vi "COD主界面（列队使用）.vi"() -> (8 "多列列表框":i32(listbox))   [LabVIEW 2016, in "斯坦道CODMn.lvlib"]
uses:
  <vilib>/Utility/miscctls.llb/LVPointTypeDef.ctl
  <vilib>/Analysis/6fits.llb/Curve Fitting Criteria.ctl
  <vilib>/Plasmionique/MB Master/MB_Master_Serial/MB_Master_Serial.lvclass
  D:/Program Files (x86)/National Instruments/LabVIEW 2016/vi.lib/Plasmionique/MB Master/MB_Master/MB_Master.lvclass
  <vilib>/Utility/config.llb/Write Key (Double).vi
  <vilib>/Utility/config.llb/Read Key (I32).vi
  <vilib>/Utility/config.llb/Read Key (Double).vi
  <vilib>/Utility/config.llb/Read Key (Boolean).vi
  <vilib>/Utility/config.llb/Write Key (Boolean).vi
  <vilib>/Utility/config.llb/Write Key (I32).vi
  <vilib>/Waveform/WDTFileIO.llb/Read Waveform from File.vi
  <vilib>/Plasmionique/MB Master/MB Master.lvlib
  <vilib>/ptbypt/NI_PtbyPt.lvlib
  <vilib>/Utility/config.llb/NI_LVConfig.lvlib
  <vilib>/Analysis/NI_AALPro.lvlib
panel:
  out "ORP-K":string
  out "ORP-B":string
  out "ORP-A":string
  out "x = y?":bool
  out "稀释倍数解释":string
  in  "CODMn跨度量程选择":enum32{"H", "L", "AUTO"}(ring)=enum."AUTO"
  in  "跨度液浓度":dbl
  in  "水样":dbl
  in  "蒸馏水":dbl
  in  "标液":dbl
  in  "质控样":dbl
  in  "加标回收":dbl
  in  "草酸钠":dbl
  in  "高锰酸钾":dbl
  in  "硫酸":dbl
  out "量程解释说明":string
  in  "高切低阈值:":dbl
  in  "低切高阈值:":dbl
  in  "自动切换量程:":enum16{"关闭", "自动切换测一次", "自动切换测两次"}(ring)
  in  "修正系数":dbl
  in  "标准液浓度":dbl
  in  "温度":dbl
  in  "恒温时间":dbl
  in  "基本量程":enum16{"L", "H"}(ring)
  in  "CODMn零点核查选择":enum16{"零点核查走纯水管", "零点核查走质控管"}(ring)
  in  "锁定按钮":bool
  in  "低量程稀释倍数:":i8=1
  out "切换量程连续测两次":bool
  in  "高量程稀释倍数:":i8=2
  in  "一键写入":bool
  in  "测量模式(公式)":u16(ring)=1 items=["水样测试"=1, "标样核查"=2, "零点核查"=3, "跨度核查"=4, "空白测试"=5, "平行样"=6, "加标回收"=7]
  out "基本量程(显示)":string
  out "测量模式(显示)":string
  in  "量程切换次数":u8
  out "数据时间":string
  out "断电排液标记":bool
  in  "测量模式":T1(ring)
  out "COM":string
  in  "启用5":bool
  in  "校准5":bool
  in  "泵滴定数5":dbl
  in  "浓度5":dbl
  in  "启用4":bool
  in  "校准4":bool
  in  "泵滴定数4":dbl
  in  "浓度4":dbl
  out "波形时间":timestamp
  in  "历史波形":bool
  out "滴定数-ORP值":u16[](array[numeric]) caption="数组"
  in  "关闭 3":bool
  in  "滴定曲线":bool
  out "ORP滴定曲线":u16[](graph)
  out "空白测试标记":bool
  out "跨度核查标记":bool
  out "启动选择 2":u16(ring) items=["水样测试", "标样核查", "零点核查", "跨度核查", "空白测试", "加标回收", "平行样", "校零", "校标"]
  in  "量程选择":enum16{"低量程", "高量程", "0-2量程"}(ring)
  in  "手动控制":bool
  in  "选用水样":enum16{"葡萄糖", "草酸钠"}(ring)
  in  "方程系数":cluster{"X":dbl, "b":dbl, "X^2":dbl} {"X^2" format="%#.6g"; "b" format="%#.6g"; "X" format="%#.6g"}
  out "多项式系数1":dbl[](array[numeric]) caption="多项式系数"
  out "XY图":cluster{"X Values":dbl[], "Y Values":dbl[]}[](graph)
  in  "模型":enum32{"线性", "多项式"}(ring)
  out "启动时间":timestamp format="%<%Y/%m/%d %H:%M:%S>T"
  in  "24H周期设置":bool[](xcontrol)
  in  "关闭 2":bool
  in  "周期设置":bool
  out "文本.文本":string
  out "r^2":dbl format="%.8g"
  out "拟合公式":string
  out "b":dbl format="%#.4g"
  out "K":dbl format="%#.4f"
  out "当前校准":i32
  in  "启用3":bool
  in  "启用2":bool
  in  "启用1":bool
  in  "校准3":bool
  in  "校准2":bool
  in  "校准1":bool
  in  "泵滴定数3":dbl
  in  "泵滴定数2":dbl
  in  "泵滴定数1":dbl
  in  "浓度3":dbl
  in  "浓度2":dbl
  in  "浓度1":dbl
  in  "写入":bool
  out "测量模式数字":i32
  out "零点核查标记":bool
  out "排液故障":bool
  out "进水样超量程":bool
  out "标样核查标记":bool
  out "平行样测量":bool
  out "加标回收测量":bool
  out "质控样测量":bool
  out "待机":bool
  out "校标错误":bool
  out "校零错误":bool
  out "测量错误":bool
  out "草酸钠报警":bool
  out "高锰酸钾报警":bool
  out "加热故障":bool
  out "温控器故障":bool
  out "ORP故障":bool
  out "排液标记":bool
  out "故障标记":bool
  out "校标标记":bool
  out "校零标记":bool
  out "通讯状态":bool
  out "水样测量":bool
  out "读取KB值":bool
  in  "读取":bool
  in  "返回":bool
  in  "校准配置":bool
  in  "零点泵计量数 2":dbl
  in  "标度泵计量数 2":dbl
  out "标度滴定值":dbl
  out "零点滴定值":dbl
  in  "保存":bool
  in  "关闭":bool
  out "测量数据区":T2 {"单位" items=["ug/L", "mg/L", "ppm", "mg/m3", "cm", "ppb", "ug/m3", "%", "nmol/mol", "umol/mol", "MPN/L", "MPN/100ml", "ng/m3", "NTU", "无量纲", "ms/cm", "us/cm", "℃", "mV", "万个/L"]}
  out "仪器时间":timestamp format="%<%Y/%m/%d %H:%M:%S>T"
  out "秒":u16
  out "分":u16
  out "COD浓度（mg/L)":dbl format="%.2g"
  out "进样管":dbl
  out "高锰酸钾":dbl
  out "草酸钠":dbl
  out "硫酸":dbl
  out "ORP显示":dbl
  out "温度":dbl
  out "加热":bool
  out "搅拌":bool
  out "进硫酸":bool
  out "进加标回收样":bool
  out "进质控样":bool
  out "进标液":bool
  out "进蒸馏水":bool
  out "进水样":bool
  out "进草酸钠":bool
  out "进高锰酸钾":bool
  out "定时启动":bool
  in  "启动":bool
  in  "故障清除":bool
  in  "参数配置":bool
  in  "停止":bool
  in  "单步启动":bool
  out "系统时间":timestamp
  in  "时间校准":bool
  in  "枚举":enum16{"读取数据", "写入数据", "读取写入DATABASE", "读取参数"}(ring)
  out "报警簇":T3
  out "Registers":u16[](array[numeric])
  in  "Slave ID":u8=1
  in  "Serial Config":T4={"baud rate (bps)"=115200, "stop bits"=10, "parity"=0, "flow control"=0, "timeout"=1000, "retries"=1} {"stop bits" items=["1.0"=10, "1.5"=15, "2.0"=20]; "flow control" items=["None", "XON/XOFF", "RTS/CTS", "XON/XOFF & RTS/CTS", "DTR/DSR", "XON/XOFF & DTR/DSR"]; "parity" items=["None", "Odd", "Even", "Mark", "Space"]}
  out "模式（受控）":u16
  in  "VISA resource name":refnum<visa-resource-name>="COM4" caption="VISA资源名称"
  # "测量时间："
  # "(水样~加标回收)"
  # "mV"
  # "℃"
  # "注：遇到加热故障和排液故障时仪器不能正常启动，\n必须排查故障并点击报警清除按钮方可运行。"
  # "mg/L"
  # "泵计量参数设置"
  # "基本参数设置"
  # "校零校标结果"
  # "校零结果："
  # "校零滴定值："
  # "加热恒温温度(℃):"
  # "水样："
  # "高锰酸钾："
  # "校标结果："
  # "标度滴定值："
  # "恒温时间(分钟):"
  # "草酸钠："
  # "蒸馏水："
  # "零点泵计量值："
  # "标准液浓度(mg/L):"
  # "硫酸："
  # "标液："
  # "标度泵计量值："
  # "修正系数："
  # "跨度液浓度："
  # "质控样:"
  # "基本量程(L、H)可选:"
  # "跨度量程选择："
  # "加标回收样："
  # "是否启用"
  # "泵滴定数"
  # "浓度"
  # "辅\n助\n计\n算\n区"
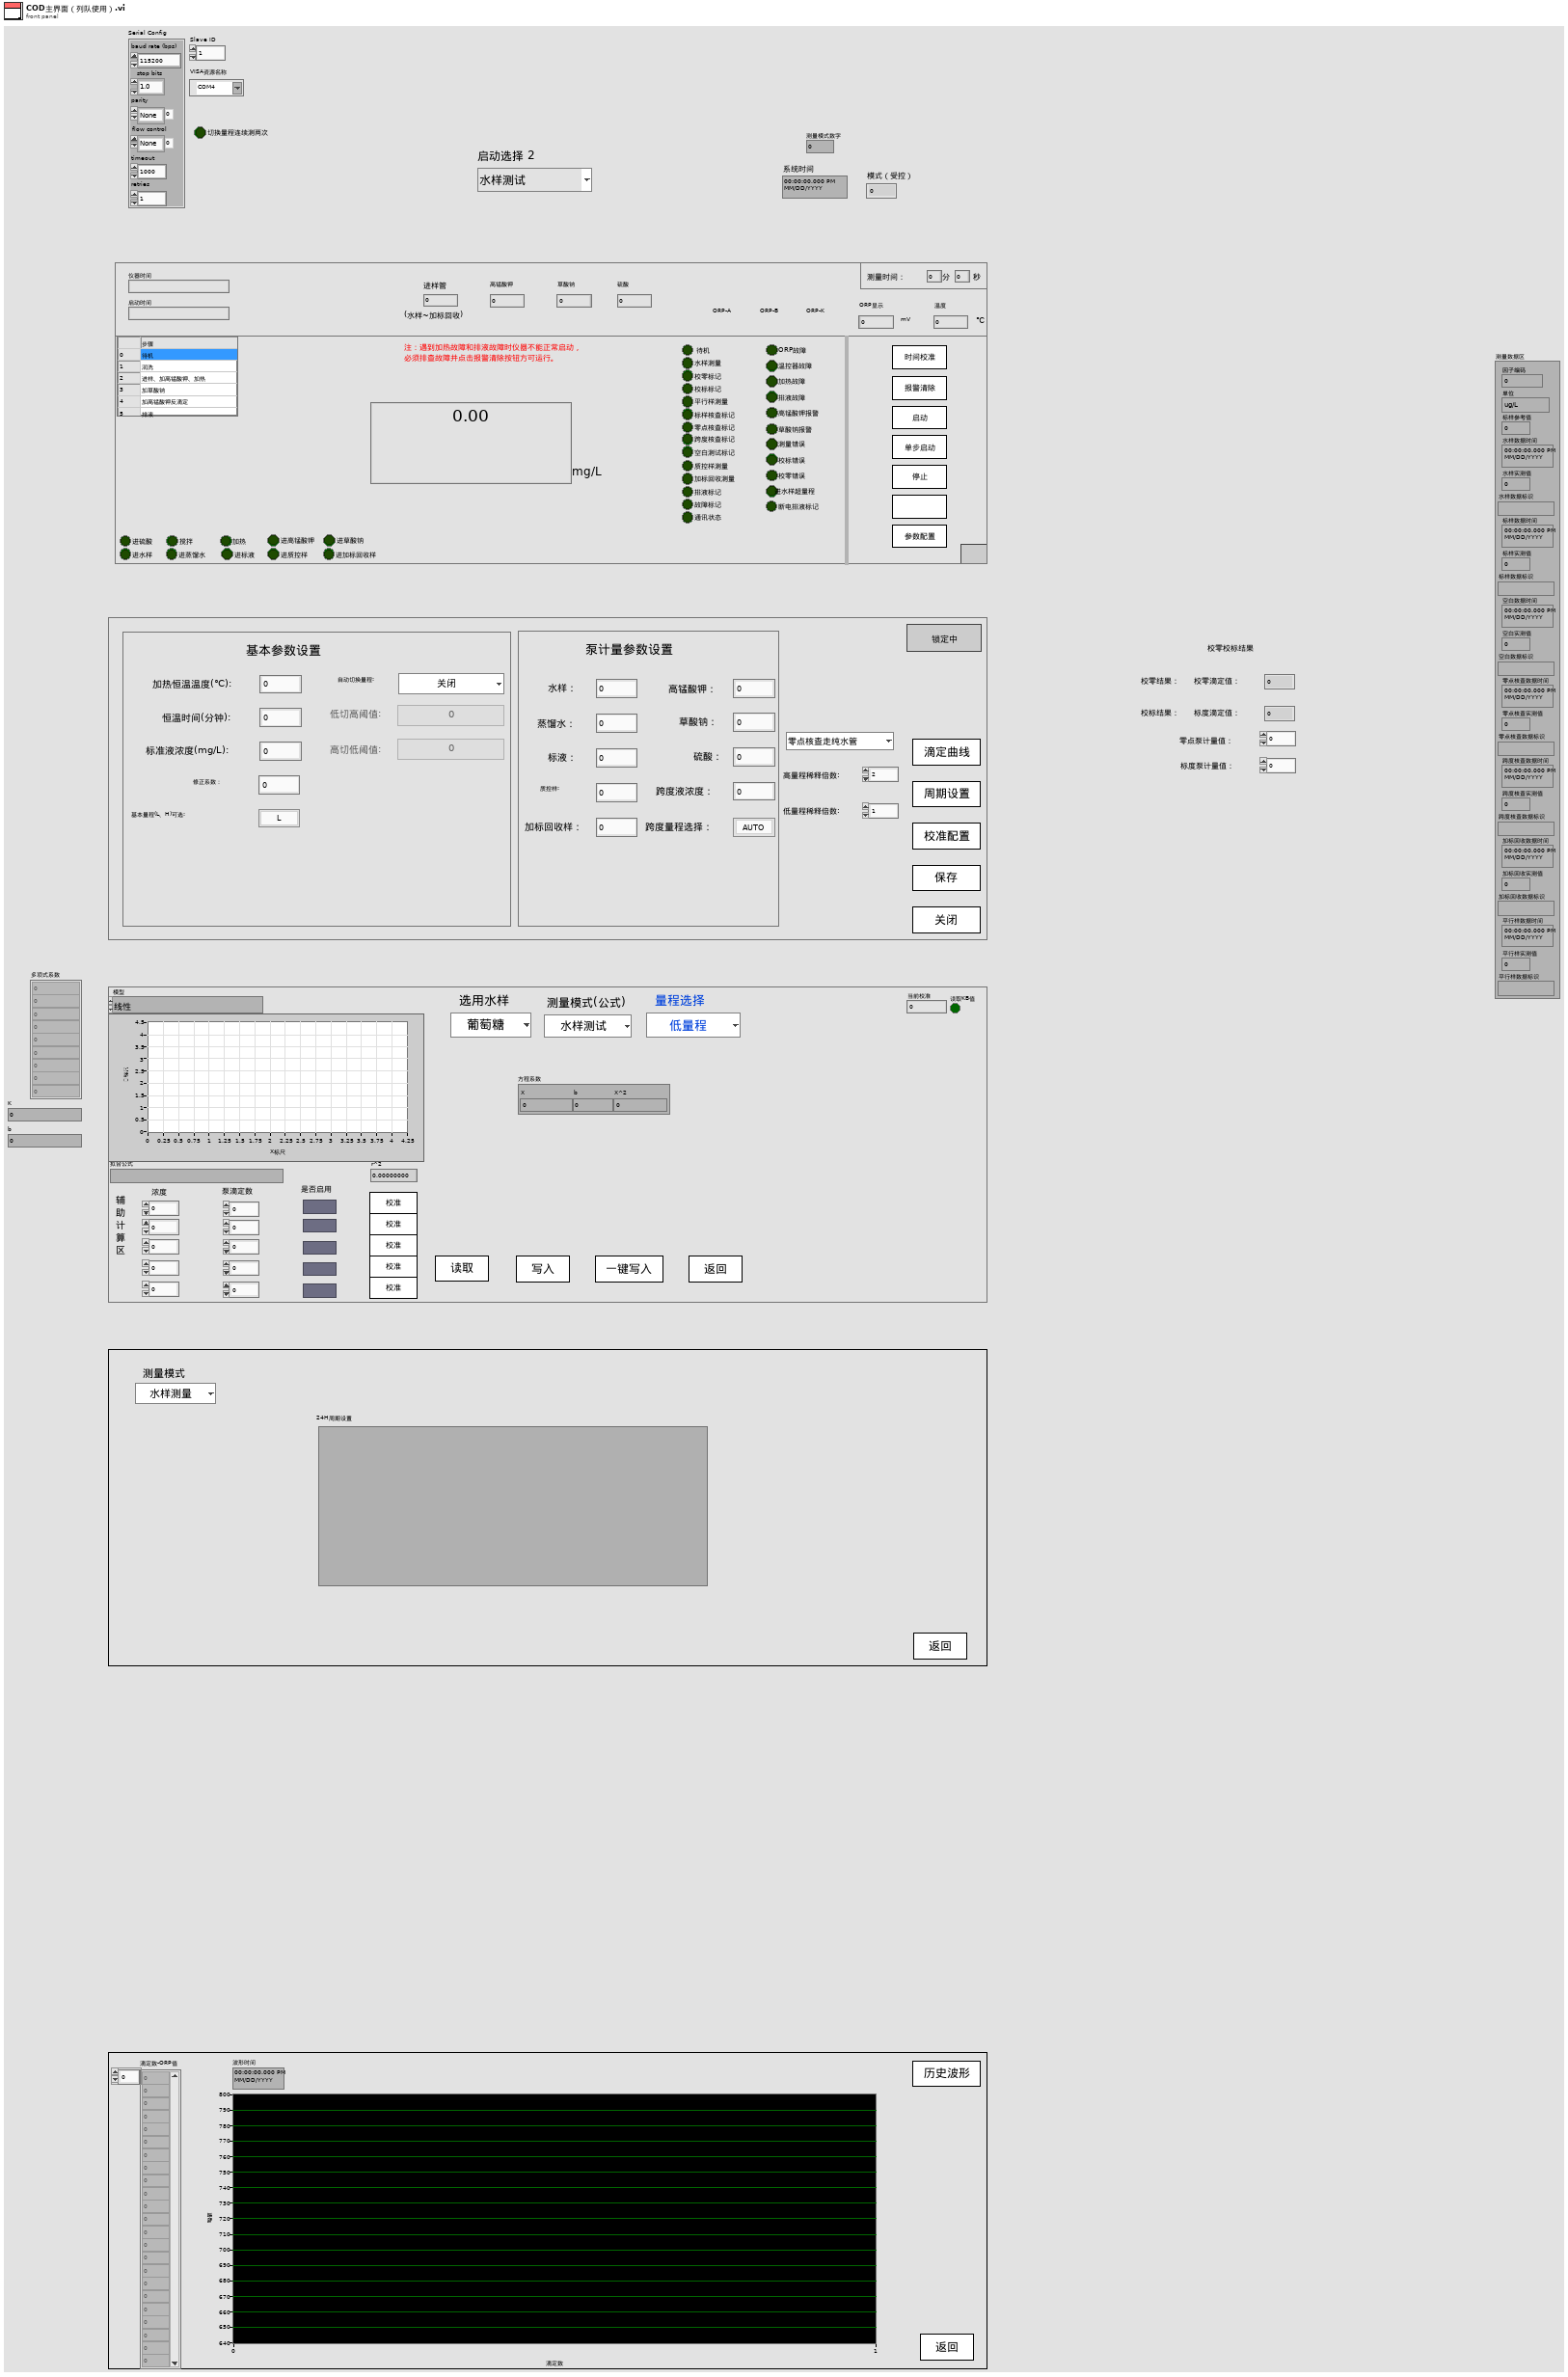
[diagram p1: front panel]
types:
  T1 = enum16{"水样测量", "标样核查", "零点核查", "跨度核查", "空白测试", "加标回收", "平行样", "校零", "校标"}
  T2 = cluster{"因子编码":u32, "单位":u16, "标样参考值":sgl, "水样数据时间":timestamp, "水样实测值":sgl, "水样数据标识":string, "标样数据时间":timestamp, "标样实测值":sgl, "标样数据标识":string, "空白数据时间":timestamp, "空白实测值":sgl, "空白数据标识":string, "零点核查数据时间":timestamp, "零点核查实测值":sgl, "零点核查数据标识":string, "跨度核查数据时间":timestamp, "跨度核查实测值":sgl, "跨度核查数据标识":string, "加标回收数据时间":timestamp, "加标回收实测值":sgl, "加标回收数据标识":string, "平行样数据时间":timestamp, "平行样实测值":sgl, "平行样数据标识":string}
  T3 = cluster{"ORP故障":bool, "温控器故障":bool, "加热故障":bool, "高锰酸钾报警":bool, "草酸钠报警":bool, "测量错误":bool, "校零错误":bool, "校标错误":bool, " 进水样超量程":bool, "排液阀故障":bool}
  T4 = cluster{"baud rate (bps)":u32, "stop bits":u16, "parity":u16, "flow control":u16, "timeout":u32, "retries":i32}
  T5 = cluster{"starting address":u16, "number of holding registers":u16}
  T6 = typedef "NI_LVConfig.lvlib/Config Data RefNum.ctl" = refnum<k1>
  T7 = cluster{"测量模式":enum16{"水样测量", "标样核查", "零点核查", "跨度核查", "空白测试", "加标回收", "平行样", "校零", "校标"}}
  T8 = cluster{"仪器测试类型":enum16{"水样测试", "标样核查", "空白测试", "跨度核查"}, "周期设置类型":enum16{"定点启动", "间隔启动"}, "定时功能启用":bool, "定时间隔":dbl, "24H周期设置":bool[]}
  T9 = typedef "LVDateTimeRec.ctl" = cluster{"秒数的小数部分":dbl, "秒":i32, "分":i32, "时":i32, "日":i32, "月":i32, "年":i32, "天数（周）":i32, "天数（年）":i32, "DST":i32}
  T10 = enum8{"Enabled", "Disabled", "Disabled and Grayed Out"}
  T11 = typedef "NI_AALPro.lvlib/Curve Fitting Criteria.ctl" = u16
  T12 = cluster{"时间":timestamp, "测量模式":string, "数据类型":string, "检测值":sgl, "单位":string, "数据标识":string, "因子编码":string, "标样参考值":sgl, "ORP-A":sgl, "ORP-B":sgl, "ORP-K":sgl, "COD滴定值":sgl, "高锰酸钾滴定数":sgl, "温度":sgl, "量程":sgl}
  T13 = typedef "LVPointTypeDef.ctl" = cluster{"Horizontal":i16, "Vertical":i16}
  T14 = cluster{"时间标识":timestamp, "参数":string, "日志信息":string, "流程参数":string}
  T15 = cluster{"时间标识":timestamp, "设备":string, "日志信息":string}
  T16 = cluster{"时间标识":timestamp, "设备":string, "日志信息":string, "流程参数":string}
  T17 = cluster{"运行模式":enum16{"维护模式", "常规模式", "应急模式", "质控模式"}}
  T18 = cluster{"数组 2[0]":sgl, "数组 2[1]":sgl, "数组 2[2]":sgl, "数组 2[3]":sgl, "数组 2[4]":sgl, "数组 2[5]":sgl, "数组 2[6]":sgl, "数组 2[7]":sgl, "数组 2[8]":sgl, "数组 2[9]":sgl, "数组 2[10]":sgl, "数组 2[11]":sgl, "数组 2[12]":sgl, "数组 2[13]":sgl, "数组 2[14]":sgl, "数组 2[15]":sgl, "数组 2[16]":sgl, "数组 2[17]":sgl, "数组 2[18]":sgl, "数组 2[19]":sgl, "数组 2[20]":sgl, "数组 2[21]":sgl, "数组 2[22]":sgl, "数组 2[23]":sgl, "数组 2[24]":sgl, "数组 2[25]":sgl, "数组 2[26]":sgl, "数组 2[27]":sgl, "数组 2[28]":sgl, "数组 2[29]":sgl, "数组 2[30]":sgl, "数组 2[31]":sgl, "数组 2[32]":sgl, "数组 2[33]":sgl, "数组 2[34]":sgl, "数组 2[35]":sgl, "数组 2[36]":sgl, "数组 2[37]":sgl, "数组 2[38]":sgl, "数组 2[39]":sgl, "数组 2[40]":sgl, "数组 2[41]":sgl}
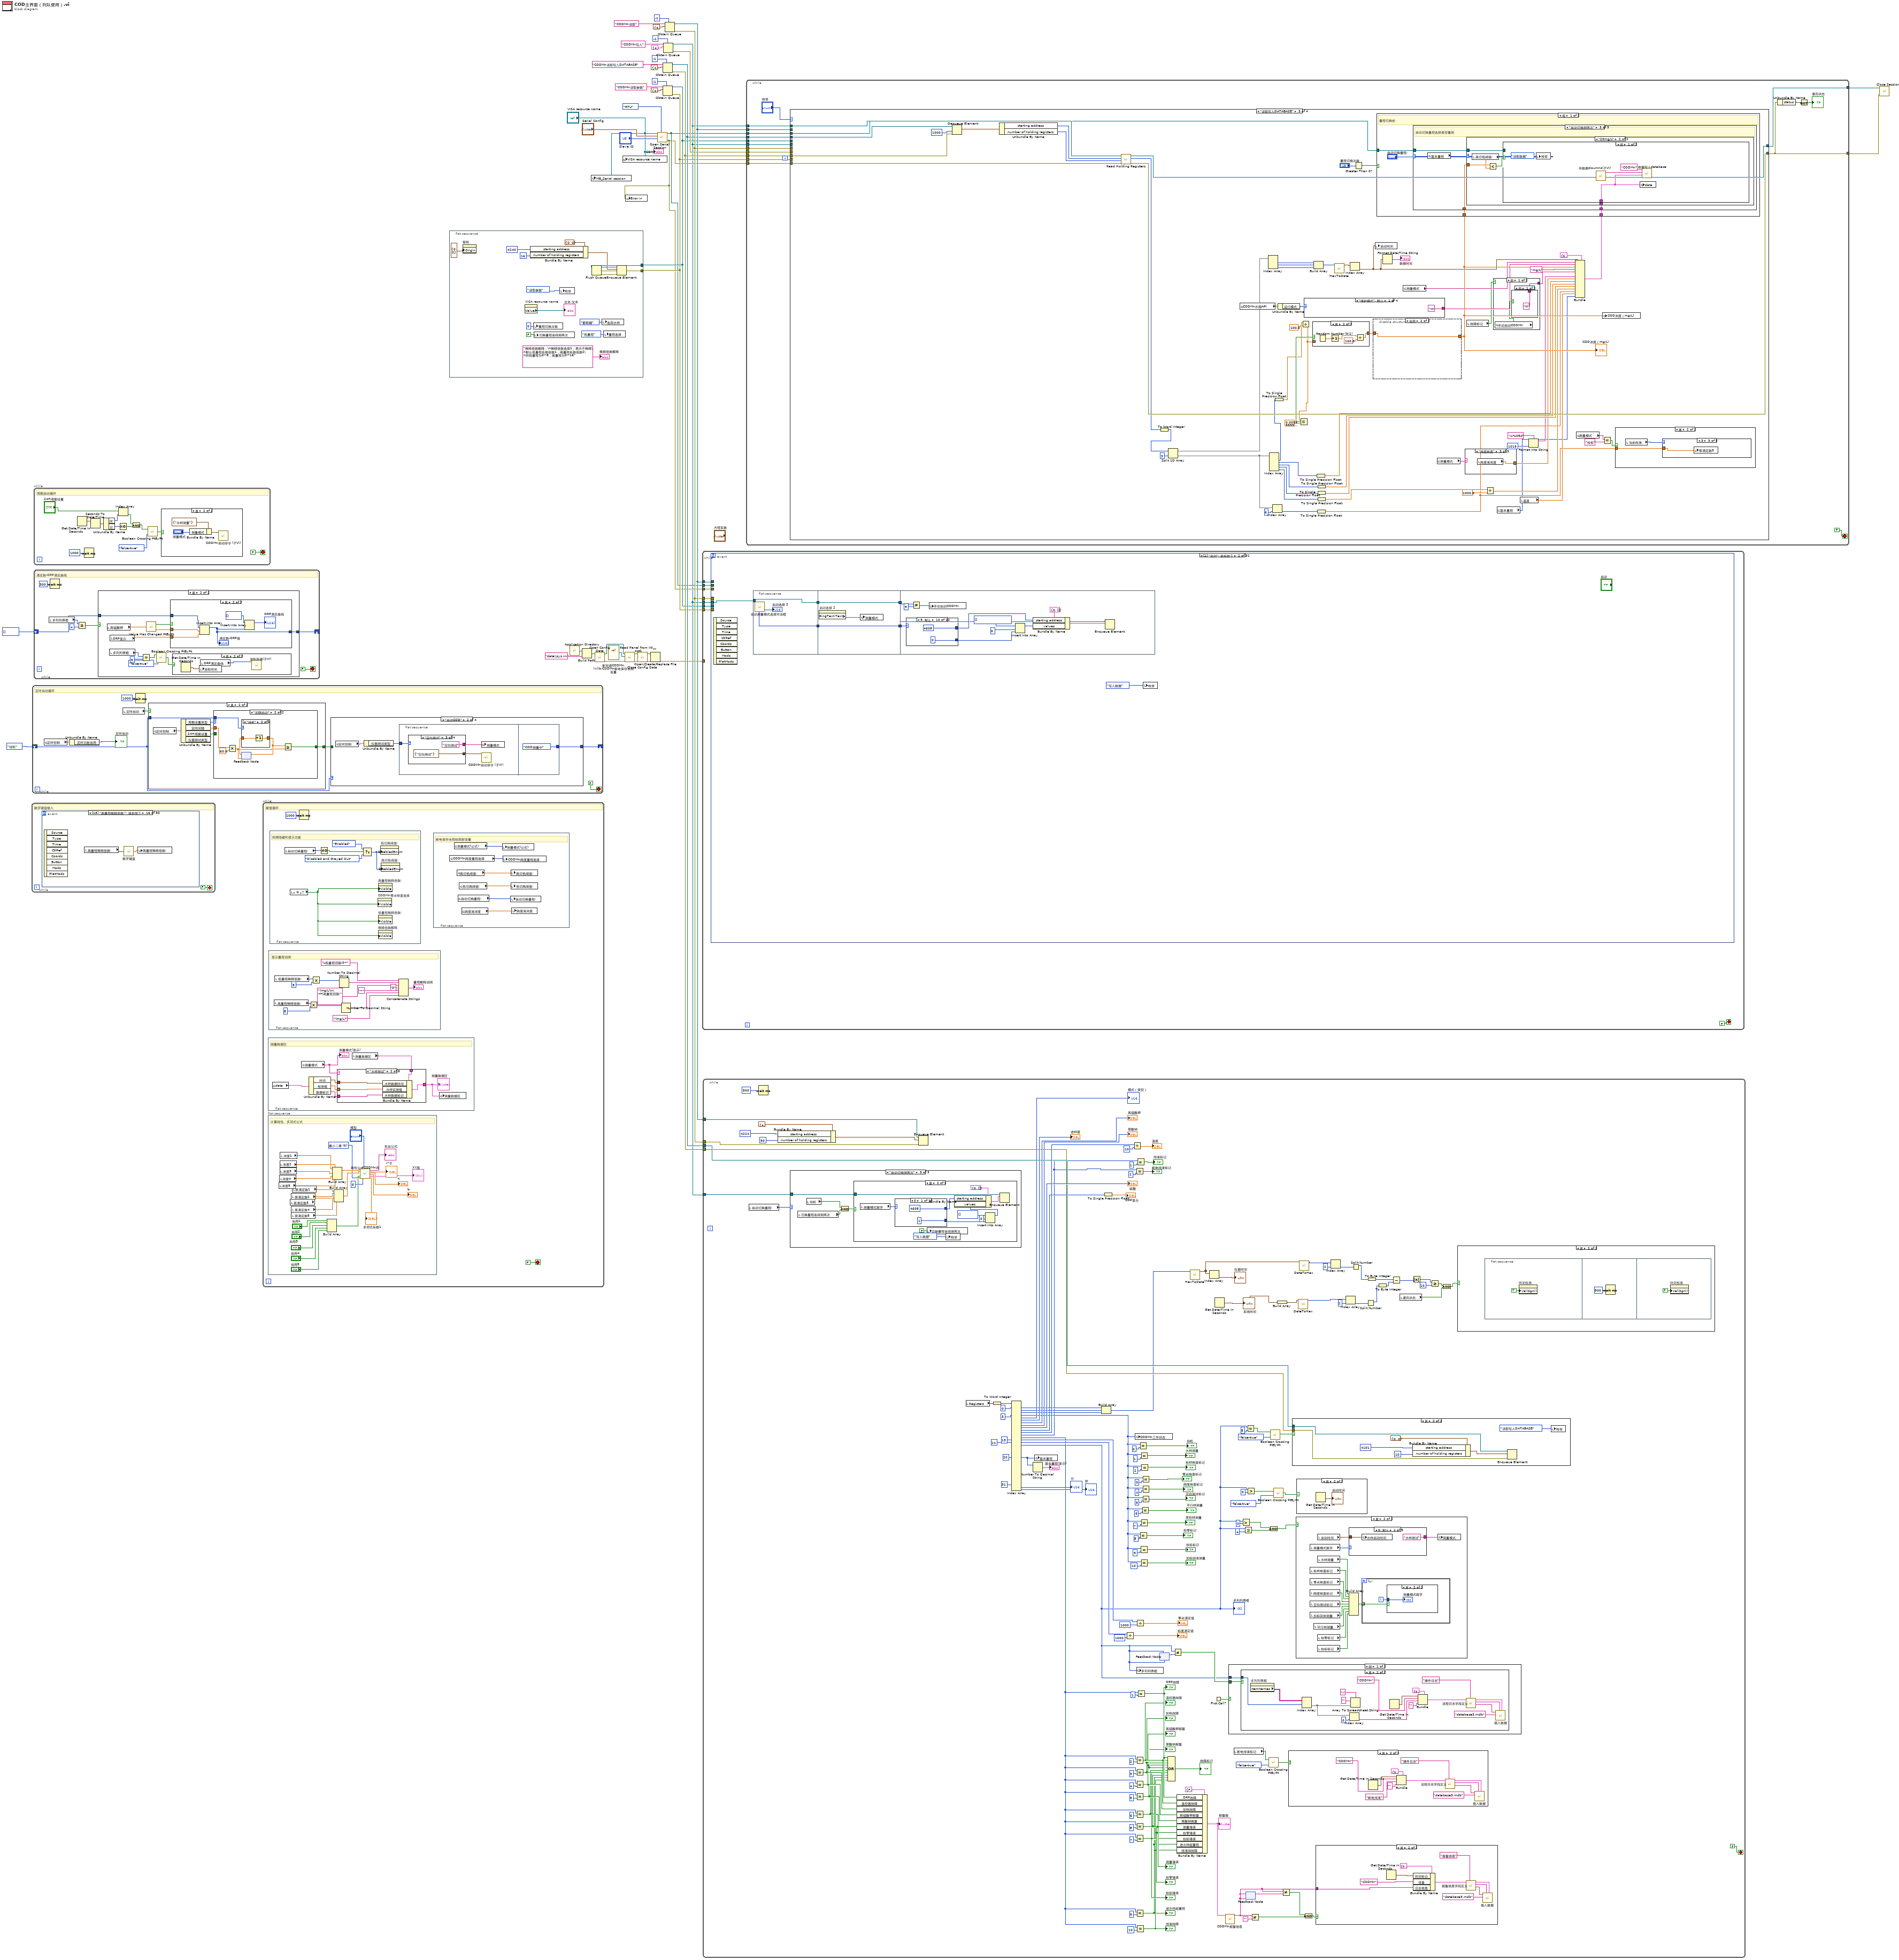
[diagram p0: block diagram]
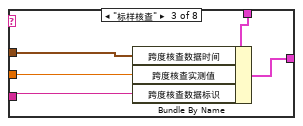
[diagram p3: hidden frame]
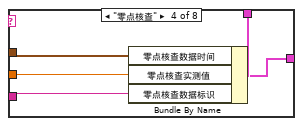
[diagram p4: hidden frame]
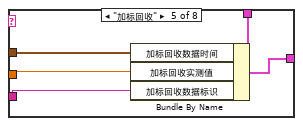
[diagram p5: hidden frame]
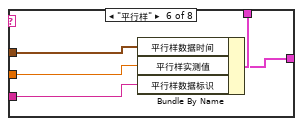
[diagram p6: hidden frame]
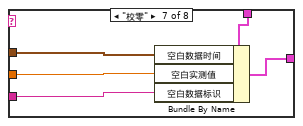
[diagram p7: hidden frame]
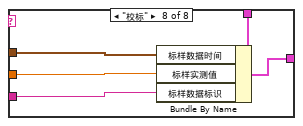
[diagram p8: hidden frame]
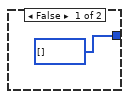
[diagram p9: hidden frame]
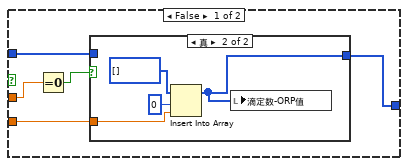
[diagram p11: hidden frame]
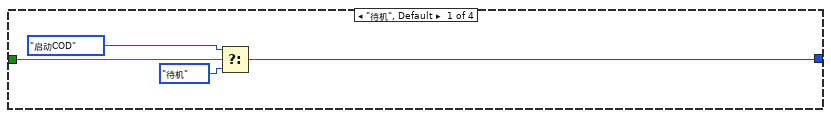
[diagram p14: hidden frame]
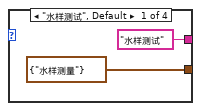
[diagram p15: hidden frame]
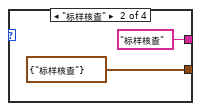
[diagram p16: hidden frame]
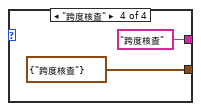
[diagram p17: hidden frame]
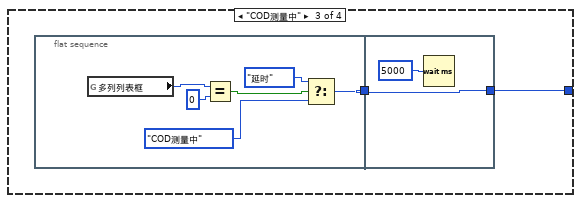
[diagram p18: hidden frame]
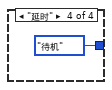
[diagram p19: hidden frame]
diagram:
  n1 = while {
    stop <- FALSE stop-if-true
    # "数字键盘输入"
    n2 = event shown="[15] \"高量程稀释倍数:\": 鼠标按下" {
      selector: _ -> [_ _ _ _ _ _ _ _ _ _ _ _ _ _ _ _ _ _ _ _ _ _ _ _ _ _ _ _ _ _]
      dyn-events: _ -> [_ _ _ _ _ _ _ _ _ _ _ _ _ _ _ _ _ _ _ _ _ _ _ _ _ _ _ _ _ _]
      timeout: _ -> [_ _ _ _ _ _ _ _ _ _ _ _ _ _ _ _ _ _ _ _ _ _ _ _ _ _ _ _ _ _]
      event Timeout {
        n3 = event-data() -> ()  [unwired: 1 in, 3 out]
      }
      event "温度": Mouse Down {
        n4 = event-data() -> ()  [unwired: 1 in, 8 out]
        n5 = local read "温度"() -> (w44:dbl)
        n6 = call "数字键盘.vi"("OldNumber"=w44) -> ("NewNumber"=w43:sgl)
        n7 = local write "温度"(w43) -> ()
      }
      event "恒温时间": Mouse Down {
        n8 = event-data() -> ()  [unwired: 1 in, 8 out]
        n9 = local read "恒温时间"() -> (w45:dbl)
        n10 = call "数字键盘.vi"("OldNumber"=w45) -> ("NewNumber"=w46:sgl)
        n11 = local write "恒温时间"(w46) -> ()
      }
      event "标准液浓度": Mouse Down {
        n12 = event-data() -> ()  [unwired: 1 in, 8 out]
        n13 = local read "标准液浓度"() -> (w48:dbl)
        n14 = call "数字键盘.vi"("OldNumber"=w48) -> ("NewNumber"=w47:sgl)
        n15 = local write "标准液浓度"(w47) -> ()
      }
      event "修正系数": Mouse Down {
        n16 = event-data() -> ()  [unwired: 1 in, 8 out]
        n17 = local read "修正系数"() -> (w49:dbl)
        n18 = call "数字键盘.vi"("OldNumber"=w49) -> ("NewNumber"=w50:sgl)
        n19 = local write "修正系数"(w50) -> ()
      }
      event "水样": Mouse Down {
        n20 = event-data() -> ()  [unwired: 1 in, 8 out]
        n21 = local read "水样"() -> (w51:dbl)
        n22 = call "数字键盘.vi"("OldNumber"=w51) -> ("NewNumber"=w52:sgl)
        n23 = local write "水样"(w52) -> ()
      }
      event "蒸馏水": Mouse Down {
        n24 = event-data() -> ()  [unwired: 1 in, 8 out]
        n25 = local read "蒸馏水"() -> (w53:dbl)
        n26 = call "数字键盘.vi"("OldNumber"=w53) -> ("NewNumber"=w54:sgl)
        n27 = local write "蒸馏水"(w54) -> ()
      }
      event "标液": Mouse Down {
        n28 = event-data() -> ()  [unwired: 1 in, 8 out]
        n29 = local read "标液"() -> (w55:dbl)
        n30 = call "数字键盘.vi"("OldNumber"=w55) -> ("NewNumber"=w56:sgl)
        n31 = local write "标液"(w56) -> ()
      }
      event "质控样": Mouse Down {
        n32 = event-data() -> ()  [unwired: 1 in, 8 out]
        n33 = local read "质控样"() -> (w57:dbl)
        n34 = call "数字键盘.vi"("OldNumber"=w57) -> ("NewNumber"=w58:sgl)
        n35 = local write "质控样"(w58) -> ()
      }
      event "加标回收": Mouse Down {
        n36 = event-data() -> ()  [unwired: 1 in, 8 out]
        n37 = local read "加标回收"() -> (w59:dbl)
        n38 = call "数字键盘.vi"("OldNumber"=w59) -> ("NewNumber"=w60:sgl)
        n39 = local write "加标回收"(w60) -> ()
      }
      event "草酸钠": Mouse Down {
        n40 = event-data() -> ()  [unwired: 1 in, 8 out]
        n41 = local read "草酸钠"() -> (w61:dbl)
        n42 = call "数字键盘.vi"("OldNumber"=w61) -> ("NewNumber"=w62:sgl)
        n43 = local write "草酸钠"(w62) -> ()
      }
      event "高锰酸钾": Mouse Down {
        n44 = event-data() -> ()  [unwired: 1 in, 8 out]
        n45 = local read "高锰酸钾"() -> (w63:dbl)
        n46 = call "数字键盘.vi"("OldNumber"=w63) -> ("NewNumber"=w64:sgl)
        n47 = local write "高锰酸钾"(w64) -> ()
      }
      event "硫酸": Mouse Down {
        n48 = event-data() -> ()  [unwired: 1 in, 8 out]
        n49 = local read "硫酸"() -> (w65:dbl)
        n50 = call "数字键盘.vi"("OldNumber"=w65) -> ("NewNumber"=w66:sgl)
        n51 = local write "硫酸"(w66) -> ()
      }
      event "零点泵计量数 2": Mouse Down {
        n52 = event-data() -> ()  [unwired: 1 in, 8 out]
        n53 = local read "零点泵计量数 2"() -> (w67:dbl)
        n54 = call "数字键盘.vi"("OldNumber"=w67) -> ("NewNumber"=w68:sgl)
        n55 = local write "零点泵计量数 2"(w68) -> ()
      }
      event "标度泵计量数 2": Mouse Down {
        n56 = event-data() -> ()  [unwired: 1 in, 8 out]
        n57 = local read "标度泵计量数 2"() -> (w69:dbl)
        n58 = call "数字键盘.vi"("OldNumber"=w69) -> ("NewNumber"=w70:sgl)
        n59 = local write "标度泵计量数 2"(w70) -> ()
      }
      event "高量程稀释倍数:": Mouse Down {
        n60 = event-data() -> ()  [unwired: 1 in, 8 out]
        n61 = local read "高量程稀释倍数:"() -> (w72:i8)
        n62 = call "数字键盘.vi"("OldNumber"=w72) -> ("NewNumber"=w71:sgl)
        n63 = local write "高量程稀释倍数:"(w71) -> ()
      }
      event "低量程稀释倍数:": Mouse Down {
        n64 = event-data() -> ()  [unwired: 1 in, 8 out]
        n65 = local read "低量程稀释倍数:"() -> (w74:i8)
        n66 = call "数字键盘.vi"("OldNumber"=w74) -> ("NewNumber"=w73:sgl)
        n67 = local write "低量程稀释倍数:"(w73) -> ()
      }
      event "浓度1": Mouse Down {
        n68 = event-data() -> ()  [unwired: 1 in, 8 out]
        n69 = local read "浓度1"() -> (w76:dbl)
        n70 = call "数字键盘.vi"("OldNumber"=w76) -> ("NewNumber"=w75:sgl)
        n71 = property on="浓度1" class="DigNum (严格)"("Val(Sgnl)"=w75) -> ()  [unwired: 2 in, 2 out]
      }
      event "浓度2": Mouse Down {
        n72 = event-data() -> ()  [unwired: 1 in, 8 out]
        n73 = local read "浓度2"() -> (w78:dbl)
        n74 = call "数字键盘.vi"("OldNumber"=w78) -> ("NewNumber"=w77:sgl)
        n75 = property on="浓度2" class="DigNum (严格)"("Val(Sgnl)"=w77) -> ()  [unwired: 2 in, 2 out]
      }
      event "浓度3": Mouse Down {
        n76 = event-data() -> ()  [unwired: 1 in, 8 out]
        n77 = local read "浓度3"() -> (w80:dbl)
        n78 = call "数字键盘.vi"("OldNumber"=w80) -> ("NewNumber"=w79:sgl)
        n79 = property on="浓度3" class="DigNum (严格)"("Val(Sgnl)"=w79) -> ()  [unwired: 2 in, 2 out]
      }
      event "浓度4": Mouse Down {
        n80 = event-data() -> ()  [unwired: 1 in, 8 out]
        n81 = local read "浓度4"() -> (w82:dbl)
        n82 = call "数字键盘.vi"("OldNumber"=w82) -> ("NewNumber"=w81:sgl)
        n83 = property on="浓度4" class="DigNum (严格)"("Val(Sgnl)"=w81) -> ()  [unwired: 2 in, 2 out]
      }
      event "浓度5": Mouse Down {
        n84 = event-data() -> ()  [unwired: 1 in, 8 out]
        n85 = local read "浓度5"() -> (w84:dbl)
        n86 = call "数字键盘.vi"("OldNumber"=w84) -> ("NewNumber"=w83:sgl)
        n87 = property on="浓度5" class="DigNum (严格)"("Val(Sgnl)"=w83) -> ()  [unwired: 2 in, 2 out]
      }
      event "跨度液浓度": Mouse Down {
        n88 = event-data() -> ()  [unwired: 1 in, 8 out]
        n89 = local read "跨度液浓度"() -> (w86:dbl)
        n90 = call "数字键盘.vi"("OldNumber"=w86) -> ("NewNumber"=w85:sgl)
        n91 = property on="跨度液浓度" class="DigNum (严格)"("Val(Sgnl)"=w85) -> ()  [unwired: 2 in, 2 out]
      }
      event "跨度液浓度": Value Change {
        n92 = event-data() -> ()  [unwired: 1 in, 6 out]
        n93 = call <vilib>:"Application Directory.vi"() -> ("Application Directory"=w90:path)
        n94 = Build Path(base path=w90, name or relative path="data\\Set.ini" ("名称或相对路径")) -> (appended path=w92:path)
        n95 = local read "跨度液浓度"() -> (w87:dbl)
        n96 = call <vilib>:"Open Config Data.vi"("configuration file path"=w92) -> ("error out"=w94:errorcluster, "refnum"=w93:T6)  [unwired: 8 in, 1 out]
        n97 = call-poly <vilib>:"Write Key.vi"("section"="CODMn参数" ("key"), "error in (no error)"=w94, "value"=w87, "key"="跨度液浓度", "refnum"=w93) -> ("error out"=w96:errorcluster, "refnum out"=w95:T6)  [unwired: 4 in, 1 out]
        n98 = call <vilib>:"Close Config Data.vi"("error in (no error)"=w96, "refnum"=w95) -> ()  [unwired: 8 in, 2 out]
      }
      event "泵滴定数1": Mouse Down {
        n99 = event-data() -> ()  [unwired: 1 in, 8 out]
        n100 = local read "泵滴定数1"() -> (w98:dbl)
        n101 = call "数字键盘.vi"("OldNumber"=w98) -> ("NewNumber"=w97:sgl)
        n102 = property on="泵滴定数1" class="DigNum (严格)"("Val(Sgnl)"=w97) -> ()  [unwired: 2 in, 2 out]
      }
      event "泵滴定数2": Mouse Down {
        n103 = event-data() -> ()  [unwired: 1 in, 8 out]
        n104 = local read "泵滴定数2"() -> (w100:dbl)
        n105 = call "数字键盘.vi"("OldNumber"=w100) -> ("NewNumber"=w99:sgl)
        n106 = property on="泵滴定数2" class="DigNum (严格)"("Val(Sgnl)"=w99) -> ()  [unwired: 2 in, 2 out]
      }
      event "泵滴定数3": Mouse Down {
        n107 = event-data() -> ()  [unwired: 1 in, 8 out]
        n108 = local read "泵滴定数3"() -> (w102:dbl)
        n109 = call "数字键盘.vi"("OldNumber"=w102) -> ("NewNumber"=w101:sgl)
        n110 = property on="泵滴定数3" class="DigNum (严格)"("Val(Sgnl)"=w101) -> ()  [unwired: 2 in, 2 out]
      }
      event "泵滴定数4": Mouse Down {
        n111 = event-data() -> ()  [unwired: 1 in, 8 out]
        n112 = local read "泵滴定数4"() -> (w104:dbl)
        n113 = call "数字键盘.vi"("OldNumber"=w104) -> ("NewNumber"=w103:sgl)
        n114 = property on="泵滴定数4" class="DigNum (严格)"("Val(Sgnl)"=w103) -> ()  [unwired: 2 in, 2 out]
      }
      event "泵滴定数5": Mouse Down {
        n115 = event-data() -> ()  [unwired: 1 in, 8 out]
        n116 = local read "泵滴定数5"() -> (w106:dbl)
        n117 = call "数字键盘.vi"("OldNumber"=w106) -> ("NewNumber"=w105:sgl)
        n118 = property on="泵滴定数5" class="DigNum (严格)"("Val(Sgnl)"=w105) -> ()  [unwired: 2 in, 2 out]
      }
      event "低切高阈值:", "高切低阈值:": Mouse Down {
        n119 = event-data() -> ("CtlRef"=w110:refnum<vi>)  [unwired: 1 in, 7 out]
        n120 = property class="DigNum (严格)"(reference=w110) -> (reference out=w109:refnum<vi>, "Value"=w108:dbl)  [unwired: 1 in, 1 out]
        n121 = call "数字键盘.vi"("OldNumber"=w108) -> ("NewNumber"=w107:sgl)
        n122 = property class="DigNum (严格)"(reference=w109, "Val(Sgnl)"=w107) -> ()  [unwired: 1 in, 2 out]
      }
    }
  }
  n123 = while {
    shift-right: [w116] -> _
    shift-left: enum16{"待机", "启动COD", "COD测量中", "延时"}."待机" -> [w115]
    stop <- FALSE stop-if-true
    # "定时启动循环"
    n124 = global read "CODMn断电保存全局变量.vi" "定时控制"() -> (w112:T8)
    n125 = Unbundle By Name(w112) -> ("定时功能启用"=→"定时启动":bool)
    n126 = local read "定时启动"() -> (w113:bool)
    n127 = Wait (ms)(milliseconds to wait=u32 1000 ("等待时间（毫秒）")) -> ()  [unwired: 1 out]
    n128 = case shown="真" w113 {
      tunnel: w115 -> [_ w151]
      tunnel: [_ w150] -> w114
      frame False {
      }
      frame True {
        n129 = global read "CODMn断电保存全局变量.vi" "定时控制"() -> (w149:T8)
        n130 = Unbundle By Name(w149) -> ("周期设置类型"=w152:enum16{"定点启动", "间隔启动"}, "定时间隔"=w153:dbl, "24H周期设置"=w154:bool[])  [unwired: 1 out]
        n131 = case shown="\"间隔启动\"" w152 {
          tunnel: w153 -> [_ w171]
          tunnel: w154 -> [w157 _]
          tunnel: w151 -> [w155 w174]
          tunnel: [w156 w169] -> w150
          frame "定点启动", Default {
            n132 = case shown="\"待机\", 默认" w155 {
              tunnel: w157 -> [w165 _]
              tunnel: [w158 _] -> w156
              frame "待机", Default {
                n133 = Get Date/Time In Seconds() -> (seconds since 1Jan1904=w167:timestamp)
                n134 = Seconds To Date/Time(time stamp (now)=w167) -> (date time rec=w166:T9)  [unwired: 1 in]
                n135 = Unbundle By Name(w166) -> ("时"=w164:i32, "分"=w162:i32, "秒"=w163:i32)
                n136 = Equal To 0?(x=w162) -> (x = 0?=w160:bool)
                n137 = Equal To 0?(x=w163) -> (x = 0?=w159:bool)
                n138 = Index Array(array=w165, index=w164) -> (element=w161:bool)
                n139 = Compound Arithmetic op=AND ("复合运算")(w161, w160, w159) -> (w158:bool)
              }
              frame "启动COD" {
              }
            }
          }
          frame "间隔启动" {
            n140 = Multiply(x=w171, y=60.0) -> (x*y=w168:dbl)
            n141 = feedback #1(w168) -> (w173:dbl)
            n142 = case shown="\"待机\"" w174 {
              tunnel: w173 -> [_ w176]
              tunnel: [_ w175] -> w172
              frame Default {
              }
              frame "待机" {
                n143 = Increment(x=w176) -> (x+1=w175:dbl)
              }
            }
            n144 = feedback-in #1(w172) -> ()
            n145 = Greater Or Equal?(x=w172, y=w168) -> (x >= y?=w169:bool)
          }
        }
      }
    }
    n146 = case shown="\"启动COD\"" w115 {
      tunnel: [w119 w125 w139 enum16{"待机", "启动COD", "COD测量中", "延时"}."待机"] -> w116
      tunnel: w114 -> [w122 _ _ _]
      frame "待机", Default {
        n147 = Select(t=enum16{"待机", "启动COD", "COD测量中", "延时"}."启动COD", s=w122, f=enum16{"待机", "启动COD", "COD测量中", "延时"}."待机") -> (s? t:f=w119:enum16{"待机", "启动COD", "COD测量中", "延时"})
      }
      frame "启动COD" {
        n148 = global read "CODMn断电保存全局变量.vi" "定时控制"() -> (w123:T8)
        n149 = Unbundle By Name(w123) -> ("仪器测试类型"=w124:enum16{"水样测试", "标样核查", "空白测试", "跨度核查"})
        n150 = flat-sequence {
          tunnel: w124 -> [w128]
          tunnel: [enum16{"待机", "启动COD", "COD测量中", "延时"}."COD测量中"] -> w125
          frame #0 {
            n151 = case shown="\"空白测试\"" w128 {
              tunnel: [T7 {"测量模式"=enum."水样测量"} ("启动测量模式") T7 {"测量模式"=enum."标样核查"} ("启动测量模式") T7 {"测量模式"=enum."空白测试"} ("启动测量模式") T7 {"测量模式"=enum."跨度核查"} ("启动测量模式")] -> w127
              tunnel: ["水样测试" ("测量模式") "标样核查" ("测量模式") "空白测试" ("测量模式") "跨度核查" ("测量模式")] -> w126
              frame "水样测试", Default {
              }
              frame "标样核查" {
              }
              frame "空白测试" {
              }
              frame "跨度核查" {
              }
            }
            n152 = global write "COD测量模式全局.vi" "测量模式"(w126) -> ()
            n153 = call "CODMn启动命令 (子VI).vi"("启动测量模式"=w127) -> ()  [unwired: 11 in]
          }
          frame #1 {
          }
        }
      }
      frame "COD测量中" {
        n154 = flat-sequence {
          tunnel: [w140] -> w138
          tunnel: [w147] -> w139
          tunnel: w138 -> [w147]
          frame #0 {
            n155 = global read "运行时序全局变量.vi" "多列列表框"() -> (w145:i32)
            n156 = Equal?(x=w145, y=0) -> (x = y?=w143:bool)
            n157 = Select(t=enum16{"待机", "启动COD", "COD测量中", "延时"}."延时", s=w143, f=enum16{"待机", "启动COD", "COD测量中", "延时"}."COD测量中") -> (s? t:f=w140:enum16{"待机", "启动COD", "COD测量中", "延时"})
          }
          frame #1 {
            n158 = Wait (ms)(milliseconds to wait=u32 5000 ("等待时间（毫秒）")) -> ()  [unwired: 1 out]
          }
        }
      }
      frame "延时" {
      }
    }
  }
  n159 = while {
    shift-right: [w180] -> _
    shift-left: u16[] [] ("ORP滴定曲线") -> [w181]
    stop <- FALSE stop-if-true
    # "滴定数-ORP滴定曲线"
    n160 = local read "多列列表框"() -> (w179:i32)
    n161 = Wait (ms)(milliseconds to wait=u32 300 ("等待时间（毫秒）")) -> ()  [unwired: 1 out]
    n162 = Greater Or Equal?(x=w179, y=4) -> (x >= y?=w177:bool)
    n163 = case shown="真" w177 {
      tunnel: w181 -> [_ w195]
      tunnel: [u16[] [] ("ORP滴定曲线") w194] -> w180
      frame False {
      }
      frame True {
        n164 = local read "高锰酸钾"() -> (w191:dbl)
        n165 = local read "多列列表框"() -> (w189:i32)
        n166 = local read "ORP显示"() -> (w190:dbl)
        n167 = Equal?(x=w189, y=5) -> (x = y?=w187:bool)
        n168 = call <vilib>:"Value Has Changed PtByPt.vi"("input data point"=w191) -> ("has changed"=w193:bool, "output data point"=w192:dbl)  [unwired: 1 in]
        n169 = call <vilib>:"Boolean Crossing PtByPt.vi"("direction"=enum16{"either", "false-true", "true-false"}."false-true", "input"=w187) -> ("crossing"=w185:bool)  [unwired: 1 in]
        n170 = case shown="真" w193 {
          tunnel: w195 -> [w201 w211]
          tunnel: [w200 w210] -> w194
          tunnel: w192 -> [w202 w209]
          tunnel: w190 -> [w198 w208]
          frame False {
            n171 = Equal To 0?(x=w202) -> (x = 0?=w199:bool)
            n172 = case shown="真" w199 {
              tunnel: [w203 w206] -> w200
              tunnel: w201 -> [w203 _]
              tunnel: w198 -> [_ w205]
              frame False {
              }
              frame True {
                n173 = Insert Into Array(array=u16[] [] ("ORP滴定曲线"), index=0 ("索引"), new element=w205) -> (w206:u16[])
                n174 = local write "滴定数-ORP值"(w206) -> ()
              }
            }
          }
          frame True {
            n175 = Insert Into Array(array=w211, index=w209, new element=w208) -> (w210:u16[])
            "滴定数-ORP值" <- w210
            n176 = Insert Into Array(array=u16[] [] ("ORP滴定曲线"), new element=w210) -> (→"ORP滴定曲线":u16[])  [unwired: 1 in]
          }
        }
        n177 = case shown="真" w185 {
          frame False {
          }
          frame True {
            n178 = Get Date/Time In Seconds() -> (seconds since 1Jan1904=w196:timestamp)
            n179 = local write "波形时间"(w196) -> ()
            n180 = local read "ORP滴定曲线"() -> (w197:u16[])
            n181 = call "波形存储(子VI).vi"("ORP滴定曲线"=w197) -> ()  [unwired: 11 in]
          }
        }
      }
    }
  }
  n182 = while "While循环" {
    stop <- FALSE stop-if-true
    # "周期启动循环"
    n183 = Get Date/Time In Seconds() -> (seconds since 1Jan1904=w225:timestamp)
    n184 = Wait (ms)(milliseconds to wait=u32 1000 ("等待时间（毫秒）")) -> ()  [unwired: 1 out]
    n185 = Seconds To Date/Time(time stamp (now)=w225) -> (date time rec=w224:T9)  [unwired: 1 in]
    n186 = Unbundle By Name(w224) -> ("时"=w221:i32, "分"=w223:i32)
    n187 = Equal To 0?(x=w223) -> (x = 0?=w222:bool)
    n188 = Index Array(array="24H周期设置", index=w221) -> (element=w220:bool)
    n189 = And(x=w220, y=w222) -> (x .and. y?=w218:bool)
    n190 = call <vilib>:"Boolean Crossing PtByPt.vi"("direction"=enum16{"either", "false-true", "true-false"}."false-true", "input"=w218) -> ("crossing"=w217:bool)  [unwired: 1 in]
    n191 = case shown="真" w217 {
      frame False {
      }
      frame True {
        n192 = Bundle By Name(cluster=T7 {"测量模式"=enum."水样测量"} ("启动测量模式"), "测量模式"="测量模式") -> (w227:T7)
        n193 = call "CODMn启动命令 (子VI).vi"("启动测量模式"=w227) -> ()  [unwired: 11 in]
      }
    }
  }
  n194 = while {
    stop <- FALSE stop-if-true
    # "赋值循环"
    n195 = flat-sequence {
      frame #0 {
        w248 = T11 0 items=["最小二乘", "最小绝对残差", "Bisquare"] ("method")
        # "计算线性、多项式公式"
        n196 = local read "浓度5"() -> (w239:dbl)
        n197 = local read "浓度4"() -> (w240:dbl)
        n198 = local read "浓度2"() -> (w253:dbl)
        n199 = local read "浓度3"() -> (w254:dbl)
        n200 = local read "浓度1"() -> (w252:dbl)
        n201 = local read "泵滴定数3"() -> (w257:dbl)
        n202 = local read "泵滴定数2"() -> (w256:dbl)
        n203 = local read "泵滴定数4"() -> (w238:dbl)
        n204 = local read "泵滴定数5"() -> (w237:dbl)
        n205 = local read "泵滴定数1"() -> (w255:dbl)
        n206 = Build Array("启用1", "启用2", "启用3", "启用4", "启用5") -> (w231:bool[])
        n207 = Build Array(w252, w253, w254, w240, w239) -> (w250:dbl[])
        n208 = Build Array(w255, w256, w257, w238, w237) -> (w249:dbl[])
        n209 = call "线性公式CODMn用.vi"("标液浓度"=w250, "监测浓度"=w249, "启用"=w231, "method"=w248, "模型"="模型", "精度"=6) -> ("拟合方程"=→"拟合公式":string, "r^2"=→"r^2":dbl, "slope"=→"K":dbl, "intercept"=→"b":dbl, "XY图"=→"XY图":cluster{"X Values":dbl[], "Y Values":dbl[]}[], "Polynomial Coefficients"=→"多项式系数1":dbl[])  [unwired: 8 in]
      }
    }
    n210 = flat-sequence {
      frame #0 {
        # "测量数据区"
        n211 = global read "COD读取DATA全局.vi" "data"() -> (w263:T12)
        n212 = global read "COD测量模式全局.vi" "测量模式"() -> (w258:string)
        "测量模式(显示)" <- w258
        n213 = Unbundle By Name(w263) -> ("时间"=w262:timestamp, "检测值"=w261:sgl, "数据标识"=w260:string)
        n214 = local read "测量数据区"() -> (w264:T2)
        n215 = case shown="\"水样测试\"" w258 {
          tunnel: w264 -> [w265 w270 w275 w280 w285 w290 w295 w300]
          tunnel: [w265 w269 w271 w279 w284 w289 w291 w299] -> w259
          tunnel: w262 -> [_ w268 w274 w278 w283 w288 w294 w298]
          tunnel: w261 -> [_ w267 w273 w277 w282 w287 w293 w297]
          tunnel: w260 -> [_ w266 w272 w276 w281 w286 w292 w296]
          frame "", Default {
          }
          frame "水样测试" {
            n216 = Bundle By Name(cluster=w270, "水样数据时间"=w268, "水样实测值"=w267, "水样数据标识"=w266) -> (w269:T2)
          }
          frame "标样核查" {
            n217 = Bundle By Name(cluster=w275, "跨度核查数据时间"=w274, "跨度核查实测值"=w273, "跨度核查数据标识"=w272) -> (w271:T2)
          }
          frame "零点核查" {
            n218 = Bundle By Name(cluster=w280, "零点核查数据时间"=w278, "零点核查实测值"=w277, "零点核查数据标识"=w276) -> (w279:T2)
          }
          frame "加标回收" {
            n219 = Bundle By Name(cluster=w285, "加标回收数据时间"=w283, "加标回收实测值"=w282, "加标回收数据标识"=w281) -> (w284:T2)
          }
          frame "平行样" {
            n220 = Bundle By Name(cluster=w290, "平行样数据时间"=w288, "平行样实测值"=w287, "平行样数据标识"=w286) -> (w289:T2)
          }
          frame "校零" {
            n221 = Bundle By Name(cluster=w295, "空白数据时间"=w294, "空白实测值"=w293, "空白数据标识"=w292) -> (w291:T2)
          }
          frame "校标" {
            n222 = Bundle By Name(cluster=w300, "标样数据时间"=w298, "标样实测值"=w297, "标样数据标识"=w296) -> (w299:T2)
          }
        }
        "测量数据区" <- w259
        n223 = global write "COD读取DATA全局.vi" "测量数据区"(w259) -> ()
      }
    }
    n224 = flat-sequence {
      frame #0 {
        # "显示量程说明"
        n225 = local read "高量程稀释倍数:"() -> (w313:i8)
        n226 = local read "低量程稀释倍数:"() -> (w318:i8)
        n227 = Multiply(x=w313, y=i8 8) -> (x*y=w307:i8)
        n228 = Multiply(x=w318, y=i8 8) -> (x*y=w308:i8)
        n229 = Number To Decimal String(number=w308) -> (decimal integer string=w314:string)  [unwired: 1 in]
        n230 = Number To Decimal String(number=w307) -> (decimal integer string=w311:string)  [unwired: 1 in]
        n231 = Concatenate Strings("L低量程范围:0~" ("量程解释说明"), w314, "(mg/L)\n\nH高量程范围:" ("量程解释说明"), "0" ("字符串"), "~" ("量程解释说明"), w311, "(mg/L)" ("量程解释说明")) -> (→"量程解释说明":string)
      }
    }
    n232 = flat-sequence {
      frame #0 {
        # "权限隐藏和显示功能"
        n233 = local read "自动切换量程:"() -> (w323:enum16{"关闭", "自动切换测一次", "自动切换测两次"})
        n234 = local read "x = y?"() -> (w321:bool)
        n235 = Not Equal To 0?(x=w323) -> (x != 0?=w322:bool)
        n236 = Select(t=T10."Enabled" ("禁用"), s=w322, f=T10."Disabled and Grayed Out" ("禁用")) -> (s? t:f=w324:T10)
        n237 = property on="CODMn零点核查选择" class="Enum (严格)"("Visible"=w321) -> ()  [unwired: 2 in, 2 out]
        n238 = property on="高量程稀释倍数:" class="DigNum (严格)"("Visible"=w321) -> ()  [unwired: 2 in, 2 out]
        n239 = property on="低量程稀释倍数:" class="DigNum (严格)"("Visible"=w321) -> ()  [unwired: 2 in, 2 out]
        n240 = property on="稀释倍数解释" class="Str"("Visible"=w321) -> ()  [unwired: 2 in, 2 out]
        n241 = property on="低切高阈值:" class="DigNum (严格)"("DisabledEnum"=w324) -> ()  [unwired: 2 in, 2 out]
        n242 = property on="高切低阈值:" class="DigNum (严格)"("DisabledEnum"=w324) -> ()  [unwired: 2 in, 2 out]
      }
    }
    n243 = Wait (ms)(milliseconds to wait=u32 1000 ("等待时间（毫秒）")) -> ()  [unwired: 1 out]
    n244 = flat-sequence {
      frame #0 {
        # "断电保存全局给局部变量"
        n245 = global read "CODMn断电保存全局变量.vi" "CODMn跨度量程选择"() -> (w305:enum32{"H", "L", "AUTO"})
        n246 = global read "CODMn断电保存全局变量.vi" "测量模式(公式)"() -> (w306:u16)
        n247 = global read "CODMn断电保存全局变量.vi" "高切低阈值:"() -> (w304:dbl)
        n248 = global read "CODMn断电保存全局变量.vi" "自动切换量程:"() -> (w302:enum16{"关闭", "自动切换测一次", "自动切换测两次"})
        n249 = global read "CODMn断电保存全局变量.vi" "低切高阈值:"() -> (w303:dbl)
        n250 = global read "CODMn断电保存全局变量.vi" "跨度液浓度"() -> (w301:dbl)
        n251 = local write "测量模式(公式)"(w306) -> ()
        n252 = local write "CODMn跨度量程选择"(w305) -> ()
        n253 = local write "自动切换量程:"(w302) -> ()
        n254 = local write "高切低阈值:"(w304) -> ()
        n255 = local write "低切高阈值:"(w303) -> ()
        n256 = local write "跨度液浓度"(w301) -> ()
      }
    }
  }
  n257 = flat-sequence {
    tunnel: w16 -> [w334]
    tunnel: w15 -> [w333]
    frame #0 {
      n258 = property on="窗格" class="Pane"("Origin"=T13 {"Horizontal"=0, "Vertical"=0} ("原点")) -> ()  [unwired: 2 in, 2 out]
      n259 = property on="VISA resource name" class="VISAName"() -> ("Value"=→"文本.文本":refnum<visa-resource-name>)  [unwired: 2 in, 2 out]
      n260 = Bundle By Name(cluster=T5 {"starting address"=0, "number of holding registers"=0}, "starting address"=u16 4240, "number of holding registers"=u16 16) -> (w341:T5)
      n261 = local write "量程切换次数"(u8 0 ("量程切换次数")) -> ()
      n262 = local write "切换量程连续测两次"(FALSE ("切换量程连续测两次")) -> ()
      n263 = local write "枚举"(enum16{"读取数据", "写入数据", "读取写入DATABASE", "读取参数"}."读取参数" ("枚举")) -> ()
      n264 = Flush Queue(queue=w334, error in (no error)=w333) -> (queue out=w337:refnum<queue>, error out=w336:errorcluster)  [unwired: 1 out]
      n265 = local write "选用水样"(enum16{"葡萄糖", "草酸钠"}."葡萄糖" ("选用水样")) -> ()
      n266 = local write "量程选择"(enum16{"低量程", "高量程", "0-2量程"}."低量程" ("量程选择")) -> ()
      n267 = Enqueue Element(queue=w337, element=w341, error in (no error)=w336) -> ()  [unwired: 1 in, 3 out]
      "稀释倍数解释" <- "稀释倍数解释：\n稀释倍数选择1，表示不稀释\n默认低量程系数倍数1，高量程系数倍数2\n则低量程为0~8，高量程为0~16" ("稀释倍数解释")
    }
  }
  n268 = call <vilib>:"Application Directory.vi"() -> ("Application Directory"=w5:path)
  n269 = Build Path(base path=w5, name or relative path="data\\sys.ini" ("名称或相对路径")) -> (appended path=w7:path)
  n270 = call <vilib>:"Open Config Data.vi"("configuration file path"=w7) -> ("error out"=w11:errorcluster, "refnum"=w8:T6)  [unwired: 8 in, 1 out]
  n271 = vi-ref "斯坦道CODMn.lvlib:CODMn断电保存全局变量.vi"() -> (w9:refnum<vi>)
  n272 = global write "COD浓度全局变量.vi" "VISA resource name"("VISA resource name") -> ()
  n273 = call <userlib>:"Read Panel from INI__ogtk.vi"("error in (no error)"=w11, "VI ref"=w9, "refnum"=w8) -> ("error out"=w12:errorcluster, "refnum out"=w10:T6)  [unwired: 7 in]
  n274 = call <vilib>:"Close Config Data.vi"("error in (no error)"=w12, "refnum"=w10) -> ("error out"=w13:errorcluster, "file path"=w14:path)  [unwired: 8 in]
  n275 = Open/Create/Replace File(file path (use dialog)=w14, error in=w13) -> (error out=w4:errorcluster)  [unwired: 4 in, 2 out]
  n276 = call <vilib>:"Open Serial Session.vi"("Mode (RTU)"=enum16{"RTU", "ASCII"}."RTU", "Slave ID"="Slave ID", "Serial Config"="Serial Config", "VISA Resource"="VISA resource name") -> ("Error out"=w2:errorcluster, "MB_Serial session"=w3:refnum<class "MB_Master_Serial.lvclass">)  [unwired: 6 in]
  n277 = global write "COD浓度全局变量.vi" "MB_Serial session"(w3) -> ()
  n278 = global write "COD浓度全局变量.vi" "Error in"(w2) -> ()
  n279 = Obtain Queue(max queue size (-1, unlimited)=-1 ("队列最大值（-1，无限）"), name (unnamed)="CODMn读取写入DATABASE" ("名称（未命名）"), element data type=T5 {"starting address"=4224, "number of holding registers"=16}) -> (queue out=w22:refnum<queue>, error out=w21:errorcluster)  [unwired: 2 in, 1 out]
  n280 = Obtain Queue(max queue size (-1, unlimited)=-1 ("队列最大值（-1，无限）"), name (unnamed)="CODMn读取参数" ("名称（未命名）"), element data type=T5 {"starting address"=4224, "number of holding registers"=16}) -> (queue out=w16:refnum<queue>, error out=w15:errorcluster)  [unwired: 2 in, 1 out]
  n281 = Obtain Queue(max queue size (-1, unlimited)=-1 ("队列最大值（-1，无限）"), name (unnamed)="CODMn写入" ("名称（未命名）"), element data type=cluster{"starting address":u16, "values":u16[]} {"starting address"=4272, "values"=[]}) -> (queue out=w1:refnum<queue>, error out=w20:errorcluster)  [unwired: 2 in, 1 out]
  n282 = Obtain Queue(max queue size (-1, unlimited)=-1 ("队列最大值（-1，无限）"), name (unnamed)="CODMn读取" ("名称（未命名）"), element data type=T5 {"starting address"=4224, "number of holding registers"=16}) -> (queue out=w32:refnum<queue>, error out=w31:errorcluster)  [unwired: 2 in, 1 out]
  n283 = while {
    tunnel: w32 -> [w350]
    tunnel: w31 -> [w349]
    tunnel: w1 -> [w348]
    tunnel: w16 -> [w347]
    tunnel: w15 -> [w346]
    tunnel: w3 -> [w344]
    tunnel: w2 -> [w343]
    tunnel: w4 -> [_]
    stop <- FALSE stop-if-true
    n284 = event shown="[1] \"启动\": 鼠标按下" {
      selector: _ -> [_ _ _ _ _ _ _ _ _ _ _ _ _ _ _ _ _ _ _ _ _ _ _ _ _ _ _ _ _ _ _]
      dyn-events: _ -> [_ _ _ _ _ _ _ _ _ _ _ _ _ _ _ _ _ _ _ _ _ _ _ _ _ _ _ _ _ _ _]
      timeout: _ -> [_ _ _ _ _ _ _ _ _ _ _ _ _ _ _ _ _ _ _ _ _ _ _ _ _ _ _ _ _ _ _]
      tunnel: w350 -> [_ _ _ _ _ _ _ _ _ _ _ _ _ _ _ _ _ _ _ _ _ _ _ _ _ _ _ _ _ _ _]
      tunnel: w349 -> [_ _ _ _ _ _ _ _ _ _ _ _ _ _ _ _ _ _ _ _ _ _ _ _ _ _ _ _ _ _ _]
      tunnel: w348 -> [w358 w391 w433 _ _ _ w491 _ _ _ _ _ _ _ _ w852 w866 _ _ _ _ w919 _ _ _ _ w1105 w1205 _ _ _]
      tunnel: w347 -> [_ _ _ _ _ w470 _ _ _ _ _ _ _ _ _ _ _ _ _ _ _ _ _ _ _ w1097 _ _ _ _ _]
      tunnel: w346 -> [_ _ _ _ _ w469 _ _ _ _ _ _ _ _ _ _ _ _ _ _ _ _ _ _ _ w1096 _ _ _ _ _]
      tunnel: w344 -> [_ _ _ w441 _ _ _ _ _ _ _ _ _ _ w851 _ _ _ _ _ _ _ _ _ _ _ _ _ _ _ _]
      tunnel: w343 -> [_ _ _ w440 _ _ _ _ _ _ _ _ _ _ w850 _ _ _ _ _ _ _ _ _ _ _ _ _ _ _ _]
      event "单步启动": Mouse Down {
        n285 = event-data() -> ()  [unwired: 1 in, 8 out]
        n286 = call "单步启动选择对话框.vi"() -> ("启动选择2"=w351:u16)  [unwired: 10 in, 1 out]
        n287 = case shown="3" w351 {
          tunnel: [u16 4610 ("address") u16 4610 ("address") u16 4610 ("address") u16 4610 ("address") u16 4610 ("address") u16 4610 ("address") u16 4610 ("address") u16 4610 ("address") u16 4610 ("address") u16 4610 ("address") u16 4610 ("address") u16 4610 ("address") u16 4610 ("address")] -> w357
          tunnel: [u16 1 ("address") u16 2 ("address") u16 3 ("address") u16 4 ("address") u16 5 ("address") u16 6 ("address") u16 7 ("address") u16 8 ("address") u16 9 ("holding register value") u16 10 ("holding register value") u16 11 ("holding register value") u16 12 ("address") u16 0 ("address")] -> w354
          frame 0 {
          }
          frame 1 {
          }
          frame 2 {
          }
          frame 3 {
          }
          frame 4 {
          }
          frame 5 {
          }
          frame 6 {
          }
          frame 7 {
          }
          frame 8 {
          }
          frame 9 {
          }
          frame 10 {
          }
          frame 11 {
          }
          frame 12, Default {
          }
        }
        n288 = local write "枚举"(enum16{"读取数据", "写入数据", "读取写入DATABASE", "读取参数"}."写入数据" ("枚举")) -> ()
        n289 = Insert Into Array(array=u16[] [] ("values"), index=0 ("索引"), new element=w354) -> (w353:u16[])
        n290 = Bundle By Name(cluster=cluster{"starting address":u16, "values":u16[]} {"starting address"=0, "values"=[]}, "starting address"=w357, "values"=w353) -> (w359:cluster{"starting address":u16, "values":u16[]})
        n291 = Enqueue Element(queue=w358, element=w359) -> ()  [unwired: 2 in, 3 out]
      }
      event "启动": Mouse Down {
        n292 = event-data() -> ()  [unwired: 1 in, 8 out]
        n293 = flat-sequence {
          tunnel: w391 -> [w394]
          tunnel: [w394] -> w390
          tunnel: [w393] -> w387
          tunnel: w390 -> [w397]
          tunnel: [w397] -> w389
          tunnel: [w395] -> w388
          tunnel: w387 -> [w395]
          tunnel: w389 -> [w401]
          tunnel: w388 -> [w400]
          frame #0 {
            n294 = call "启动测量模式选择对话框.vi"() -> ("启动选择 2"=w393:u16)  [unwired: 11 in]
            "启动选择 2" <- w393
          }
          frame #1 {
            n295 = property on="启动选择 2" class="Ring (严格)"() -> ("RingText.Text"=w396:string)  [unwired: 2 in, 2 out]
            n296 = global write "COD测量模式全局.vi" "测量模式"(w396) -> ()
          }
          frame #2 {
            n297 = case shown="9, 默认" w400 {
              tunnel: [u16 4608 ("address") u16 4608 ("address") u16 4608 ("address") u16 4608 ("address") u16 4608 ("address") u16 4608 ("address") u16 4608 ("address") u16 4608 ("address") u16 4608 ("address") u16 4608 ("address")] -> w402
              tunnel: [u16 1 ("address") u16 2 ("address") u16 3 ("address") u16 4 ("address") u16 5 ("address") u16 7 ("address") u16 6 ("address") u16 8 ("address") u16 9 ("address") u16 0 ("address")] -> w403
              frame 0 {
              }
              frame 1 {
              }
              frame 2 {
              }
              frame 3 {
              }
              frame 4 {
              }
              frame 5 {
              }
              frame 6 {
              }
              frame 7 {
              }
              frame 8 {
              }
              frame 9, Default {
              }
            }
            n298 = Not Equal?(x=w400, y=u16 9) -> (x != y?=w398:bool)
            n299 = global write "CODMN外部API.vi" "手动启动CODMn"(w398) -> ()
            n300 = Insert Into Array(array=u16[] [] ("values"), index=0 ("索引"), new element=w403) -> (w408:u16[])
            n301 = Bundle By Name(cluster=cluster{"starting address":u16, "values":u16[]} {"starting address"=0, "values"=[]}, "starting address"=w402, "values"=w408) -> (w405:cluster{"starting address":u16, "values":u16[]})
            n302 = Enqueue Element(queue=w401, element=w405) -> ()  [unwired: 2 in, 3 out]
          }
        }
        n303 = local write "枚举"(enum16{"读取数据", "写入数据", "读取写入DATABASE", "读取参数"}."写入数据" ("枚举")) -> ()
      }
      event "停止": Value Change {
        n304 = event-data() -> ()  [unwired: 1 in, 6 out]
        n305 = Two Button Dialog(message="确认是否停止？" ("消息"), 1:"否" ("F按钮名称（“取消”）"), 2:"是" ("T按钮名称（“确定”）")) -> (T button?=w431:bool)
        n306 = case shown="真" w431 {
          tunnel: w433 -> [_ w435]
          frame False {
          }
          frame True {
            n307 = local write "枚举"(enum16{"读取数据", "写入数据", "读取写入DATABASE", "读取参数"}."写入数据" ("枚举")) -> ()
            n308 = Bundle By Name(cluster=cluster{"starting address":u16, "values":u16[]} {"starting address"=0, "values"=[]}, "starting address"=u16 4608, "values"=u16[] [11]) -> (w437:cluster{"starting address":u16, "values":u16[]})
            n309 = Enqueue Element(queue=w435, element=w437) -> ()  [unwired: 2 in, 3 out]
          }
        }
      }
      event "手动控制": Value Change {
        n310 = event-data() -> ()  [unwired: 1 in, 6 out]
        n311 = call "数字密码键盘.vi"() -> ("NewNumber"=w442:sgl)  [unwired: 1 in]
        n312 = Equal?(x=w442, y=8.0) -> (x = y?=w443:bool)
        n313 = case shown="真" w443 {
          tunnel: w441 -> [_ w447]
          tunnel: w440 -> [_ w446]
          frame False {
            n314 = call "窗口弹出对话框(子VI).vi"("消息"="密码错误") -> ()  [unwired: 10 in, 1 out]
          }
          frame True {
            n315 = call "CODMn手动控制框.vi"("Error in"=w446, "MB_Serial session"=w447) -> ()  [unwired: 10 in]
          }
        }
      }
      event "锁定按钮": Mouse Down {
        n316 = event-data() -> ("CtlRef"=w450:refnum<vi>)  [unwired: 1 in, 7 out]
        n317 = property class="Bool (严格)"(reference=w450) -> ("Value"=w449:bool)  [unwired: 1 in, 2 out]
        n318 = case shown="真" w449 {
          selector: w449 -> [w451 _]
          tunnel: [w451 w452] -> w448
          frame False {
          }
          frame True {
            n319 = call "数字密码键盘.vi"() -> ("NewNumber"=w453:sgl)  [unwired: 1 in]
            n320 = Equal?(x=w453, y=8.0) -> (x = y?=w452:bool)
            n321 = case shown="假" w452 {
              selector: w452 -> [w456 _]
              frame False {
                n322 = One Button Dialog(message="密码错误!" ("消息")) -> ()  [unwired: 1 in, 1 out]
                n323 = local write "锁定按钮"(w456) -> ()
              }
              frame True {
                n324 = One Button Dialog(message="解锁成功!" ("消息")) -> ()  [unwired: 1 in, 1 out]
              }
            }
          }
        }
        "x = y?" <- w448
      }
      event "参数配置": Value Change {
        n325 = event-data() -> ()  [unwired: 1 in, 6 out]
        n326 = call <vilib>:"Application Directory.vi"() -> ("Application Directory"=w458:path)
        n327 = Build Path(base path=w458, name or relative path="data\\sys.ini" ("名称或相对路径")) -> (appended path=w460:path)
        n328 = call <vilib>:"Open Config Data.vi"("configuration file path"=w460) -> ("error out"=w464:errorcluster, "refnum"=w461:T6)  [unwired: 8 in, 1 out]
        n329 = property on="窗格" class="Pane"("Origin"=T13 {"Horizontal"=0, "Vertical"=650} ("原点")) -> ()  [unwired: 2 in, 2 out]
        n330 = vi-ref "斯坦道CODMn.lvlib:CODMn断电保存全局变量.vi"() -> (w462:refnum<vi>)
        n331 = call <userlib>:"Read Panel from INI__ogtk.vi"("error in (no error)"=w464, "VI ref"=w462, "refnum"=w461) -> ("error out"=w465:errorcluster, "refnum out"=w463:T6)  [unwired: 7 in]
        n332 = Bundle By Name(cluster=T5 {"starting address"=0, "number of holding registers"=0}, "starting address"=u16 4272, "number of holding registers"=u16 20) -> (w477:T5)
        n333 = call <vilib>:"Close Config Data.vi"("error in (no error)"=w465, "refnum"=w463) -> ("error out"=w466:errorcluster, "file path"=w467:path)  [unwired: 8 in]
        n334 = Open/Create/Replace File(file path (use dialog)=w467, error in=w466) -> ()  [unwired: 4 in, 3 out]
        n335 = local write "读取KB值"(FALSE ("读取KB值")) -> ()
        n336 = local write "枚举"(enum16{"读取数据", "写入数据", "读取写入DATABASE", "读取参数"}."读取参数" ("枚举")) -> ()
        n337 = Flush Queue(queue=w470, error in (no error)=w469) -> (queue out=w473:refnum<queue>, error out=w472:errorcluster)  [unwired: 1 out]
        n338 = Enqueue Element(queue=w473, element=w477, error in (no error)=w472) -> ()  [unwired: 1 in, 3 out]
      }
      event "保存": Mouse Down {
        n339 = event-data() -> ()  [unwired: 1 in, 8 out]
        n340 = local write "枚举"(enum16{"读取数据", "写入数据", "读取写入DATABASE", "读取参数"}."写入数据" ("枚举")) -> ()
        n341 = local read "CODMn零点核查选择"() -> (w479:enum16{"零点核查走纯水管", "零点核查走质控管"})
        n342 = Multiply(x="温度", y=10.0) -> (x*y=w488:dbl)
        n343 = Multiply(x="标准液浓度", y=100.0) -> (x*y=w482:dbl)
        n344 = Multiply(x="修正系数", y=100.0) -> (x*y=w485:dbl)
        n345 = Build Array(w488, "恒温时间", w482, w485, "基本量程", "水样", "蒸馏水", "标液", "质控样", "加标回收", "高锰酸钾", "草酸钠", "硫酸", "零点泵计量数 2", "标度泵计量数 2", "高量程稀释倍数:", "低量程稀释倍数:", w479) -> (w505:dbl[])
        n346 = Bundle By Name(cluster=cluster{"starting address":u16, "values":u16[]} {"starting address"=4272, "values"=[]}, "starting address"=u16 4272, "values"=w505) -> (w507:cluster{"starting address":u16, "values":u16[]})
        n347 = Enqueue Element(queue=w491, element=w507, timeout in ms (-1)=1000 ("超时毫秒(-1)")) -> ()  [unwired: 1 in, 3 out]
      }
      event "跨度液浓度": Value Change {
        n348 = event-data() -> ()  [unwired: 1 in, 6 out]
        n349 = flat-sequence {
          frame #0 {
            n350 = global write "CODMn断电保存全局变量.vi" "跨度液浓度"("跨度液浓度") -> ()
          }
          frame #1 {
            n351 = call <vilib>:"Application Directory.vi"() -> ("Application Directory"=w524:path)
            n352 = Build Path(base path=w524, name or relative path="data\\sys.ini" ("名称或相对路径")) -> (appended path=w522:path)
            n353 = call <vilib>:"Open Config Data.vi"("configuration file path"=w522) -> ("error out"=w518:errorcluster, "refnum"=w521:T6)  [unwired: 8 in, 1 out]
            n354 = vi-ref "斯坦道CODMn.lvlib:CODMn断电保存全局变量.vi"() -> (w520:refnum<vi>)
            n355 = call <userlib>:"Write Panel to INI__ogtk.vi"("error in (no error)"=w518, "VI ref"=w520, "refnum"=w521) -> ("error out"=w517:errorcluster, "refnum out"=w519:T6)  [unwired: 7 in]
            n356 = call <vilib>:"Close Config Data.vi"("error in (no error)"=w517, "refnum"=w519) -> ("error out"=w512:errorcluster, "file path"=w511:path)  [unwired: 8 in]
            n357 = Open/Create/Replace File(file path (use dialog)=w511, error in=w512) -> (refnum out=w515:refnum<file>, error out=w516:errorcluster)  [unwired: 4 in, 1 out]
            n358 = Flush File(refnum=w515, error in=w516) -> (refnum out=w514:refnum<file>, error out=w513:errorcluster)
            n359 = Close File(refnum=w514, error in=w513) -> ()  [unwired: 2 out]
          }
        }
      }
      event "校准配置": Value Change {
        n360 = event-data() -> ()  [unwired: 1 in, 6 out]
        n361 = property on="窗格" class="Pane"("Origin"=T13 {"Horizontal"=0, "Vertical"=1300} ("原点")) -> ()  [unwired: 2 in, 2 out]
        n362 = call <vilib>:"Application Directory.vi"() -> ("Application Directory"=w575:path)
        n363 = Build Path(base path=w575, name or relative path="data\\Set.ini" ("名称或相对路径")) -> (appended path=w573:path)
        n364 = call <vilib>:"Open Config Data.vi"("configuration file path"=w573) -> ("error out"=w543:errorcluster, "refnum"=w544:T6)  [unwired: 8 in, 1 out]
        n365 = call-poly <vilib>:"Read Key.vi"("section"="CODMn模型选择" ("key"), "error in (no error)"=w543, "key"="线性和多项式", "refnum"=w544) -> ("error out"=w539:errorcluster, "value"=w542:i32, "refnum out"=w540:T6)  [unwired: 4 in, 1 out]
        n366 = local write "模型"(w542) -> ()
        n367 = call-poly <vilib>:"Read Key.vi"("section"="标线选择", "error in (no error)"=w539, "key"="选用水样", "refnum"=w540) -> ("error out"=w537:errorcluster, "value"=w541:i32, "refnum out"=w538:T6)  [unwired: 4 in, 1 out]
        n368 = local write "选用水样"(w541) -> ()
        n369 = local read "量程选择"() -> (w550:enum16{"低量程", "高量程", "0-2量程"})
        n370 = case shown="0, 默认" w541 {
          tunnel: ["葡萄糖标线" ("section") "草酸钠标线" ("section")] -> w549
          frame 0, Default {
          }
          frame 1 {
          }
        }
        n371 = case shown="\"0-2量程\"" w550 {
          tunnel: ["低量程" "高量程" "0-2量程"] -> w548
          frame "低量程", Default {
          }
          frame "高量程" {
          }
          frame "0-2量程" {
          }
        }
        n372 = Concatenate Strings(w549, w548) -> (w547:string)
        n373 = call-poly <vilib>:"Read Key.vi"("section"=w547, "error in (no error)"=w537, "key"="浓度1", "refnum"=w538) -> ("error out"=w579:errorcluster, "value"=w577:dbl, "refnum out"=w578:T6)  [unwired: 4 in, 1 out]
        n374 = local write "浓度1"(w577) -> ()
        n375 = call-poly <vilib>:"Read Key.vi"("section"=w547, "error in (no error)"=w579, "key"="浓度2", "refnum"=w578) -> ("error out"=w593:errorcluster, "value"=w580:dbl, "refnum out"=w592:T6)  [unwired: 4 in, 1 out]
        n376 = local write "浓度2"(w580) -> ()
        n377 = call-poly <vilib>:"Read Key.vi"("section"=w547, "error in (no error)"=w593, "key"="浓度3", "refnum"=w592) -> ("error out"=w594:errorcluster, "value"=w582:dbl, "refnum out"=w591:T6)  [unwired: 4 in, 1 out]
        n378 = local write "浓度3"(w582) -> ()
        n379 = call-poly <vilib>:"Read Key.vi"("section"=w547, "error in (no error)"=w594, "key"="泵滴定数1", "refnum"=w591) -> ("error out"=w595:errorcluster, "value"=w584:dbl, "refnum out"=w590:T6)  [unwired: 4 in, 1 out]
        n380 = local write "泵滴定数1"(w584) -> ()
        n381 = call-poly <vilib>:"Read Key.vi"("section"=w547, "error in (no error)"=w595, "key"="泵滴定数2", "refnum"=w590) -> ("error out"=w589:errorcluster, "value"=w587:dbl, "refnum out"=w596:T6)  [unwired: 4 in, 1 out]
        n382 = local write "泵滴定数2"(w587) -> ()
        n383 = call-poly <vilib>:"Read Key.vi"("section"=w547, "error in (no error)"=w589, "key"="泵滴定数3", "refnum"=w596) -> ("error out"=w601:errorcluster, "value"=w600:dbl, "refnum out"=w597:T6)  [unwired: 4 in, 1 out]
        n384 = local write "泵滴定数3"(w600) -> ()
        n385 = call-poly <vilib>:"Read Key.vi"("section"=w547, "error in (no error)"=w601, "key"="浓度4", "refnum"=w597) -> ("error out"=w602:errorcluster, "value"=w530:dbl, "refnum out"=w598:T6)  [unwired: 4 in, 1 out]
        n386 = local write "浓度4"(w530) -> ()
        n387 = call-poly <vilib>:"Read Key.vi"("section"=w547, "error in (no error)"=w602, "key"="浓度5", "refnum"=w598) -> ("error out"=w535:errorcluster, "value"=w529:dbl, "refnum out"=w536:T6)  [unwired: 4 in, 1 out]
        n388 = local write "浓度5"(w529) -> ()
        n389 = call-poly <vilib>:"Read Key.vi"("section"=w547, "error in (no error)"=w535, "key"="泵滴定数4", "refnum"=w536) -> ("error out"=w603:errorcluster, "value"=w528:dbl, "refnum out"=w599:T6)  [unwired: 4 in, 1 out]
        n390 = local write "泵滴定数4"(w528) -> ()
        n391 = call-poly <vilib>:"Read Key.vi"("section"=w547, "error in (no error)"=w603, "key"="泵滴定数5", "refnum"=w599) -> ("error out"=w533:errorcluster, "value"=w527:dbl, "refnum out"=w534:T6)  [unwired: 4 in, 1 out]
        n392 = local write "泵滴定数5"(w527) -> ()
        n393 = call-poly <vilib>:"Read Key.vi"("section"=w547, "error in (no error)"=w533, "key"="当前选用的校准", "refnum"=w534) -> ("error out"=w569:errorcluster, "value"=w571:i32, "refnum out"=w570:T6)  [unwired: 4 in, 1 out]
        n394 = local write "当前校准"(w571) -> ()
        n395 = call-poly <vilib>:"Read Key.vi"("section"=w547, "error in (no error)"=w569, "key"="启用1", "refnum"=w570) -> ("error out"=w566:errorcluster, "value"=w555:bool, "refnum out"=w567:T6)  [unwired: 4 in, 1 out]
        n396 = local write "启用1"(w555) -> ()
        n397 = call-poly <vilib>:"Read Key.vi"("section"=w547, "error in (no error)"=w566, "key"="启用2", "refnum"=w567) -> ("error out"=w564:errorcluster, "value"=w554:bool, "refnum out"=w565:T6)  [unwired: 4 in, 1 out]
        n398 = local write "启用2"(w554) -> ()
        n399 = call-poly <vilib>:"Read Key.vi"("section"=w547, "error in (no error)"=w564, "key"="启用3", "refnum"=w565) -> ("error out"=w562:errorcluster, "value"=w553:bool, "refnum out"=w563:T6)  [unwired: 4 in, 1 out]
        n400 = local write "启用3"(w553) -> ()
        n401 = call-poly <vilib>:"Read Key.vi"("section"=w547, "error in (no error)"=w562, "key"="启用4", "refnum"=w563) -> ("error out"=w560:errorcluster, "value"=w526:bool, "refnum out"=w561:T6)  [unwired: 4 in, 1 out]
        n402 = local write "启用4"(w526) -> ()
        n403 = call-poly <vilib>:"Read Key.vi"("section"=w547, "error in (no error)"=w560, "key"="启用5", "refnum"=w561) -> ("error out"=w531:errorcluster, "value"=w525:bool, "refnum out"=w532:T6)  [unwired: 4 in, 1 out]
        n404 = local write "启用5"(w525) -> ()
        n405 = call <vilib>:"Close Config Data.vi"("error in (no error)"=w531, "refnum"=w532) -> ()  [unwired: 8 in, 2 out]
      }
      event "选用水样": Value Change {
        (unwired) "浓度6" ("key")
        n406 = event-data() -> ()  [unwired: 1 in, 6 out]
        n407 = property on="窗格" class="Pane"("Origin"=T13 {"Horizontal"=0, "Vertical"=1300} ("原点")) -> ()  [unwired: 2 in, 2 out]
        n408 = local read "量程选择"() -> (w627:enum16{"低量程", "高量程", "0-2量程"})
        n409 = case shown="\"0-2量程\"" w627 {
          tunnel: ["低量程" "高量程" "0-2量程"] -> w628
          frame "低量程", Default {
          }
          frame "高量程" {
          }
          frame "0-2量程" {
          }
        }
        n410 = case shown="\"葡萄糖\", 默认" "选用水样" {
          tunnel: ["葡萄糖标线" ("section") "草酸钠标线" ("section")] -> w629
          frame "葡萄糖", Default {
          }
          frame "草酸钠" {
          }
        }
        n411 = call <vilib>:"Application Directory.vi"() -> ("Application Directory"=w653:path)
        n412 = Build Path(base path=w653, name or relative path="data\\Set.ini" ("名称或相对路径")) -> (appended path=w651:path)
        n413 = call <vilib>:"Open Config Data.vi"("configuration file path"=w651) -> ("error out"=w654:errorcluster, "refnum"=w655:T6)  [unwired: 8 in, 1 out]
        n414 = Concatenate Strings(w629, w628) -> (w626:string)
        n415 = call-poly <vilib>:"Read Key.vi"("section"=w626, "error in (no error)"=w654, "key"="浓度1", "refnum"=w655) -> ("error out"=w659:errorcluster, "value"=w657:dbl, "refnum out"=w658:T6)  [unwired: 4 in, 1 out]
        n416 = local write "浓度1"(w657) -> ()
        n417 = call-poly <vilib>:"Read Key.vi"("section"=w626, "error in (no error)"=w659, "key"="浓度2", "refnum"=w658) -> ("error out"=w673:errorcluster, "value"=w660:dbl, "refnum out"=w672:T6)  [unwired: 4 in, 1 out]
        n418 = local write "浓度2"(w660) -> ()
        n419 = call-poly <vilib>:"Read Key.vi"("section"=w626, "error in (no error)"=w673, "key"="浓度3", "refnum"=w672) -> ("error out"=w674:errorcluster, "value"=w662:dbl, "refnum out"=w671:T6)  [unwired: 4 in, 1 out]
        n420 = local write "浓度3"(w662) -> ()
        n421 = call-poly <vilib>:"Read Key.vi"("section"=w626, "error in (no error)"=w674, "key"="泵滴定数1", "refnum"=w671) -> ("error out"=w675:errorcluster, "value"=w664:dbl, "refnum out"=w670:T6)  [unwired: 4 in, 1 out]
        n422 = local write "泵滴定数1"(w664) -> ()
        n423 = call-poly <vilib>:"Read Key.vi"("section"=w626, "error in (no error)"=w675, "key"="泵滴定数2", "refnum"=w670) -> ("error out"=w669:errorcluster, "value"=w667:dbl, "refnum out"=w676:T6)  [unwired: 4 in, 1 out]
        n424 = local write "泵滴定数2"(w667) -> ()
        n425 = call-poly <vilib>:"Read Key.vi"("section"=w626, "error in (no error)"=w669, "key"="泵滴定数3", "refnum"=w676) -> ("error out"=w681:errorcluster, "value"=w680:dbl, "refnum out"=w677:T6)  [unwired: 4 in, 1 out]
        n426 = local write "泵滴定数3"(w680) -> ()
        n427 = call-poly <vilib>:"Read Key.vi"("section"=w626, "error in (no error)"=w681, "key"="浓度4", "refnum"=w677) -> ("error out"=w682:errorcluster, "value"=w621:dbl, "refnum out"=w678:T6)  [unwired: 4 in, 1 out]
        n428 = local write "浓度4"(w621) -> ()
        n429 = call-poly <vilib>:"Read Key.vi"("section"=w626, "error in (no error)"=w682, "key"="浓度5", "refnum"=w678) -> ("error out"=w624:errorcluster, "value"=w620:dbl, "refnum out"=w625:T6)  [unwired: 4 in, 1 out]
        n430 = local write "浓度5"(w620) -> ()
        n431 = call-poly <vilib>:"Read Key.vi"("section"=w626, "error in (no error)"=w624, "key"="泵滴定数4", "refnum"=w625) -> ("error out"=w683:errorcluster, "value"=w619:dbl, "refnum out"=w679:T6)  [unwired: 4 in, 1 out]
        n432 = local write "泵滴定数4"(w619) -> ()
        n433 = call-poly <vilib>:"Read Key.vi"("section"=w626, "error in (no error)"=w683, "key"="泵滴定数5", "refnum"=w679) -> ("error out"=w622:errorcluster, "value"=w618:dbl, "refnum out"=w623:T6)  [unwired: 4 in, 1 out]
        n434 = local write "泵滴定数5"(w618) -> ()
        n435 = call-poly <vilib>:"Read Key.vi"("section"=w626, "error in (no error)"=w622, "key"="当前选用的校准", "refnum"=w623) -> ("error out"=w647:errorcluster, "value"=w649:i32, "refnum out"=w648:T6)  [unwired: 4 in, 1 out]
        n436 = local write "当前校准"(w649) -> ()
        n437 = call-poly <vilib>:"Read Key.vi"("section"=w626, "error in (no error)"=w647, "key"="启用1", "refnum"=w648) -> ("error out"=w644:errorcluster, "value"=w633:bool, "refnum out"=w645:T6)  [unwired: 4 in, 1 out]
        n438 = local write "启用1"(w633) -> ()
        n439 = call-poly <vilib>:"Read Key.vi"("section"=w626, "error in (no error)"=w644, "key"="启用2", "refnum"=w645) -> ("error out"=w642:errorcluster, "value"=w632:bool, "refnum out"=w643:T6)  [unwired: 4 in, 1 out]
        n440 = local write "启用2"(w632) -> ()
        n441 = call-poly <vilib>:"Read Key.vi"("section"=w626, "error in (no error)"=w642, "key"="启用3", "refnum"=w643) -> ("error out"=w640:errorcluster, "value"=w631:bool, "refnum out"=w641:T6)  [unwired: 4 in, 1 out]
        n442 = local write "启用3"(w631) -> ()
        n443 = call-poly <vilib>:"Read Key.vi"("section"=w626, "error in (no error)"=w640, "key"="启用4", "refnum"=w641) -> ("error out"=w638:errorcluster, "value"=w615:bool, "refnum out"=w639:T6)  [unwired: 4 in, 1 out]
        n444 = local write "启用4"(w615) -> ()
        n445 = call-poly <vilib>:"Read Key.vi"("section"=w626, "error in (no error)"=w638, "key"="启用5", "refnum"=w639) -> ("error out"=w616:errorcluster, "value"=w614:bool, "refnum out"=w617:T6)  [unwired: 4 in, 1 out]
        n446 = local write "启用5"(w614) -> ()
        n447 = call <vilib>:"Close Config Data.vi"("error in (no error)"=w616, "refnum"=w617) -> ()  [unwired: 8 in, 2 out]
      }
      event "量程选择": Value Change {
        n448 = event-data() -> ()  [unwired: 1 in, 6 out]
        n449 = property on="窗格" class="Pane"("Origin"=T13 {"Horizontal"=0, "Vertical"=1300} ("原点")) -> ()  [unwired: 2 in, 2 out]
        n450 = local read "选用水样"() -> (w710:enum16{"葡萄糖", "草酸钠"})
        n451 = case shown="\"葡萄糖\", 默认" w710 {
          tunnel: ["葡萄糖标线" ("section") "草酸钠标线" ("section")] -> w709
          frame "葡萄糖", Default {
          }
          frame "草酸钠" {
          }
        }
        n452 = case shown="\"0-2量程\"" "量程选择" {
          tunnel: ["低量程" "高量程" "0-2量程"] -> w706
          frame "低量程", Default {
          }
          frame "高量程" {
          }
          frame "0-2量程" {
          }
        }
        n453 = call <vilib>:"Application Directory.vi"() -> ("Application Directory"=w733:path)
        n454 = Build Path(base path=w733, name or relative path="data\\Set.ini" ("名称或相对路径")) -> (appended path=w731:path)
        n455 = call <vilib>:"Open Config Data.vi"("configuration file path"=w731) -> ("error out"=w734:errorcluster, "refnum"=w735:T6)  [unwired: 8 in, 1 out]
        n456 = Concatenate Strings(w709, w706) -> (w708:string)
        n457 = call-poly <vilib>:"Read Key.vi"("section"=w708, "error in (no error)"=w734, "key"="浓度1", "refnum"=w735) -> ("error out"=w739:errorcluster, "value"=w737:dbl, "refnum out"=w738:T6)  [unwired: 4 in, 1 out]
        n458 = local write "浓度1"(w737) -> ()
        n459 = call-poly <vilib>:"Read Key.vi"("section"=w708, "error in (no error)"=w739, "key"="浓度2", "refnum"=w738) -> ("error out"=w753:errorcluster, "value"=w740:dbl, "refnum out"=w752:T6)  [unwired: 4 in, 1 out]
        n460 = local write "浓度2"(w740) -> ()
        n461 = call-poly <vilib>:"Read Key.vi"("section"=w708, "error in (no error)"=w753, "key"="浓度3", "refnum"=w752) -> ("error out"=w754:errorcluster, "value"=w742:dbl, "refnum out"=w751:T6)  [unwired: 4 in, 1 out]
        n462 = local write "浓度3"(w742) -> ()
        n463 = call-poly <vilib>:"Read Key.vi"("section"=w708, "error in (no error)"=w754, "key"="泵滴定数1", "refnum"=w751) -> ("error out"=w755:errorcluster, "value"=w744:dbl, "refnum out"=w750:T6)  [unwired: 4 in, 1 out]
        n464 = local write "泵滴定数1"(w744) -> ()
        n465 = call-poly <vilib>:"Read Key.vi"("section"=w708, "error in (no error)"=w755, "key"="泵滴定数2", "refnum"=w750) -> ("error out"=w749:errorcluster, "value"=w747:dbl, "refnum out"=w756:T6)  [unwired: 4 in, 1 out]
        n466 = local write "泵滴定数2"(w747) -> ()
        n467 = call-poly <vilib>:"Read Key.vi"("section"=w708, "error in (no error)"=w749, "key"="泵滴定数3", "refnum"=w756) -> ("error out"=w761:errorcluster, "value"=w760:dbl, "refnum out"=w757:T6)  [unwired: 4 in, 1 out]
        n468 = local write "泵滴定数3"(w760) -> ()
        n469 = call-poly <vilib>:"Read Key.vi"("section"=w708, "error in (no error)"=w761, "key"="浓度4", "refnum"=w757) -> ("error out"=w762:errorcluster, "value"=w697:dbl, "refnum out"=w758:T6)  [unwired: 4 in, 1 out]
        n470 = local write "浓度4"(w697) -> ()
        n471 = call-poly <vilib>:"Read Key.vi"("section"=w708, "error in (no error)"=w762, "key"="浓度5", "refnum"=w758) -> ("error out"=w704:errorcluster, "value"=w696:dbl, "refnum out"=w705:T6)  [unwired: 4 in, 1 out]
        n472 = local write "浓度5"(w696) -> ()
        n473 = call-poly <vilib>:"Read Key.vi"("section"=w708, "error in (no error)"=w704, "key"="泵滴定数4", "refnum"=w705) -> ("error out"=w763:errorcluster, "value"=w695:dbl, "refnum out"=w759:T6)  [unwired: 4 in, 1 out]
        n474 = local write "泵滴定数4"(w695) -> ()
        n475 = call-poly <vilib>:"Read Key.vi"("section"=w708, "error in (no error)"=w763, "key"="泵滴定数5", "refnum"=w759) -> ("error out"=w702:errorcluster, "value"=w694:dbl, "refnum out"=w703:T6)  [unwired: 4 in, 1 out]
        n476 = local write "泵滴定数5"(w694) -> ()
        n477 = call-poly <vilib>:"Read Key.vi"("section"=w708, "error in (no error)"=w702, "key"="当前选用的校准", "refnum"=w703) -> ("error out"=w727:errorcluster, "value"=w729:i32, "refnum out"=w728:T6)  [unwired: 4 in, 1 out]
        n478 = local write "当前校准"(w729) -> ()
        n479 = call-poly <vilib>:"Read Key.vi"("section"=w708, "error in (no error)"=w727, "key"="启用1", "refnum"=w728) -> ("error out"=w724:errorcluster, "value"=w713:bool, "refnum out"=w725:T6)  [unwired: 4 in, 1 out]
        n480 = local write "启用1"(w713) -> ()
        n481 = call-poly <vilib>:"Read Key.vi"("section"=w708, "error in (no error)"=w724, "key"="启用2", "refnum"=w725) -> ("error out"=w722:errorcluster, "value"=w712:bool, "refnum out"=w723:T6)  [unwired: 4 in, 1 out]
        n482 = local write "启用2"(w712) -> ()
        n483 = call-poly <vilib>:"Read Key.vi"("section"=w708, "error in (no error)"=w722, "key"="启用3", "refnum"=w723) -> ("error out"=w720:errorcluster, "value"=w711:bool, "refnum out"=w721:T6)  [unwired: 4 in, 1 out]
        n484 = local write "启用3"(w711) -> ()
        n485 = call-poly <vilib>:"Read Key.vi"("section"=w708, "error in (no error)"=w720, "key"="启用4", "refnum"=w721) -> ("error out"=w718:errorcluster, "value"=w699:bool, "refnum out"=w719:T6)  [unwired: 4 in, 1 out]
        n486 = local write "启用4"(w699) -> ()
        n487 = call-poly <vilib>:"Read Key.vi"("section"=w708, "error in (no error)"=w718, "key"="启用5", "refnum"=w719) -> ("error out"=w700:errorcluster, "value"=w698:bool, "refnum out"=w701:T6)  [unwired: 4 in, 1 out]
        n488 = local write "启用5"(w698) -> ()
        n489 = call <vilib>:"Close Config Data.vi"("error in (no error)"=w700, "refnum"=w701) -> ()  [unwired: 8 in, 2 out]
      }
      event "周期设置": Value Change {
        n490 = event-data() -> ()  [unwired: 1 in, 6 out]
        n491 = call "数字密码键盘.vi"() -> ("NewNumber"=w774:sgl)  [unwired: 1 in]
        n492 = Equal?(x=w774, y=8.0) -> (x = y?=w775:bool)
        n493 = case shown="真" w775 {
          frame False {
            n494 = call "窗口弹出对话框(子VI).vi"("消息"="密码错误") -> ()  [unwired: 10 in, 1 out]
          }
          frame True {
            n495 = call "窗口弹出对话框(子VI).vi"("消息"="登录成功") -> ("true"=w778:bool)  [unwired: 10 in]
            n496 = case shown="真" w778 {
              frame False {
              }
              frame True {
                n497 = property on="窗格" class="Pane"("Origin"=T13 {"Horizontal"=0, "Vertical"=1950} ("原点")) -> ()  [unwired: 2 in, 2 out]
              }
            }
          }
        }
      }
      event "返回": Value Change {
        (unwired) "泵滴定数6" ("key")
        w794 = "CODMn" ("section")
        n498 = event-data() -> ()  [unwired: 1 in, 6 out]
        n499 = property on="窗格" class="Pane"("Origin"=T13 {"Horizontal"=0, "Vertical"=0} ("原点")) -> ()  [unwired: 2 in, 2 out]
        n500 = call <vilib>:"Application Directory.vi"() -> ("Application Directory"=w847:path)
        n501 = Build Path(base path=w847, name or relative path="data\\Set.ini" ("名称或相对路径")) -> (appended path=w845:path)
        n502 = local write "读取KB值"(FALSE ("读取KB值")) -> ()
        n503 = call <vilib>:"Open Config Data.vi"("configuration file path"=w845) -> ("error out"=w843:errorcluster, "refnum"=w844:T6)  [unwired: 8 in, 1 out]
        n504 = local read "浓度1"() -> (w841:dbl)
        n505 = local read "浓度2"() -> (w825:dbl)
        n506 = call-poly <vilib>:"Write Key.vi"("section"=w794, "error in (no error)"=w843, "value"=w841, "key"="浓度1", "refnum"=w844) -> ("error out"=w840:errorcluster, "refnum out"=w839:T6)  [unwired: 4 in, 1 out]
        n507 = local read "浓度3"() -> (w821:dbl)
        n508 = call-poly <vilib>:"Write Key.vi"("section"=w794, "error in (no error)"=w840, "value"=w825, "key"="浓度2", "refnum"=w839) -> ("error out"=w838:errorcluster, "refnum out"=w837:T6)  [unwired: 4 in, 1 out]
        n509 = local read "泵滴定数1"() -> (w819:dbl)
        n510 = call-poly <vilib>:"Write Key.vi"("section"=w794, "error in (no error)"=w838, "value"=w821, "key"="浓度3", "refnum"=w837) -> ("error out"=w836:errorcluster, "refnum out"=w835:T6)  [unwired: 4 in, 1 out]
        n511 = call-poly <vilib>:"Write Key.vi"("section"=w794, "error in (no error)"=w836, "value"=w819, "key"="泵滴定数1", "refnum"=w835) -> ("error out"=w834:errorcluster, "refnum out"=w833:T6)  [unwired: 4 in, 1 out]
        n512 = local read "泵滴定数2"() -> (w817:dbl)
        n513 = call-poly <vilib>:"Write Key.vi"("section"=w794, "error in (no error)"=w834, "value"=w817, "key"="泵滴定数2", "refnum"=w833) -> ("error out"=w832:errorcluster, "refnum out"=w831:T6)  [unwired: 4 in, 1 out]
        n514 = local read "泵滴定数3"() -> (w815:dbl)
        n515 = local read "浓度4"() -> (w782:dbl)
        n516 = call-poly <vilib>:"Write Key.vi"("section"=w794, "error in (no error)"=w832, "value"=w815, "key"="泵滴定数3", "refnum"=w831) -> ("error out"=w830:errorcluster, "refnum out"=w829:T6)  [unwired: 4 in, 1 out]
        n517 = call-poly <vilib>:"Write Key.vi"("section"=w794, "error in (no error)"=w830, "value"=w782, "key"="浓度4", "refnum"=w829) -> ("error out"=w823:errorcluster, "refnum out"=w824:T6)  [unwired: 4 in, 1 out]
        n518 = local read "浓度5"() -> (w781:dbl)
        n519 = call-poly <vilib>:"Write Key.vi"("section"=w794, "error in (no error)"=w823, "value"=w781, "key"="浓度5", "refnum"=w824) -> ("error out"=w791:errorcluster, "refnum out"=w792:T6)  [unwired: 4 in, 1 out]
        n520 = local read "泵滴定数4"() -> (w783:dbl)
        n521 = call-poly <vilib>:"Write Key.vi"("section"=w794, "error in (no error)"=w791, "value"=w783, "key"="泵滴定数4", "refnum"=w792) -> ("error out"=w828:errorcluster, "refnum out"=w827:T6)  [unwired: 4 in, 1 out]
        n522 = local read "泵滴定数5"() -> (w784:dbl)
        n523 = call-poly <vilib>:"Write Key.vi"("section"=w794, "error in (no error)"=w828, "value"=w784, "key"="泵滴定数5", "refnum"=w827) -> ("error out"=w789:errorcluster, "refnum out"=w790:T6)  [unwired: 4 in, 1 out]
        n524 = local read "启用1"() -> (w803:bool)
        n525 = call-poly <vilib>:"Write Key.vi"("section"=w794, "error in (no error)"=w789, "value"=w803, "key"="启用1", "refnum"=w790) -> ("error out"=w799:errorcluster, "refnum out"=w802:T6)  [unwired: 4 in, 1 out]
        n526 = local read "启用2"() -> (w800:bool)
        n527 = call-poly <vilib>:"Write Key.vi"("section"=w794, "error in (no error)"=w799, "value"=w800, "key"="启用2", "refnum"=w802) -> ("error out"=w810:errorcluster, "refnum out"=w809:T6)  [unwired: 4 in, 1 out]
        n528 = local read "启用3"() -> (w798:bool)
        n529 = call-poly <vilib>:"Write Key.vi"("section"=w794, "error in (no error)"=w810, "value"=w798, "key"="启用3", "refnum"=w809) -> ("error out"=w808:errorcluster, "refnum out"=w807:T6)  [unwired: 4 in, 1 out]
        n530 = local read "启用4"() -> (w786:bool)
        n531 = call-poly <vilib>:"Write Key.vi"("section"=w794, "error in (no error)"=w808, "value"=w786, "key"="启用4", "refnum"=w807) -> ("error out"=w806:errorcluster, "refnum out"=w805:T6)  [unwired: 4 in, 1 out]
        n532 = local read "启用5"() -> (w785:bool)
        n533 = call-poly <vilib>:"Write Key.vi"("section"=w794, "error in (no error)"=w806, "value"=w785, "key"="启用5", "refnum"=w805) -> ("error out"=w787:errorcluster, "refnum out"=w788:T6)  [unwired: 4 in, 1 out]
        n534 = call <vilib>:"Close Config Data.vi"("error in (no error)"=w787, "refnum"=w788) -> ()  [unwired: 8 in, 2 out]
      }
      event "关闭", "关闭 2", "关闭 3": Value Change {
        n535 = event-data() -> ()  [unwired: 1 in, 6 out]
        n536 = property on="窗格" class="Pane"("Origin"=T13 {"Horizontal"=0, "Vertical"=0} ("原点")) -> ()  [unwired: 2 in, 2 out]
      }
      event Application Instance Close {
        n537 = event-data() -> ()  [unwired: 1 in, 4 out]
        n538 = call-dynamic "Close Session.vi"("error in (no error)"=w850, "MB_Serial session"=w851) -> ()  [unwired: 9 in, 1 out]
      }
      event "时间校准": Value Change {
        n539 = event-data() -> ()  [unwired: 1 in, 6 out]
        n540 = flat-sequence {
          tunnel: w852 -> [w857]
          frame #0 {
            n541 = Get Date/Time In Seconds() -> (seconds since 1Jan1904=w862:timestamp)
            n542 = Build Array(w862) -> (w861:timestamp[])
            n543 = call "DateToHex.vi"("DATE"=w861) -> ("数组"=w855:u16[])  [unwired: 10 in]
            n544 = Insert Into Array(array=u16[] [1] ("values"), index=1 ("索引"), new element=w855) -> (w853:u16[])
            n545 = Bundle By Name(cluster=cluster{"starting address":u16, "values":u16[]} {"starting address"=0, "values"=[]}, "starting address"=u16 4612, "values"=w853) -> (w858:cluster{"starting address":u16, "values":u16[]})
            n546 = Enqueue Element(queue=w857, element=w858) -> ()  [unwired: 2 in, 3 out]
          }
          frame #1 {
            n547 = local write "枚举"(enum16{"读取数据", "写入数据", "读取写入DATABASE", "读取参数"}."写入数据" ("枚举")) -> ()
          }
        }
      }
      event "故障清除": Value Change {
        n548 = event-data() -> ()  [unwired: 1 in, 6 out]
        n549 = local write "枚举"(enum16{"读取数据", "写入数据", "读取写入DATABASE", "读取参数"}."写入数据" ("枚举")) -> ()
        n550 = Bundle By Name(cluster=cluster{"starting address":u16, "values":u16[]} {"starting address"=0, "values"=[]}, "starting address"=u16 4611, "values"=u16[] [1]) -> (w867:cluster{"starting address":u16, "values":u16[]})
        n551 = Enqueue Element(queue=w866, element=w867) -> ()  [unwired: 2 in, 3 out]
      }
      event "定时启动": Mouse Down {
        n552 = event-data() -> ()  [unwired: 1 in, 8 out]
        n553 = flat-sequence {
          frame #0 {
            n554 = global read "CODMn断电保存全局变量.vi" "定时控制"() -> (w870:T8)
            n555 = call "周期设置.vi"("定时控制参数输入"=w870) -> ("定时控制参数输出"=w871:T8)  [unwired: 10 in]
            n556 = global write "CODMn断电保存全局变量.vi" "定时控制"(w871) -> ()
          }
          frame #1 {
            n557 = call <vilib>:"Application Directory.vi"() -> ("Application Directory"=w885:path)
            n558 = Build Path(base path=w885, name or relative path="data\\sys.ini" ("名称或相对路径")) -> (appended path=w883:path)
            n559 = call <vilib>:"Open Config Data.vi"("configuration file path"=w883) -> ("error out"=w879:errorcluster, "refnum"=w882:T6)  [unwired: 8 in, 1 out]
            n560 = vi-ref "斯坦道CODMn.lvlib:CODMn断电保存全局变量.vi"() -> (w881:refnum<vi>)
            n561 = call <userlib>:"Write Panel to INI__ogtk.vi"("error in (no error)"=w879, "VI ref"=w881, "refnum"=w882) -> ("error out"=w878:errorcluster, "refnum out"=w880:T6)  [unwired: 7 in]
            n562 = call <vilib>:"Close Config Data.vi"("error in (no error)"=w878, "refnum"=w880) -> ("error out"=w873:errorcluster, "file path"=w872:path)  [unwired: 8 in]
            n563 = Open/Create/Replace File(file path (use dialog)=w872, error in=w873) -> (refnum out=w876:refnum<file>, error out=w877:errorcluster)  [unwired: 4 in, 1 out]
            n564 = Flush File(refnum=w876, error in=w877) -> (refnum out=w875:refnum<file>, error out=w874:errorcluster)
            n565 = Close File(refnum=w875, error in=w874) -> ()  [unwired: 2 out]
          }
        }
      }
      event "测量模式(公式)": Value Change {
        n566 = event-data() -> ()  [unwired: 1 in, 6 out]
        n567 = flat-sequence {
          frame #0 {
            n568 = local read "测量模式(公式)"() -> (w886:u16)
            n569 = global write "CODMn断电保存全局变量.vi" "测量模式(公式)"(w886) -> ()
          }
          frame #1 {
            n570 = call <vilib>:"Application Directory.vi"() -> ("Application Directory"=w900:path)
            n571 = Build Path(base path=w900, name or relative path="data\\sys.ini" ("名称或相对路径")) -> (appended path=w898:path)
            n572 = call <vilib>:"Open Config Data.vi"("configuration file path"=w898) -> ("error out"=w894:errorcluster, "refnum"=w897:T6)  [unwired: 8 in, 1 out]
            n573 = vi-ref "斯坦道CODMn.lvlib:CODMn断电保存全局变量.vi"() -> (w896:refnum<vi>)
            n574 = call <userlib>:"Write Panel to INI__ogtk.vi"("error in (no error)"=w894, "VI ref"=w896, "refnum"=w897) -> ("error out"=w893:errorcluster, "refnum out"=w895:T6)  [unwired: 7 in]
            n575 = call <vilib>:"Close Config Data.vi"("error in (no error)"=w893, "refnum"=w895) -> ("error out"=w888:errorcluster, "file path"=w887:path)  [unwired: 8 in]
            n576 = Open/Create/Replace File(file path (use dialog)=w887, error in=w888) -> (refnum out=w891:refnum<file>, error out=w892:errorcluster)  [unwired: 4 in, 1 out]
            n577 = Flush File(refnum=w891, error in=w892) -> (refnum out=w890:refnum<file>, error out=w889:errorcluster)
            n578 = Close File(refnum=w890, error in=w889) -> ()  [unwired: 2 out]
          }
        }
      }
      event "CODMn跨度量程选择": Value Change {
        n579 = event-data() -> ()  [unwired: 1 in, 6 out]
        n580 = flat-sequence {
          frame #0 {
            n581 = global write "CODMn断电保存全局变量.vi" "CODMn跨度量程选择"("CODMn跨度量程选择") -> ()
          }
          frame #1 {
            n582 = call <vilib>:"Application Directory.vi"() -> ("Application Directory"=w915:path)
            n583 = Build Path(base path=w915, name or relative path="data\\sys.ini" ("名称或相对路径")) -> (appended path=w913:path)
            n584 = call <vilib>:"Open Config Data.vi"("configuration file path"=w913) -> ("error out"=w909:errorcluster, "refnum"=w912:T6)  [unwired: 8 in, 1 out]
            n585 = vi-ref "斯坦道CODMn.lvlib:CODMn断电保存全局变量.vi"() -> (w911:refnum<vi>)
            n586 = call <userlib>:"Write Panel to INI__ogtk.vi"("error in (no error)"=w909, "VI ref"=w911, "refnum"=w912) -> ("error out"=w908:errorcluster, "refnum out"=w910:T6)  [unwired: 7 in]
            n587 = call <vilib>:"Close Config Data.vi"("error in (no error)"=w908, "refnum"=w910) -> ("error out"=w903:errorcluster, "file path"=w902:path)  [unwired: 8 in]
            n588 = Open/Create/Replace File(file path (use dialog)=w902, error in=w903) -> (refnum out=w906:refnum<file>, error out=w907:errorcluster)  [unwired: 4 in, 1 out]
            n589 = Flush File(refnum=w906, error in=w907) -> (refnum out=w905:refnum<file>, error out=w904:errorcluster)
            n590 = Close File(refnum=w905, error in=w904) -> ()  [unwired: 2 out]
          }
        }
      }
      event "CODMn零点核查选择": Value Change {
        n591 = event-data() -> ()  [unwired: 1 in, 6 out]
        n592 = global write "CODMn断电保存全局变量.vi" "CODMn零点核查选择"("CODMn零点核查选择") -> ()
      }
      event "校准1", "校准2", "校准3", "校准4", "校准5": Value Change {
        n593 = event-data() -> ()  [unwired: 1 in, 6 out]
        n594 = flat-sequence {
          tunnel: w919 -> [w924]
          tunnel: [w923] -> w918
          tunnel: [w922] -> w917
          tunnel: w918 -> [w958]
          tunnel: w917 -> [w957]
          frame #0 {
            n595 = Build Array("校准1", "校准2", "校准3", "校准4", "校准5") -> (w925:bool[])
            n596 = for {
              tunnel: w925 -> [w939] mode=indexing
              tunnel: w924 -> [w935]
              tunnel: [w931] -> w923
              tunnel: [w930] -> w922
              i -> [w929]
              n597 = case shown="4" w929 {
                tunnel: ["浓度1" "浓度2" "浓度3" "浓度4" "浓度5"] -> w934
                frame 0, Default {
                }
                frame 1 {
                }
                frame 2 {
                }
                frame 3 {
                }
                frame 4 {
                }
              }
              n598 = Multiply(x=w934, y=100.0) -> (x*y=w932:dbl)
              n599 = Insert Into Array(array=u16[] [] ("values"), index=0 ("索引"), new element=w932) -> (w936:u16[])
              n600 = case shown="真" w939 {
                tunnel: w936 -> [_ w951]
                tunnel: w935 -> [w945 w950]
                tunnel: [w945 w949] -> w931
                tunnel: [_ w948] -> w930
                tunnel: w929 -> [_ w947]
                frame False {
                }
                frame True {
                  n601 = Increment(x=w947) -> (x+1=→"当前校准":i32)
                  n602 = Bundle By Name(cluster=cluster{"starting address":u16, "values":u16[]} {"starting address"=4272, "values"=[]}, "starting address"=u16 4274, "values"=w951) -> (w953:cluster{"starting address":u16, "values":u16[]})
                  n603 = Enqueue Element(queue=w950, element=w953) -> (queue out=w949:refnum<queue>, error out=w948:errorcluster)  [unwired: 2 in, 1 out]
                }
              }
            }
          }
          frame #1 {
            n604 = local read "当前校准"() -> (w962:i32)
            n605 = case shown="5" w962 {
              tunnel: [w968 w969 w970 w971 w972] -> w961
              frame 1, Default {
                n606 = local read "浓度1"() -> (w968:dbl)
              }
              frame 2 {
                n607 = local read "浓度2"() -> (w969:dbl)
              }
              frame 3 {
                n608 = local read "浓度3"() -> (w970:dbl)
              }
              frame 4 {
                n609 = local read "浓度4"() -> (w971:dbl)
              }
              frame 5 {
                n610 = local read "浓度5"() -> (w972:dbl)
              }
            }
            n611 = Not Equal To 0?(x=w961) -> (x != 0?=w955:bool)
            n612 = case shown="假" w955 {
              tunnel: [u16 8 ("address") u16 9 ("address")] -> w965
              tunnel: ["校零" ("测量模式") "校标" ("测量模式")] -> w956
              frame False {
              }
              frame True {
              }
            }
            n613 = global write "COD测量模式全局.vi" "测量模式"(w956) -> ()
            n614 = Insert Into Array(array=u16[] [] ("values"), index=0 ("索引"), new element=w965) -> (w960:u16[])
            n615 = Bundle By Name(cluster=cluster{"starting address":u16, "values":u16[]} {"starting address"=0, "values"=[]}, "starting address"=u16 4608 ("address"), "values"=w960) -> (w967:cluster{"starting address":u16, "values":u16[]})
            n616 = Enqueue Element(queue=w958, element=w967, error in (no error)=w957) -> ()  [unwired: 1 in, 3 out]
          }
          frame #2 {
            n617 = local write "枚举"(enum16{"读取数据", "写入数据", "读取写入DATABASE", "读取参数"}."写入数据" ("枚举")) -> ()
            n618 = call <vilib>:"Application Directory.vi"() -> ("Application Directory"=w984:path)
            n619 = Build Path(base path=w984, name or relative path="data\\Set.ini" ("名称或相对路径")) -> (appended path=w986:path)
            n620 = local read "当前校准"() -> (w979:i32)
            n621 = call <vilib>:"Open Config Data.vi"("configuration file path"=w986) -> ("error out"=w982:errorcluster, "refnum"=w983:T6)  [unwired: 8 in, 1 out]
            n622 = call-poly <vilib>:"Write Key.vi"("section"="CODMn", "error in (no error)"=w982, "value"=w979, "key"="当前选用的校准" ("section"), "refnum"=w983) -> ("error out"=w977:errorcluster, "refnum out"=w978:T6)  [unwired: 4 in, 1 out]
            n623 = call <vilib>:"Close Config Data.vi"("error in (no error)"=w977, "refnum"=w978) -> ()  [unwired: 8 in, 2 out]
          }
        }
      }
      event "自动切换量程:", "低切高阈值:", "高切低阈值:": Value Change {
        n624 = event-data() -> ()  [unwired: 1 in, 6 out]
        n625 = flat-sequence {
          frame #0 {
            n626 = local read "自动切换量程:"() -> (w990:enum16{"关闭", "自动切换测一次", "自动切换测两次"})
            n627 = local read "低切高阈值:"() -> (w989:dbl)
            n628 = local read "高切低阈值:"() -> (w988:dbl)
            n629 = global write "CODMn断电保存全局变量.vi" "自动切换量程:"(w990) -> ()
            n630 = global write "CODMn断电保存全局变量.vi" "低切高阈值:"(w989) -> ()
            n631 = global write "CODMn断电保存全局变量.vi" "高切低阈值:"(w988) -> ()
          }
          frame #1 {
            n632 = call <vilib>:"Application Directory.vi"() -> ("Application Directory"=w1004:path)
            n633 = Build Path(base path=w1004, name or relative path="data\\sys.ini" ("名称或相对路径")) -> (appended path=w1002:path)
            n634 = call <vilib>:"Open Config Data.vi"("configuration file path"=w1002) -> ("error out"=w998:errorcluster, "refnum"=w1001:T6)  [unwired: 8 in, 1 out]
            n635 = vi-ref "斯坦道CODMn.lvlib:CODMn断电保存全局变量.vi"() -> (w1000:refnum<vi>)
            n636 = call <userlib>:"Write Panel to INI__ogtk.vi"("error in (no error)"=w998, "VI ref"=w1000, "refnum"=w1001) -> ("error out"=w997:errorcluster, "refnum out"=w999:T6)  [unwired: 7 in]
            n637 = call <vilib>:"Close Config Data.vi"("error in (no error)"=w997, "refnum"=w999) -> ("error out"=w992:errorcluster, "file path"=w991:path)  [unwired: 8 in]
            n638 = Open/Create/Replace File(file path (use dialog)=w991, error in=w992) -> (refnum out=w995:refnum<file>, error out=w996:errorcluster)  [unwired: 4 in, 1 out]
            n639 = Flush File(refnum=w995, error in=w996) -> (refnum out=w994:refnum<file>, error out=w993:errorcluster)
            n640 = Close File(refnum=w994, error in=w993) -> ()  [unwired: 2 out]
          }
        }
      }
      event "模型": Value Change {
        n641 = event-data() -> ()  [unwired: 1 in, 6 out]
        n642 = call <vilib>:"Application Directory.vi"() -> ("Application Directory"=w1014:path)
        n643 = Build Path(base path=w1014, name or relative path="data\\Set.ini" ("名称或相对路径")) -> (appended path=w1012:path)
        n644 = call <vilib>:"Open Config Data.vi"("configuration file path"=w1012) -> ("error out"=w1010:errorcluster, "refnum"=w1011:T6)  [unwired: 8 in, 1 out]
        n645 = local read "模型"() -> (w1005:enum32{"线性", "多项式"})
        n646 = call-poly <vilib>:"Write Key.vi"("section"="CODMn模型选择" ("key"), "error in (no error)"=w1010, "value"=w1005, "key"="线性和多项式", "refnum"=w1011) -> ("error out"=w1006:errorcluster, "refnum out"=w1007:T6)  [unwired: 4 in, 1 out]
        n647 = call <vilib>:"Close Config Data.vi"("error in (no error)"=w1006, "refnum"=w1007) -> ()  [unwired: 8 in, 2 out]
      }
      event "浓度1", "浓度2", "浓度3", "泵滴定数1", "泵滴定数2", "泵滴定数3", "启用1", "启用2", "启用3", "浓度4", "浓度5", "泵滴定数4", "泵滴定数5", "启用4", "启用5": Value Change {
        n648 = event-data() -> ()  [unwired: 1 in, 6 out]
        n649 = local read "选用水样"() -> (w1030:enum16{"葡萄糖", "草酸钠"})
        n650 = local read "量程选择"() -> (w1029:enum16{"低量程", "高量程", "0-2量程"})
        n651 = case shown="\"0-2量程\"" w1029 {
          tunnel: ["低量程" "高量程" "0-2量程"] -> w1027
          frame "低量程", Default {
          }
          frame "高量程" {
          }
          frame "0-2量程" {
          }
        }
        n652 = call <vilib>:"Application Directory.vi"() -> ("Application Directory"=w1089:path)
        n653 = case shown="\"葡萄糖\", 默认" w1030 {
          tunnel: ["葡萄糖标线" ("section") "草酸钠标线" ("section")] -> w1036
          frame "葡萄糖", Default {
          }
          frame "草酸钠" {
          }
        }
        n654 = Build Path(base path=w1089, name or relative path="data\\Set.ini" ("名称或相对路径")) -> (appended path=w1087:path)
        n655 = call <vilib>:"Open Config Data.vi"("configuration file path"=w1087) -> ("error out"=w1085:errorcluster, "refnum"=w1086:T6)  [unwired: 8 in, 1 out]
        n656 = local read "浓度1"() -> (w1083:dbl)
        n657 = Concatenate Strings(w1036, w1027) -> (w1028:string)
        n658 = local read "浓度2"() -> (w1067:dbl)
        n659 = call-poly <vilib>:"Write Key.vi"("section"=w1028, "error in (no error)"=w1085, "value"=w1083, "key"="浓度1", "refnum"=w1086) -> ("error out"=w1082:errorcluster, "refnum out"=w1081:T6)  [unwired: 4 in, 1 out]
        n660 = local read "浓度3"() -> (w1063:dbl)
        n661 = call-poly <vilib>:"Write Key.vi"("section"=w1028, "error in (no error)"=w1082, "value"=w1067, "key"="浓度2", "refnum"=w1081) -> ("error out"=w1080:errorcluster, "refnum out"=w1079:T6)  [unwired: 4 in, 1 out]
        n662 = local read "泵滴定数1"() -> (w1061:dbl)
        n663 = call-poly <vilib>:"Write Key.vi"("section"=w1028, "error in (no error)"=w1080, "value"=w1063, "key"="浓度3", "refnum"=w1079) -> ("error out"=w1078:errorcluster, "refnum out"=w1077:T6)  [unwired: 4 in, 1 out]
        n664 = call-poly <vilib>:"Write Key.vi"("section"=w1028, "error in (no error)"=w1078, "value"=w1061, "key"="泵滴定数1", "refnum"=w1077) -> ("error out"=w1076:errorcluster, "refnum out"=w1075:T6)  [unwired: 4 in, 1 out]
        n665 = local read "泵滴定数2"() -> (w1059:dbl)
        n666 = call-poly <vilib>:"Write Key.vi"("section"=w1028, "error in (no error)"=w1076, "value"=w1059, "key"="泵滴定数2", "refnum"=w1075) -> ("error out"=w1074:errorcluster, "refnum out"=w1073:T6)  [unwired: 4 in, 1 out]
        n667 = local read "泵滴定数3"() -> (w1057:dbl)
        n668 = local read "浓度4"() -> (w1026:dbl)
        n669 = call-poly <vilib>:"Write Key.vi"("section"=w1028, "error in (no error)"=w1074, "value"=w1057, "key"="泵滴定数3", "refnum"=w1073) -> ("error out"=w1072:errorcluster, "refnum out"=w1071:T6)  [unwired: 4 in, 1 out]
        n670 = local read "浓度5"() -> (w1025:dbl)
        n671 = call-poly <vilib>:"Write Key.vi"("section"=w1028, "error in (no error)"=w1072, "value"=w1026, "key"="浓度4", "refnum"=w1071) -> ("error out"=w1065:errorcluster, "refnum out"=w1066:T6)  [unwired: 4 in, 1 out]
        n672 = call-poly <vilib>:"Write Key.vi"("section"=w1028, "error in (no error)"=w1065, "value"=w1025, "key"="浓度5", "refnum"=w1066) -> ("error out"=w1023:errorcluster, "refnum out"=w1024:T6)  [unwired: 4 in, 1 out]
        n673 = local read "泵滴定数4"() -> (w1022:dbl)
        n674 = call-poly <vilib>:"Write Key.vi"("section"=w1028, "error in (no error)"=w1023, "value"=w1022, "key"="泵滴定数4", "refnum"=w1024) -> ("error out"=w1070:errorcluster, "refnum out"=w1069:T6)  [unwired: 4 in, 1 out]
        n675 = local read "泵滴定数5"() -> (w1021:dbl)
        n676 = call-poly <vilib>:"Write Key.vi"("section"=w1028, "error in (no error)"=w1070, "value"=w1021, "key"="泵滴定数5", "refnum"=w1069) -> ("error out"=w1019:errorcluster, "refnum out"=w1020:T6)  [unwired: 4 in, 1 out]
        n677 = local read "启用1"() -> (w1045:bool)
        n678 = call-poly <vilib>:"Write Key.vi"("section"=w1028, "error in (no error)"=w1019, "value"=w1045, "key"="启用1", "refnum"=w1020) -> ("error out"=w1041:errorcluster, "refnum out"=w1044:T6)  [unwired: 4 in, 1 out]
        n679 = local read "启用2"() -> (w1042:bool)
        n680 = call-poly <vilib>:"Write Key.vi"("section"=w1028, "error in (no error)"=w1041, "value"=w1042, "key"="启用2", "refnum"=w1044) -> ("error out"=w1052:errorcluster, "refnum out"=w1051:T6)  [unwired: 4 in, 1 out]
        n681 = local read "启用3"() -> (w1040:bool)
        n682 = call-poly <vilib>:"Write Key.vi"("section"=w1028, "error in (no error)"=w1052, "value"=w1040, "key"="启用3", "refnum"=w1051) -> ("error out"=w1050:errorcluster, "refnum out"=w1049:T6)  [unwired: 4 in, 1 out]
        n683 = local read "启用4"() -> (w1015:bool)
        n684 = call-poly <vilib>:"Write Key.vi"("section"=w1028, "error in (no error)"=w1050, "value"=w1015, "key"="启用4", "refnum"=w1049) -> ("error out"=w1048:errorcluster, "refnum out"=w1047:T6)  [unwired: 4 in, 1 out]
        n685 = local read "启用5"() -> (w1016:bool)
        n686 = call-poly <vilib>:"Write Key.vi"("section"=w1028, "error in (no error)"=w1048, "value"=w1016, "key"="启用5", "refnum"=w1047) -> ("error out"=w1017:errorcluster, "refnum out"=w1018:T6)  [unwired: 4 in, 1 out]
        n687 = local read "选用水样"() -> (w1035:enum16{"葡萄糖", "草酸钠"})
        n688 = call-poly <vilib>:"Write Key.vi"("section"="标线选择", "error in (no error)"=w1017, "value"=w1035, "key"="选用水样", "refnum"=w1018) -> ("error out"=w1032:errorcluster, "refnum out"=w1033:T6)  [unwired: 4 in, 1 out]
        n689 = call <vilib>:"Close Config Data.vi"("error in (no error)"=w1032, "refnum"=w1033) -> ()  [unwired: 8 in, 2 out]
      }
      event "读取": Value Change {
        n690 = event-data() -> ()  [unwired: 1 in, 6 out]
        n691 = local write "枚举"(enum16{"读取数据", "写入数据", "读取写入DATABASE", "读取参数"}."读取参数" ("枚举")) -> ()
        n692 = Bundle By Name(cluster=T5 {"starting address"=0, "number of holding registers"=0}, "starting address"=u16 4616, "number of holding registers"=u16 94) -> (w1104:T5)
        n693 = Flush Queue(queue=w1097, error in (no error)=w1096) -> (queue out=w1100:refnum<queue>, error out=w1099:errorcluster)  [unwired: 1 out]
        n694 = Enqueue Element(queue=w1100, element=w1104, error in (no error)=w1099) -> ()  [unwired: 1 in, 3 out]
        "读取KB值" <- TRUE
      }
      event "写入": Mouse Down {
        n695 = event-data() -> ()  [unwired: 1 in, 8 out]
        n696 = flat-sequence {
          tunnel: w1105 -> [w1108]
          frame #0 {
            n697 = local read "模型"() -> (w1106:enum32{"线性", "多项式"})
            n698 = case shown="\"线性\", 默认" w1106 {
              tunnel: [w1120 w1160] -> w1110
              tunnel: w1108 -> [w1114 w1159]
              tunnel: [w1114 w1159] -> w1107
              frame "线性", Default {
                n699 = local read "测量模式(公式)"() -> (w1112:u16)
                n700 = case shown="7" w1112 {
                  tunnel: [u16 4626 ("starting address") w1123 w1128 w1133 w1138 w1143 w1148 w1153] -> w1111
                  frame 0, Default {
                  }
                  frame 1 {
                    n701 = local read "量程选择"() -> (w1122:enum16{"低量程", "高量程", "0-2量程"})
                    n702 = case shown="\"低量程\", 默认" w1122 {
                      tunnel: [u16 4626 ("starting address") u16 4632 ("starting address") u16 4638 ("starting address")] -> w1123
                      frame "低量程", Default {
                      }
                      frame "高量程" {
                      }
                      frame "0-2量程" {
                      }
                    }
                  }
                  frame 2 {
                    n703 = local read "量程选择"() -> (w1127:enum16{"低量程", "高量程", "0-2量程"})
                    n704 = case shown="\"低量程\", 默认" w1127 {
                      tunnel: [u16 4638 ("starting address") u16 4644 ("starting address") u16 4638 ("starting address")] -> w1128
                      frame "低量程", Default {
                      }
                      frame "高量程" {
                      }
                      frame "0-2量程" {
                      }
                    }
                  }
                  frame 3 {
                    n705 = local read "量程选择"() -> (w1132:enum16{"低量程", "高量程", "0-2量程"})
                    n706 = case shown="\"低量程\", 默认" w1132 {
                      tunnel: [u16 4650 ("starting address") u16 4656 ("starting address") u16 4638 ("starting address")] -> w1133
                      frame "低量程", Default {
                      }
                      frame "高量程" {
                      }
                      frame "0-2量程" {
                      }
                    }
                  }
                  frame 4 {
                    n707 = local read "量程选择"() -> (w1137:enum16{"低量程", "高量程", "0-2量程"})
                    n708 = case shown="\"低量程\", 默认" w1137 {
                      tunnel: [u16 4662 ("starting address") u16 4668 ("starting address") u16 4638 ("starting address")] -> w1138
                      frame "低量程", Default {
                      }
                      frame "高量程" {
                      }
                      frame "0-2量程" {
                      }
                    }
                  }
                  frame 5 {
                    n709 = local read "量程选择"() -> (w1142:enum16{"低量程", "高量程", "0-2量程"})
                    n710 = case shown="\"低量程\", 默认" w1142 {
                      tunnel: [u16 4674 ("starting address") u16 4680 ("starting address") u16 4638 ("starting address")] -> w1143
                      frame "低量程", Default {
                      }
                      frame "高量程" {
                      }
                      frame "0-2量程" {
                      }
                    }
                  }
                  frame 6 {
                    n711 = local read "量程选择"() -> (w1147:enum16{"低量程", "高量程", "0-2量程"})
                    n712 = case shown="\"低量程\", 默认" w1147 {
                      tunnel: [u16 4686 ("starting address") u16 4692 ("starting address") u16 4638 ("starting address")] -> w1148
                      frame "低量程", Default {
                      }
                      frame "高量程" {
                      }
                      frame "0-2量程" {
                      }
                    }
                  }
                  frame 7 {
                    n713 = local read "量程选择"() -> (w1152:enum16{"低量程", "高量程", "0-2量程"})
                    n714 = case shown="\"低量程\", 默认" w1152 {
                      tunnel: [u16 4698 ("starting address") u16 4704 ("starting address") u16 4638 ("starting address")] -> w1153
                      frame "低量程", Default {
                      }
                      frame "高量程" {
                      }
                      frame "0-2量程" {
                      }
                    }
                  }
                }
                n715 = local read "K"() -> (w1117:dbl)
                n716 = local read "b"() -> (w1116:dbl)
                n717 = Build Array(w1117, w1116, 0.0 ("元素")) -> (w1115:dbl[])
                n718 = call "浮点转CDAB整形cod.vi"("浮点数"=w1115) -> ("CDAB整形输出"=w1118:u16[])  [unwired: 10 in]
                n719 = Bundle By Name(cluster=cluster{"starting address":u16, "values":u16[]} {"starting address"=4272, "values"=[]}, "starting address"=w1111, "values"=w1118) -> (w1120:cluster{"starting address":u16, "values":u16[]})
              }
              frame "多项式" {
                # "b,k,c"
                n720 = local read "测量模式(公式)"() -> (w1157:u16)
                n721 = case shown="1" w1157 {
                  tunnel: [u16 4626 ("starting address") w1170 w1175 w1180 w1185 w1190 w1195 w1200] -> w1164
                  frame 0, Default {
                  }
                  frame 1 {
                    n722 = local read "量程选择"() -> (w1169:enum16{"低量程", "高量程", "0-2量程"})
                    n723 = case shown="\"低量程\", 默认" w1169 {
                      tunnel: [u16 4626 ("starting address") u16 4632 ("starting address") u16 4638 ("starting address")] -> w1170
                      frame "低量程", Default {
                      }
                      frame "高量程" {
                      }
                      frame "0-2量程" {
                      }
                    }
                  }
                  frame 2 {
                    n724 = local read "量程选择"() -> (w1174:enum16{"低量程", "高量程", "0-2量程"})
                    n725 = case shown="\"低量程\", 默认" w1174 {
                      tunnel: [u16 4638 ("starting address") u16 4644 ("starting address") u16 4638 ("starting address")] -> w1175
                      frame "低量程", Default {
                      }
                      frame "高量程" {
                      }
                      frame "0-2量程" {
                      }
                    }
                  }
                  frame 3 {
                    n726 = local read "量程选择"() -> (w1179:enum16{"低量程", "高量程", "0-2量程"})
                    n727 = case shown="\"低量程\", 默认" w1179 {
                      tunnel: [u16 4650 ("starting address") u16 4656 ("starting address") u16 4638 ("starting address")] -> w1180
                      frame "低量程", Default {
                      }
                      frame "高量程" {
                      }
                      frame "0-2量程" {
                      }
                    }
                  }
                  frame 4 {
                    n728 = local read "量程选择"() -> (w1184:enum16{"低量程", "高量程", "0-2量程"})
                    n729 = case shown="\"低量程\", 默认" w1184 {
                      tunnel: [u16 4662 ("starting address") u16 4668 ("starting address") u16 4638 ("starting address")] -> w1185
                      frame "低量程", Default {
                      }
                      frame "高量程" {
                      }
                      frame "0-2量程" {
                      }
                    }
                  }
                  frame 5 {
                    n730 = local read "量程选择"() -> (w1189:enum16{"低量程", "高量程", "0-2量程"})
                    n731 = case shown="\"低量程\", 默认" w1189 {
                      tunnel: [u16 4674 ("starting address") u16 4680 ("starting address") u16 4638 ("starting address")] -> w1190
                      frame "低量程", Default {
                      }
                      frame "高量程" {
                      }
                      frame "0-2量程" {
                      }
                    }
                  }
                  frame 6 {
                    n732 = local read "量程选择"() -> (w1194:enum16{"低量程", "高量程", "0-2量程"})
                    n733 = case shown="\"低量程\", 默认" w1194 {
                      tunnel: [u16 4686 ("starting address") u16 4692 ("starting address") u16 4638 ("starting address")] -> w1195
                      frame "低量程", Default {
                      }
                      frame "高量程" {
                      }
                      frame "0-2量程" {
                      }
                    }
                  }
                  frame 7 {
                    n734 = local read "量程选择"() -> (w1199:enum16{"低量程", "高量程", "0-2量程"})
                    n735 = case shown="\"低量程\", 默认" w1199 {
                      tunnel: [u16 4698 ("starting address") u16 4704 ("starting address") u16 4638 ("starting address")] -> w1200
                      frame "低量程", Default {
                      }
                      frame "高量程" {
                      }
                      frame "0-2量程" {
                      }
                    }
                  }
                }
                n736 = local read "多项式系数1"() -> (w1167:dbl[])
                n737 = Index Array(array=w1167) -> (element #1=w1162:dbl, element #2=w1163:dbl, element #3=w1158:dbl)  [unwired: 3 in]
                n738 = Build Array(w1163, w1162, w1158) -> (w1166:dbl[])
                n739 = call "浮点转CDAB整形cod.vi"("浮点数"=w1166) -> ("CDAB整形输出"=w1165:u16[])  [unwired: 10 in]
                n740 = Bundle By Name(cluster=cluster{"starting address":u16, "values":u16[]} {"starting address"=4272, "values"=[]}, "starting address"=w1164, "values"=w1165) -> (w1160:cluster{"starting address":u16, "values":u16[]})
              }
            }
            n741 = Enqueue Element(queue=w1107, element=w1110, timeout in ms (-1)=1000 ("超时毫秒(-1)")) -> ()  [unwired: 1 in, 3 out]
          }
          frame #1 {
            n742 = local write "枚举"(enum16{"读取数据", "写入数据", "读取写入DATABASE", "读取参数"}."写入数据" ("枚举")) -> ()
          }
        }
      }
      event "一键写入": Value Change {
        n743 = event-data() -> ()  [unwired: 1 in, 6 out]
        n744 = flat-sequence {
          tunnel: w1205 -> [w1207]
          frame #0 {
            n745 = local read "模型"() -> (w1206:enum32{"线性", "多项式"})
            n746 = case shown="\"线性\", 默认" w1206 {
              tunnel: w1207 -> [w1208 w1261]
              frame "线性", Default {
                n747 = property on="测量模式(公式)" class="Ring (严格)"() -> ("NumItems"=w1209:u32)  [unwired: 2 in, 2 out]
                n748 = for {
                  N: w1209 -> [_]
                  tunnel: w1208 -> [w1214]
                  i -> [w1212]
                  n749 = Increment(x=w1212) -> (x+1=w1211:i32)
                  n750 = local read "K"() -> (w1221:dbl)
                  n751 = case shown="1" w1211 {
                    tunnel: [u16 4626 ("starting address") w1227 w1232 w1237 w1242 w1247 w1252 w1257] -> w1210
                    frame 0, Default {
                    }
                    frame 1 {
                      n752 = local read "量程选择"() -> (w1226:enum16{"低量程", "高量程", "0-2量程"})
                      n753 = case shown="\"低量程\", 默认" w1226 {
                        tunnel: [u16 4626 ("starting address") u16 4632 ("starting address") u16 4638 ("starting address")] -> w1227
                        frame "低量程", Default {
                        }
                        frame "高量程" {
                        }
                        frame "0-2量程" {
                        }
                      }
                    }
                    frame 2 {
                      n754 = local read "量程选择"() -> (w1231:enum16{"低量程", "高量程", "0-2量程"})
                      n755 = case shown="\"低量程\", 默认" w1231 {
                        tunnel: [u16 4638 ("starting address") u16 4644 ("starting address") u16 4638 ("starting address")] -> w1232
                        frame "低量程", Default {
                        }
                        frame "高量程" {
                        }
                        frame "0-2量程" {
                        }
                      }
                    }
                    frame 3 {
                      n756 = local read "量程选择"() -> (w1236:enum16{"低量程", "高量程", "0-2量程"})
                      n757 = case shown="\"低量程\", 默认" w1236 {
                        tunnel: [u16 4650 ("starting address") u16 4656 ("starting address") u16 4638 ("starting address")] -> w1237
                        frame "低量程", Default {
                        }
                        frame "高量程" {
                        }
                        frame "0-2量程" {
                        }
                      }
                    }
                    frame 4 {
                      n758 = local read "量程选择"() -> (w1241:enum16{"低量程", "高量程", "0-2量程"})
                      n759 = case shown="\"高量程\"" w1241 {
                        tunnel: [u16 4662 ("starting address") u16 4668 ("starting address") u16 4638 ("starting address")] -> w1242
                        frame "低量程", Default {
                        }
                        frame "高量程" {
                        }
                        frame "0-2量程" {
                        }
                      }
                    }
                    frame 5 {
                      n760 = local read "量程选择"() -> (w1246:enum16{"低量程", "高量程", "0-2量程"})
                      n761 = case shown="\"低量程\", 默认" w1246 {
                        tunnel: [u16 4674 ("starting address") u16 4680 ("starting address") u16 4638 ("starting address")] -> w1247
                        frame "低量程", Default {
                        }
                        frame "高量程" {
                        }
                        frame "0-2量程" {
                        }
                      }
                    }
                    frame 6 {
                      n762 = local read "量程选择"() -> (w1251:enum16{"低量程", "高量程", "0-2量程"})
                      n763 = case shown="\"低量程\", 默认" w1251 {
                        tunnel: [u16 4686 ("starting address") u16 4692 ("starting address") u16 4638 ("starting address")] -> w1252
                        frame "低量程", Default {
                        }
                        frame "高量程" {
                        }
                        frame "0-2量程" {
                        }
                      }
                    }
                    frame 7 {
                      n764 = local read "量程选择"() -> (w1256:enum16{"低量程", "高量程", "0-2量程"})
                      n765 = case shown="\"低量程\", 默认" w1256 {
                        tunnel: [u16 4698 ("starting address") u16 4704 ("starting address") u16 4638 ("starting address")] -> w1257
                        frame "低量程", Default {
                        }
                        frame "高量程" {
                        }
                        frame "0-2量程" {
                        }
                      }
                    }
                  }
                  n766 = local read "b"() -> (w1222:dbl)
                  n767 = Build Array(w1221, w1222, 0.0 ("元素")) -> (w1223:dbl[])
                  n768 = call "浮点转CDAB整形cod.vi"("浮点数"=w1223) -> ("CDAB整形输出"=w1220:u16[])  [unwired: 10 in]
                  n769 = Insert Into Array(array=u16[] [], index=0 ("索引"), new element=w1220) -> (w1213:u16[])
                  n770 = Bundle By Name(cluster=cluster{"starting address":u16, "values":u16[]} {"starting address"=4272, "values"=[]}, "starting address"=w1210, "values"=w1213) -> (w1215:cluster{"starting address":u16, "values":u16[]})
                  n771 = Enqueue Element(queue=w1214, element=w1215, timeout in ms (-1)=1000 ("超时毫秒(-1)")) -> ()  [unwired: 1 in, 3 out]
                }
              }
              frame "多项式" {
                # "b,k,c"
                n772 = property on="测量模式(公式)" class="Ring (严格)"() -> ("NumItems"=w1262:u32)  [unwired: 2 in, 2 out]
                n773 = for {
                  N: w1262 -> [_]
                  tunnel: w1261 -> [w1268]
                  i -> [w1266]
                  n774 = local read "多项式系数1"() -> (w1274:dbl[])
                  n775 = Increment(x=w1266) -> (x+1=w1265:i32)
                  n776 = case shown="2" w1265 {
                    tunnel: [u16 4626 ("starting address") w1281 w1286 w1291 w1296 w1301 w1306 w1311] -> w1264
                    frame 0, Default {
                    }
                    frame 1 {
                      n777 = local read "量程选择"() -> (w1280:enum16{"低量程", "高量程", "0-2量程"})
                      n778 = case shown="\"低量程\", 默认" w1280 {
                        tunnel: [u16 4626 ("starting address") u16 4632 ("starting address") u16 4638 ("starting address")] -> w1281
                        frame "低量程", Default {
                        }
                        frame "高量程" {
                        }
                        frame "0-2量程" {
                        }
                      }
                    }
                    frame 2 {
                      n779 = local read "量程选择"() -> (w1285:enum16{"低量程", "高量程", "0-2量程"})
                      n780 = case shown="\"低量程\", 默认" w1285 {
                        tunnel: [u16 4638 ("starting address") u16 4644 ("starting address") u16 4638 ("starting address")] -> w1286
                        frame "低量程", Default {
                        }
                        frame "高量程" {
                        }
                        frame "0-2量程" {
                        }
                      }
                    }
                    frame 3 {
                      n781 = local read "量程选择"() -> (w1290:enum16{"低量程", "高量程", "0-2量程"})
                      n782 = case shown="\"低量程\", 默认" w1290 {
                        tunnel: [u16 4650 ("starting address") u16 4656 ("starting address") u16 4638 ("starting address")] -> w1291
                        frame "低量程", Default {
                        }
                        frame "高量程" {
                        }
                        frame "0-2量程" {
                        }
                      }
                    }
                    frame 4 {
                      n783 = local read "量程选择"() -> (w1295:enum16{"低量程", "高量程", "0-2量程"})
                      n784 = case shown="\"低量程\", 默认" w1295 {
                        tunnel: [u16 4662 ("starting address") u16 4668 ("starting address") u16 4638 ("starting address")] -> w1296
                        frame "低量程", Default {
                        }
                        frame "高量程" {
                        }
                        frame "0-2量程" {
                        }
                      }
                    }
                    frame 5 {
                      n785 = local read "量程选择"() -> (w1300:enum16{"低量程", "高量程", "0-2量程"})
                      n786 = case shown="\"低量程\", 默认" w1300 {
                        tunnel: [u16 4674 ("starting address") u16 4680 ("starting address") u16 4638 ("starting address")] -> w1301
                        frame "低量程", Default {
                        }
                        frame "高量程" {
                        }
                        frame "0-2量程" {
                        }
                      }
                    }
                    frame 6 {
                      n787 = local read "量程选择"() -> (w1305:enum16{"低量程", "高量程", "0-2量程"})
                      n788 = case shown="\"低量程\", 默认" w1305 {
                        tunnel: [u16 4686 ("starting address") u16 4692 ("starting address") u16 4638 ("starting address")] -> w1306
                        frame "低量程", Default {
                        }
                        frame "高量程" {
                        }
                        frame "0-2量程" {
                        }
                      }
                    }
                    frame 7 {
                      n789 = local read "量程选择"() -> (w1310:enum16{"低量程", "高量程", "0-2量程"})
                      n790 = case shown="\"低量程\", 默认" w1310 {
                        tunnel: [u16 4698 ("starting address") u16 4704 ("starting address") u16 4638 ("starting address")] -> w1311
                        frame "低量程", Default {
                        }
                        frame "高量程" {
                        }
                        frame "0-2量程" {
                        }
                      }
                    }
                  }
                  n791 = Index Array(array=w1274) -> (element #1=w1277:dbl, element #2=w1276:dbl, element #3=w1278:dbl)  [unwired: 3 in]
                  n792 = Build Array(w1276, w1277, w1278) -> (w1275:dbl[])
                  n793 = call "浮点转CDAB整形cod.vi"("浮点数"=w1275) -> ("CDAB整形输出"=w1273:u16[])  [unwired: 10 in]
                  n794 = Insert Into Array(array=u16[] [], index=0 ("索引"), new element=w1273) -> (w1263:u16[])
                  n795 = Bundle By Name(cluster=cluster{"starting address":u16, "values":u16[]} {"starting address"=4272, "values"=[]}, "starting address"=w1264, "values"=w1263) -> (w1269:cluster{"starting address":u16, "values":u16[]})
                  n796 = Enqueue Element(queue=w1268, element=w1269, timeout in ms (-1)=1000 ("超时毫秒(-1)")) -> ()  [unwired: 1 in, 3 out]
                }
              }
            }
          }
          frame #1 {
            n797 = local write "枚举"(enum16{"读取数据", "写入数据", "读取写入DATABASE", "读取参数"}."写入数据" ("枚举")) -> ()
          }
        }
      }
      event "滴定曲线": Value Change {
        n798 = event-data() -> ()  [unwired: 1 in, 6 out]
        n799 = property on="窗格" class="Pane"("Origin"=T13 {"Horizontal"=0, "Vertical"=3200} ("原点")) -> ()  [unwired: 2 in, 2 out]
      }
      event "历史波形": Value Change {
        n800 = event-data() -> ()  [unwired: 1 in, 6 out]
        n801 = call-poly <vilib>:"Read Waveforms from File.vi"() -> ("error out"=w1317:errorcluster, "first waveform in record"=w1318:waveform(dbl))  [unwired: 6 in, 2 out]
        n802 = case shown="无错误" w1317 {
          tunnel: w1318 -> [w1321 _]
          frame No Error {
            n803 = Unbundle By Name(w1321) -> ("t0"=→"波形时间":timestamp, "Y"=w1320:dbl[])  [unwired: 2 out]
            n804 = local write "滴定数-ORP值"(w1320) -> ()
            n805 = local write "ORP滴定曲线"(w1320) -> ()
          }
          frame Error {
            n806 = One Button Dialog(message="打开失败" ("消息")) -> ()  [unwired: 1 in, 1 out]
          }
        }
      }
      event Timeout {
        n807 = event-data() -> ()  [unwired: 1 in, 3 out]
      }
    }
  }
  n808 = while {
    tunnel: w32 -> [w1411]
    tunnel: w31 -> [w1410]
    tunnel: w22 -> [w1406]
    tunnel: w21 -> [w1405]
    tunnel: w1 -> [w1323]
    stop <- FALSE stop-if-true
    n809 = local read "自动切换量程:"() -> (w1324:enum16{"关闭", "自动切换测一次", "自动切换测两次"})
    n810 = Wait (ms)(milliseconds to wait=u32 500 ("等待时间（毫秒）")) -> ()  [unwired: 1 out]
    n811 = Bundle By Name(cluster=T5 {"starting address"=4224, "number of holding registers"=16}, "starting address"=u16 4224, "number of holding registers"=u16 50) -> (w1464:T5)
    n812 = case shown="\"自动切换测两次\"" w1324 {
      tunnel: w1323 -> [_ _ w1465]
      frame "关闭", Default {
      }
      frame "自动切换测一次" {
      }
      frame "自动切换测两次" {
        n813 = local read "切换量程连续测两次"() -> (w1467:bool)
        n814 = local read "待机"() -> (w1468:bool)
        n815 = Compound Arithmetic op=AND ("复合运算")(w1468, w1467) -> (w1466:bool)
        n816 = case shown="真" w1466 {
          tunnel: w1465 -> [_ w1470]
          frame False {
          }
          frame True {
            n817 = local read "测量模式数字"() -> (w1474:i32)
            n818 = case shown="0" w1474 {
              tunnel: [u16 4608 ("address") u16 4608 ("address") u16 4608 ("address") u16 4608 ("address") u16 4608 ("address") u16 4608 ("address") u16 4608 ("address") u16 4608 ("address") u16 4608 ("address") u16 4608 ("address")] -> w1475
              tunnel: [u16 1 ("address") u16 2 ("address") u16 3 ("address") u16 4 ("address") u16 5 ("address") u16 7 ("address") u16 6 ("address") u16 8 ("address") u16 9 ("address") u16 0 ("address")] -> w1478
              frame 0 {
              }
              frame 1 {
              }
              frame 2 {
              }
              frame 3 {
              }
              frame 4 {
              }
              frame 5 {
              }
              frame 6 {
              }
              frame 7 {
              }
              frame 8 {
              }
              frame 9, Default {
              }
            }
            n819 = local write "切换量程连续测两次"(FALSE ("切换量程连续测两次")) -> ()
            n820 = local write "枚举"(enum16{"读取数据", "写入数据", "读取写入DATABASE", "读取参数"}."写入数据" ("枚举")) -> ()
            n821 = Insert Into Array(array=u16[] [] ("values"), index=0 ("索引"), new element=w1478) -> (w1479:u16[])
            n822 = Bundle By Name(cluster=cluster{"starting address":u16, "values":u16[]} {"starting address"=0, "values"=[]}, "starting address"=w1475, "values"=w1479) -> (w1472:cluster{"starting address":u16, "values":u16[]})
            n823 = Enqueue Element(queue=w1470, element=w1472) -> ()  [unwired: 2 in, 3 out]
          }
        }
      }
    }
    n824 = Enqueue Element(queue=w1411, element=w1464, error in (no error)=w1410) -> ()  [unwired: 1 in, 3 out]
    n825 = local read "Registers"() -> (w1361:u16[])
    n826 = To Word Integer(number=w1361) -> (16bit integer=w1360:i16[])
    n827 = Index Array(array=w1360, index #1=0 ("索引"), index #4=3 ("索引"), index #14=13 ("索引"), index #15=14 ("索引"), index #21=20 ("索引"), index #32=31 ("索引")) -> (element #1=w1389:i16, element #2=w1388:i16, element #3=w1387:i16, element #4=w1342:i16, element #5=→"模式（受控）":i16, element #6=→"进样管":i16, element #7=→"高锰酸钾":i16, element #8=→"草酸钠":i16, element #9=→"硫酸":i16, element #10=w1359:i16, element #11=w1438:i16, element #12=w1339:i16, element #13=w1353:i16, element #14=w1455:i16, element #15=w1413:i16, element #16=w1329:i16, element #21=w1325:i16, element #33=→"分":i16, element #34=→"秒":i16)  [unwired: 28 in, 15 out]
    "多列列表框" <- w1329
    n828 = Number To Decimal String(number=w1325) -> (decimal integer string=→"基本量程(显示)":string)  [unwired: 1 in]
    n829 = global write "COD浓度全局变量.vi" "基本量程"(w1325) -> ()
    n830 = Build Array(w1389, w1388, w1387) -> (w1390:i16[])
    n831 = To Single Precision Float(number=w1359) -> (single precision float=→"ORP显示":sgl)
    n832 = Divide(x=w1413, y=u16 1000) -> (x/y=→"标度滴定值":dbl)
    n833 = Divide(x=w1438, y=u16 10) -> (x/y=→"温度":dbl)
    n834 = Equal?(x=w1339, y=u16 2) -> (x = y?=→"断电排液标记":bool)
    n835 = global write "COD测量模式全局.vi" "CODMn工作状态"(w1342) -> ()
    n836 = Equal?(x=w1353, y=u16 2) -> (x = y?=w1351:bool)
    "温控器故障" <- w1351
    n837 = Equal?(x=w1353, y=u16 3) -> (x = y?=w1350:bool)
    "加热故障" <- w1350
    n838 = Equal?(x=w1353, y=u16 4) -> (x = y?=w1349:bool)
    "高锰酸钾报警" <- w1349
    n839 = Equal?(x=w1353, y=u16 5) -> (x = y?=w1348:bool)
    "草酸钠报警" <- w1348
    n840 = Equal?(x=w1353, y=u16 6) -> (x = y?=w1347:bool)
    "测量错误" <- w1347
    n841 = Equal?(x=w1353, y=u16 8) -> (x = y?=w1346:bool)
    "校零错误" <- w1346
    n842 = Equal?(x=w1353, y=u16 7) -> (x = y?=w1345:bool)
    "校标错误" <- w1345
    n843 = Equal?(x=w1353, y=u16 9) -> (x = y?=w1344:bool)
    "进水样超量程" <- w1344
    n844 = Divide(x=w1455, y=u16 1000) -> (x/y=→"零点滴定值":dbl)
    n845 = Equal?(x=w1353, y=u16 10) -> (x = y?=w1343:bool)
    "排液故障" <- w1343
    n846 = Equal?(x=w1339, y=u16 1) -> (x = y?=→"排液标记":bool)
    n847 = global write "运行时序全局变量.vi" "多列列表框"(w1329) -> ()
    n848 = Equal?(x=w1353, y=u16 1) -> (x = y?=w1352:bool)
    "ORP故障" <- w1352
    n849 = Equal?(x=w1342, y=u16 0) -> (x = y?=→"待机":bool)
    n850 = Equal?(x=w1342, y=u16 8) -> (x = y?=→"校零标记":bool)
    n851 = Equal?(x=w1342, y=u16 9) -> (x = y?=→"校标标记":bool)
    n852 = Equal?(x=w1342, y=u16 1) -> (x = y?=→"水样测量":bool)
    n853 = Equal?(x=w1342, y=u16 7) -> (x = y?=→"质控样测量":bool)
    n854 = Equal?(x=w1342, y=u16 10) -> (x = y?=→"加标回收测量":bool)
    n855 = Equal?(x=w1342, y=u16 2) -> (x = y?=→"标样核查标记":bool)
    n856 = Equal?(x=w1342, y=u16 6) -> (x = y?=→"平行样测量":bool)
    n857 = Equal?(x=w1342, y=u16 3) -> (x = y?=→"零点核查标记":bool)
    n858 = Equal?(x=w1342, y=u16 4) -> (x = y?=→"跨度核查标记":bool)
    n859 = Equal?(x=w1342, y=u16 5) -> (x = y?=→"空白测试标记":bool)
    n860 = feedback #2(w1329) -> (w1396:i16)
    n861 = feedback-in #2(w1329) -> ()
    n862 = Compound Arithmetic op=OR ("复合运算")(w1352, w1351, w1350, w1349, w1348, w1347, w1345, w1346, w1344, w1343) -> (→"故障标记":bool)
    n863 = Not Equal?(x=w1329, y=w1396) -> (x != y?=w1395:bool)
    n864 = Bundle By Name(cluster=T3 {"ORP故障"=FALSE, "温控器故障"=FALSE, "加热故障"=FALSE, "高锰酸钾报警"=FALSE, "草酸钠报警"=FALSE, "测量错误"=FALSE, "校零错误"=FALSE, "校标错误"=FALSE, " 进水样超量程"=FALSE, "排液阀故障"=FALSE} ("报警簇"), "ORP故障"=w1352, "温控器故障"=w1351, "加热故障"=w1350, "高锰酸钾报警"=w1349, "草酸钠报警"=w1348, "测量错误"=w1347, "校零错误"=w1346, "校标错误"=w1345, "进水样超量程"=w1344, "排液阀故障"=w1343) -> (w1397:T3)
    "报警簇" <- w1397
    n865 = call "HexToDate.vi"("数组"=w1390) -> ("DATE"=w1385:timestamp[])  [unwired: 10 in]
    n866 = Index Array(array=w1385) -> (element=→"仪器时间":timestamp)  [unwired: 1 in]
    n867 = First Call?() -> (First Call?: T/F=w1335:bool)
    n868 = Get Date/Time In Seconds() -> (seconds since 1Jan1904=w1384:timestamp)
    "系统时间" <- w1384
    n869 = call "CODMn报警信息.vi"("报警簇"=w1397) -> ("CODMN报警信息"=w1398:string)  [unwired: 10 in]
    n870 = case shown="假" w1335 {
      tunnel: w1395 -> [w1504 _]
      tunnel: w1329 -> [w1503 _]
      frame False {
        n871 = case shown="真" w1504 {
          tunnel: w1503 -> [_ w1516]
          frame False {
          }
          frame True {
            n872 = property on="多列列表框" class="MCListbox (严格)"() -> ("ItemNames"=w1510:string[][])  [unwired: 2 in, 2 out]
            n873 = Index Array(array=w1510, index (row)=w1516) -> (element=w1507:string[])  [unwired: 1 in]
            n874 = Index Array(array=w1507, index=0 ("索引")) -> (element=w1505:string)
            n875 = Array To Spreadsheet String(delimiter (Tab)="-" ("分隔符(Tab)"), array=w1507, 3:"" ("格式字符串")) -> ()  [unwired: 1 out]
            n876 = Get Date/Time In Seconds() -> (seconds since 1Jan1904=w1514:timestamp)
            n877 = Bundle(cluster=T14 {"时间标识"=timestamp(0 s since 1904-01-01), "参数"="", "日志信息"="", "流程参数"=""} ("data in"), "时间标识"=w1514, "参数"="CODMn" ("table输入"), "日志信息"=w1505, "流程参数"="" ("table输入")) -> (w1511:T14)
            n878 = call "流程日志字段定义.vi"("table输入"="操作日志", "data in"=w1511) -> ("table输出"=w1519:string, "columns"=w1520:string[], "data out"=w1521:T16)  [unwired: 7 in]
            n879 = call "插入数据.vi"("data"=w1521, "columns"=w1520, "database"="database3.mdb", "table"=w1519) -> ()  [unwired: 7 in, 1 out]
          }
        }
      }
      frame True {
      }
    }
    n880 = local read "断电排液标记"() -> (w1337:bool)
    n881 = Greater?(x=w1329, y=u16 0) -> (0:w1328:bool)
    n882 = Less Or Equal?(x=w1329, y=u16 4) -> (x <= y?=w1366:bool)
    n883 = Equal?(x=w1329, y=u16 5) -> (x = y?=w1409:bool)
    n884 = feedback #3(w1398) -> (w1399:string)
    n885 = feedback-in #3(w1398) -> ()
    n886 = Greater?(x=w1329, y=u16 0) -> (0:w1363:bool)
    n887 = Not Equal?(x=w1398, y="") -> (x != y?=w1403:bool)
    n888 = call <vilib>:"Boolean Crossing PtByPt.vi"("direction"=enum16{"either", "false-true", "true-false"}."false-true", "input"=w1337) -> ("crossing"=w1336:bool)  [unwired: 1 in]
    n889 = And(x=w1328, y=w1366) -> (x .and. y?=w1331:bool)
    n890 = call <vilib>:"Boolean Crossing PtByPt.vi"("direction"=enum16{"either", "false-true", "true-false"}."false-true", "input"=w1409) -> ("crossing"=w1407:bool)  [unwired: 1 in]
    n891 = call <vilib>:"Boolean Crossing PtByPt.vi"("direction"=enum16{"either", "false-true", "true-false"}."false-true", "input"=w1363) -> ("crossing"=w1362:bool)  [unwired: 1 in]
    n892 = Build Array(w1384) -> (w1383:timestamp[])
    n893 = Not Equal?(x=w1398, y=w1399) -> (x != y?=w1400:bool)
    n894 = case shown="真" w1336 {
      frame False {
      }
      frame True {
        n895 = Get Date/Time In Seconds() -> (seconds since 1Jan1904=w1527:timestamp)
        n896 = Bundle(cluster=T14 {"时间标识"=timestamp(0 s since 1904-01-01), "参数"="", "日志信息"="", "流程参数"=""} ("data in"), "时间标识"=w1527, "参数"="CODMn" ("table输入"), "日志信息"="断电排液", "流程参数"="" ("table输入")) -> (w1525:T14)
        n897 = call "流程日志字段定义.vi"("table输入"="操作日志", "data in"=w1525) -> ("table输出"=w1530:string, "columns"=w1531:string[], "data out"=w1532:T16)  [unwired: 7 in]
        n898 = call "插入数据.vi"("data"=w1532, "columns"=w1531, "database"="database3.mdb", "table"=w1530) -> ()  [unwired: 7 in, 1 out]
      }
    }
    n899 = case shown="真" w1407 {
      tunnel: w1406 -> [_ w1577]
      tunnel: w1405 -> [_ w1572]
      frame False {
      }
      frame True {
        n900 = Bundle By Name(cluster=T5 {"starting address"=0, "number of holding registers"=0}, "starting address"=u16 4101, "number of holding registers"=u16 10) -> (w1576:T5)
        n901 = Enqueue Element(queue=w1577, element=w1576, error in (no error)=w1572) -> ()  [unwired: 1 in, 3 out]
        n902 = local write "枚举"(enum16{"读取数据", "写入数据", "读取写入DATABASE", "读取参数"}."读取写入DATABASE" ("枚举")) -> ()
      }
    }
    n903 = case shown="真" w1331 {
      frame False {
      }
      frame True {
        n904 = local read "测量模式数字"() -> (w1542:i32)
        n905 = local read "标样核查标记"() -> (w1545:bool)
        n906 = local read "零点核查标记"() -> (w1544:bool)
        n907 = local read "跨度核查标记"() -> (w1540:bool)
        n908 = local read "空白测试标记"() -> (w1539:bool)
        n909 = local read "加标回收测量"() -> (w1538:bool)
        n910 = local read "平行样测量"() -> (w1537:bool)
        n911 = local read "启动时间"() -> (w1534:timestamp)
        n912 = local read "水样测量"() -> (w1546:bool)
        n913 = local read "校零标记"() -> (w1536:bool)
        n914 = local read "校标标记"() -> (w1535:bool)
        n915 = case shown="0, 默认" w1542 {
          tunnel: ["水样测试" ("测量模式") "标样核查" ("测量模式") "零点核查" ("测量模式") "跨度核查" ("测量模式") "空白测试" ("测量模式") "加标回收" ("测量模式") "平行样" ("测量模式") "校零" ("测量模式") "校标" ("测量模式")] -> w1541
          tunnel: w1534 -> [w1547 _ _ _ _ w1553 _ _ _]
          frame 0, Default {
            n916 = global write "COD测量模式全局.vi" "水样启动时间"(w1547) -> ()
          }
          frame 1 {
          }
          frame 2 {
          }
          frame 3 {
          }
          frame 4 {
          }
          frame 5 {
            n917 = global write "COD测量模式全局.vi" "加标回收启动时间"(w1553) -> ()
          }
          frame 6 {
          }
          frame 7 {
          }
          frame 8 {
          }
        }
        n918 = Build Array(w1546, w1545, w1544, w1540, w1539, w1538, w1537, w1536, w1535) -> (w1543:bool[])
        n919 = for {
          tunnel: w1543 -> [w1559] mode=indexing
          i -> [w1558]
          n920 = case shown="真" w1559 {
            tunnel: w1558 -> [_ w1560]
            frame False {
            }
            frame True {
              "测量模式数字" <- w1560
            }
          }
        }
        n921 = global write "COD测量模式全局.vi" "测量模式"(w1541) -> ()
      }
    }
    n922 = case shown="真" w1362 {
      frame False {
      }
      frame True {
        n923 = Get Date/Time In Seconds() -> (seconds since 1Jan1904=→"启动时间":timestamp)
      }
    }
    n924 = call "DateToHex.vi"("DATE"=w1383) -> ("数组"=w1382:u16[])  [unwired: 10 in]
    n925 = call "DateToHex.vi"("DATE"=w1385) -> ("数组"=w1377:u16[])  [unwired: 10 in]
    n926 = And(x=w1400, y=w1403) -> (x .and. y?=w1401:bool)
    n927 = case shown="真" w1401 {
      tunnel: w1398 -> [_ w1561]
      frame False {
      }
      frame True {
        n928 = Get Date/Time In Seconds() -> (seconds since 1Jan1904=w1563:timestamp)
        n929 = Bundle By Name(cluster=T15 {"时间标识"=timestamp(0 s since 1904-01-01), "设备"="", "日志信息"=""} ("data in"), "时间标识"=w1563, "设备"="CODMn", "日志信息"=w1561) -> (w1564:T15)
        n930 = call "报警信息字段定义.vi"("table输入"="报警信息", "data in"=w1564) -> ("table输出"=w1568:string, "columns"=w1569:string[], "data out"=w1570:T15)  [unwired: 7 in]
        n931 = call "插入数据.vi"("data"=w1570, "columns"=w1569, "database"="database3.mdb", "table"=w1568) -> ()  [unwired: 7 in, 1 out]
      }
    }
    n932 = Index Array(array=w1377, index=2 ("索引")) -> (element=w1379:u16)
    n933 = Index Array(array=w1382, index=2 ("索引")) -> (element=w1380:u16)
    n934 = Split Number(x=w1379) -> (hi(x)=w1373:u8)  [unwired: 1 out]
    n935 = Split Number(x=w1380) -> (hi(x)=w1376:u8)  [unwired: 1 out]
    n936 = To Byte Integer(number=w1373) -> (8bit integer=w1372:i8)
    n937 = To Byte Integer(number=w1376) -> (8bit integer=w1375:i8)
    n938 = Subtract(x=w1372, y=w1375) -> (x-y=w1374:i8)
    n939 = local read "通讯状态"() -> (w1333:bool)
    n940 = Absolute Value(x=w1374) -> (abs(x)=w1371:i8)
    n941 = Greater Or Equal?(x=w1371, y=i8 10) -> (x >= y?=w1334:bool)
    n942 = And(x=w1334, y=w1333) -> (x .and. y?=w1332:bool)
    n943 = case shown="真" w1332 {
      frame False {
      }
      frame True {
        n944 = flat-sequence {
          frame #0 {
            n945 = property on="时间校准" class="Bool (严格)"("Val(Sgnl)"=TRUE ("值(信号)")) -> ()  [unwired: 2 in, 2 out]
          }
          frame #1 {
            n946 = Wait (ms)(milliseconds to wait=u32 500 ("等待时间（毫秒）")) -> ()  [unwired: 1 out]
          }
          frame #2 {
            n947 = property on="时间校准" class="Bool (严格)"("Val(Sgnl)"=FALSE ("值(信号)")) -> ()  [unwired: 2 in, 2 out]
          }
        }
      }
    }
  }
  n948 = while {
    tunnel: w3 -> [w1594]
    tunnel: w2 -> [w1593]
    tunnel: w1 -> [w1592]
    tunnel: w32 -> [w1591]
    tunnel: w31 -> [w1590]
    tunnel: [w1580] -> w30
    tunnel: [w1589] -> w29
    tunnel: w16 -> [w1587]
    tunnel: w15 -> [w1586]
    tunnel: w22 -> [w1585]
    tunnel: w21 -> [w1584]
    tunnel: w20 -> [w1583]
    tunnel: w1 -> [w1578]
    stop <- FALSE stop-if-true
    n949 = case shown="\"读取写入DATABASE\"" "枚举" {
      tunnel: w1594 -> [w1659 w1670 w1753 w1901]
      tunnel: w1593 -> [w1658 w1666 w1752 w1900]
      tunnel: w1592 -> [_ w1669 _ _]
      tunnel: [w1627 w1668 w1755 w1895] -> w1589
      tunnel: [w1626 w1667 w1754 w1893] -> w1580
      tunnel: w1591 -> [w1656 _ _ _]
      tunnel: w1590 -> [w1652 _ _ _]
      tunnel: w1587 -> [_ _ _ w1899]
      tunnel: w1586 -> [_ _ _ w1898]
      tunnel: w1585 -> [_ _ w1751 _]
      tunnel: w1584 -> [_ _ w1750 _]
      tunnel: w1583 -> [_ w1665 _ _]
      tunnel: w1578 -> [_ _ w1720 _]
      frame "读取数据", Default {
        # "A，B，K"
        n950 = Dequeue Element(queue=w1656, timeout in ms (-1)=1000 ("超时毫秒(-1)"), error in (no error)=w1652) -> (element=w1655:T5)  [unwired: 3 out]
        n951 = Unbundle By Name(w1655) -> ("starting address"=w1654:u16, "number of holding registers"=w1653:u16)
        n952 = call <vilib>:"Read Holding Registers.vi"("error in (no error)"=w1658, "quantity"=w1653, "starting address"=w1654, "MB session in"=w1659) -> ("error out"=w1624:errorcluster, "Registers"=w1657:u16[], "MB session out"=w1625:refnum<class "MB_Master_Serial.lvclass">)  [unwired: 5 in]
        n953 = case shown="无错误" w1624 {
          tunnel: w1657 -> [w1660 _]
          frame No Error {
            "Registers" <- w1660
          }
          frame Error {
          }
        }
        n954 = call <vilib>:"Read Holding Registers.vi"("error in (no error)"=w1624, "quantity"=u16 10, "starting address"=u16 4101, "MB session in"=w1625) -> ("error out"=w1620:errorcluster, "Registers"=w1618:u16[], "MB session out"=w1621:refnum<class "MB_Master_Serial.lvclass">)  [unwired: 5 in]
        n955 = To Word Integer(number=w1618) -> (16bit integer=w1617:i16[])
        n956 = Split 1D Array(array=w1617, index=3 ("索引")) -> (first subarray=w1597:i16[], second subarray=w1616:i16[])
        n957 = call <vilib>:"Read Coils.vi"("error in (no error)"=w1620, "quantity"=u16 8, "starting address"=u16 140, "MB session in"=w1621) -> ("error out"=w1639:errorcluster, "Coils"=w1648:bool[], "MB session out"=w1640:refnum<class "MB_Master_Serial.lvclass">)  [unwired: 5 in]
        n958 = Index Array(array=w1597) -> (element #1=w1601:i16, element #2=w1600:i16, element #3=w1599:i16)  [unwired: 3 in]
        n959 = Index Array(array=w1616) -> (element #1=w1611:i16, element #2=w1615:i16, element #3=w1614:i16, element #4=w1613:i16)  [unwired: 4 in]
        n960 = To Single Precision Float(number=w1614) -> (single precision float=w1604:sgl)
        n961 = To Single Precision Float(number=w1611) -> (single precision float=w1610:sgl)
        n962 = To Single Precision Float(number=w1615) -> (single precision float=w1608:sgl)
        n963 = To Single Precision Float(number=w1613) -> (single precision float=w1603:sgl)
        n964 = Index Array(array=w1648) -> (element #1=→"进水样":bool, element #2=→"进蒸馏水":bool, element #3=→"进标液":bool, element #4=→"进质控样":bool, element #5=→"进加标回收样":bool, element #6=→"进高锰酸钾":bool, element #7=→"进草酸钠":bool, element #8=→"进硫酸":bool)  [unwired: 9 in, 1 out]
        n965 = Build Array(w1601, w1600, w1599) -> (w1598:i16[])
        n966 = Divide(x=w1610, y=sgl 100.0) -> (x/y=w1609:sgl)
        n967 = Number To Decimal String(number=w1608) -> (decimal integer string=→"ORP-A":string)  [unwired: 1 in]
        n968 = Number To Decimal String(number=w1604) -> (decimal integer string=→"ORP-B":string)  [unwired: 1 in]
        n969 = Number To Decimal String(number=w1603) -> (decimal integer string=→"ORP-K":string)  [unwired: 1 in]
        n970 = local write "COD浓度（mg/L)"(w1609) -> ()
        n971 = call "HexToDate.vi"("数组"=w1598) -> ("DATE"=w1602:timestamp[])  [unwired: 10 in]
        n972 = call <vilib>:"Read Coils.vi"("error in (no error)"=w1639, "quantity"=u16 1, "starting address"=u16 137, "MB session in"=w1640) -> ("error out"=w1635:errorcluster, "Coils"=w1629:bool[], "MB session out"=w1636:refnum<class "MB_Master_Serial.lvclass">)  [unwired: 5 in]
        n973 = Index Array(array=w1602) -> (element=w1595:timestamp)  [unwired: 1 in]
        n974 = Format Date/Time String(seconds (now)=w1595) -> (date/time string=w1596:string)  [unwired: 2 in]
        n975 = local write "启动时间"(w1595) -> ()
        n976 = local write "数据时间"(w1596) -> ()
        n977 = Index Array(array=w1629) -> (element=→"搅拌":bool)  [unwired: 1 in]
        n978 = call <vilib>:"Read Coils.vi"("error in (no error)"=w1635, "quantity"=u16 1, "starting address"=u16 400, "MB session in"=w1636) -> ("error out"=w1626:errorcluster, "Coils"=w1632:bool[], "MB session out"=w1627:refnum<class "MB_Master_Serial.lvclass">)  [unwired: 5 in]
        n979 = Index Array(array=w1632) -> (element=→"加热":bool)  [unwired: 1 in]
      }
      frame "写入数据" {
        n980 = flat-sequence {
          tunnel: w1670 -> [w1681]
          tunnel: w1669 -> [w1680]
          tunnel: w1666 -> [w1674]
          tunnel: w1665 -> [w1673]
          tunnel: [w1676] -> w1664
          tunnel: [w1675] -> w1663
          tunnel: [w1672] -> w1662
          tunnel: [w1671] -> w1661
          tunnel: [w1682] -> w1667
          tunnel: [w1688] -> w1668
          tunnel: w1664 -> [w1688]
          tunnel: w1663 -> [w1682]
          tunnel: w1662 -> [w1687]
          tunnel: w1661 -> [w1686]
          frame #0 {
            n981 = Dequeue Element(queue=w1680, error in (no error)=w1673) -> (queue out=w1672:refnum<queue>, element=w1679:cluster{"starting address":u16, "values":u16[]}, error out=w1671:errorcluster)  [unwired: 1 in, 1 out]
            n982 = Unbundle By Name(w1679) -> ("starting address"=w1678:u16, "values"=w1677:u16[])
            n983 = call <vilib>:"Write Multiple Registers.vi"("error in (no error)"=w1674, "values"=w1677, "starting address"=w1678, "MB session in"=w1681) -> ("error out"=w1675:errorcluster, "MB session out"=w1676:refnum<class "MB_Master_Serial.lvclass">)  [unwired: 6 in]
          }
          frame #1 {
            n984 = Get Queue Status(queue=w1687, error in (no error)=w1686) -> (# elements in queue=w1685:i32)  [unwired: 1 in, 7 out]
            n985 = Equal To 0?(x=w1685) -> (x = 0?=w1684:bool)
            n986 = case shown="假" w1684 {
              tunnel: [enum16{"读取数据", "写入数据", "读取写入DATABASE", "读取参数"}."写入数据" ("枚举") enum16{"读取数据", "写入数据", "读取写入DATABASE", "读取参数"}."读取数据" ("枚举")] -> w1683
              tunnel: w1682 -> [_ w1690]
              frame False {
              }
              frame True {
                n987 = case shown="无错误" w1690 {
                  tunnel: ["保存成功" ("消息") "保存失败" ("消息")] -> _
                  frame No Error {
                  }
                  frame Error {
                  }
                }
              }
            }
            n988 = local write "枚举"(w1683) -> ()
          }
        }
      }
      frame "读取写入DATABASE" {
        n989 = Dequeue Element(queue=w1751, timeout in ms (-1)=1000 ("超时毫秒(-1)"), error in (no error)=w1750) -> (element=w1758:T5)  [unwired: 3 out]
        n990 = Unbundle By Name(w1758) -> ("starting address"=w1757:u16, "number of holding registers"=w1756:u16)
        n991 = call <vilib>:"Read Holding Registers.vi"("error in (no error)"=w1752, "quantity"=w1756, "starting address"=w1757, "MB session in"=w1753) -> ("error out"=w1754:errorcluster, "Registers"=w1709:u16[], "MB session out"=w1755:refnum<class "MB_Master_Serial.lvclass">)  [unwired: 5 in]
        n992 = To Word Integer(number=w1709) -> (16bit integer=w1708:i16[])
        n993 = Split 1D Array(array=w1708, index=3 ("索引")) -> (first subarray=w1748:i16[], second subarray=w1738:i16[])
        n994 = global read "CODMN外部API.vi" "CODMn外围API"() -> (w1697:T17)
        n995 = Index Array(array=w1748) -> (element #1=w1746:i16, element #2=w1745:i16, element #3=w1744:i16)  [unwired: 3 in]
        n996 = Index Array(array=w1738) -> (element #1=w1713:i16, element #2=w1742:i16, element #3=w1741:i16, element #4=w1740:i16, element #5=w1739:i16)  [unwired: 5 in]
        n997 = Index Array(array=w1738, index=6 ("索引")) -> (element=w1736:i16)
        n998 = To Single Precision Float(number=w1713) -> (single precision float=w1715:sgl)
        n999 = Unbundle By Name(w1697) -> ("运行模式"=w1696:enum16{"维护模式", "常规模式", "应急模式", "质控模式"})
        n1000 = Divide(x=w1715, y=sgl 100.0) -> (x/y=w1714:sgl)
        n1001 = Less Or Equal?(x=w1714, y=sgl 0.01) -> (x <= y?=w1717:bool)
        n1002 = case shown="\"维护模式\", 默认" w1696 {
          tunnel: ["M" ("单位") "N" ("单位") "N" ("单位") "N" ("单位")] -> w1722
          frame "维护模式", Default {
          }
          frame "常规模式" {
          }
          frame "应急模式" {
          }
          frame "质控模式" {
          }
        }
        n1003 = case shown="真" w1717 {
          tunnel: [w1884 w1885] -> w1716
          tunnel: w1714 -> [w1884 _]
          frame False {
          }
          frame True {
            n1004 = Random Number (0-1)() -> (number: 0 to 1=w1888:dbl)
            n1005 = Increment(x=w1888) -> (x+1=w1886:dbl)
            n1006 = Divide(x=w1886, y=sgl 100.0) -> (x/y=w1885:dbl)
          }
        }
        n1007 = Build Array(w1746, w1745, w1744) -> (w1743:i16[])
        n1008 = To Single Precision Float(number=w1742) -> (single precision float=w1726:sgl)
        n1009 = To Single Precision Float(number=w1736) -> (single precision float=w1719:sgl)
        n1010 = To Single Precision Float(number=w1741) -> (single precision float=w1727:sgl)
        n1011 = To Single Precision Float(number=w1740) -> (single precision float=w1728:sgl)
        n1012 = To Single Precision Float(number=w1739) -> (single precision float=w1733:sgl)
        n1013 = call "HexToDate.vi"("数组"=w1743) -> ("DATE"=w1747:timestamp[])  [unwired: 10 in]
        n1014 = Index Array(array=w1747) -> (element=w1704:timestamp)  [unwired: 1 in]
        n1015 = Greater Than 0?(x="量程切换次数") -> (x > 0?=w1699:bool)
        n1016 = disable-structure shown="启用" {
          disable-tunnel: w1716 -> [w1849 w1873]
          disable-tunnel: [w1848 w1873] -> w1702
          frame Disabled {
            # "高量程0-5之间会乘1.2的系数\n低量程0-2之间会乘1.1的系数"
            n1017 = property on="基本量程" class="Enum (严格)"() -> ("Value"=w1850:enum16{"L", "H"})  [unwired: 2 in, 2 out]
            n1018 = case shown="\"L\", 默认" w1850 {
              tunnel: w1849 -> [w1853 w1863]
              tunnel: [w1851 w1862] -> w1848
              frame "L", Default {
                n1019 = Less Or Equal?(x=w1853, y=2.0) -> (x <= y?=w1856:bool)
                n1020 = Greater?(x=w1853, y=0.0) -> (0:w1855:bool)
                n1021 = And(x=w1856, y=w1855) -> (x .and. y?=w1852:bool)
                n1022 = case shown="真" w1852 {
                  tunnel: w1853 -> [w1858 w1861]
                  tunnel: [w1858 w1859] -> w1851
                  frame False {
                  }
                  frame True {
                    n1023 = Multiply(x=w1861, y=1.1) -> (x*y=w1859:dbl)
                  }
                }
              }
              frame "H" {
                n1024 = Greater?(x=w1863, y=0.0) -> (0:w1866:bool)
                n1025 = Less Or Equal?(x=w1863, y=5.0) -> (x <= y?=w1867:bool)
                n1026 = And(x=w1867, y=w1866) -> (x .and. y?=w1864:bool)
                n1027 = case shown="真" w1864 {
                  tunnel: w1863 -> [w1869 w1872]
                  tunnel: [w1869 w1870] -> w1862
                  frame False {
                  }
                  frame True {
                    n1028 = Multiply(x=w1872, y=1.2) -> (x*y=w1870:dbl)
                  }
                }
              }
            }
          }
          frame Enabled {
          }
        }
        "COD浓度（mg/L)" <- w1702
        n1029 = local write "启动时间"(w1704) -> ()
        n1030 = Format Date/Time String(seconds (now)=w1704) -> (date/time string=→"数据时间":string)  [unwired: 2 in]
        n1031 = global read "COD测量模式全局.vi" "测量模式"() -> (w1694:string)
        n1032 = global read "COD测量模式全局.vi" "测量模式"() -> (w1707:string)
        n1033 = case shown="\"跨度核查\"" w1707 {
          tunnel: [w1874 w1875 w1876] -> w1706
          frame "", Default {
            n1034 = local read "标准液浓度"() -> (w1874:dbl)
          }
          frame "标样核查", "校标" {
            n1035 = local read "标准液浓度"() -> (w1875:dbl)
          }
          frame "跨度核查" {
            n1036 = local read "跨度液浓度"() -> (w1876:dbl)
          }
        }
        n1037 = local read "故障标记"() -> (w1703:bool)
        n1038 = Divide(x=w1733, y=sgl 1000.0) -> (x/y=w1729:sgl)
        n1039 = case shown="假" w1703 {
          tunnel: [w1844 "D" ("数据标识")] -> w1724
          frame False {
            n1040 = global read "CODMN外部API.vi" "手动启动CODMn"() -> (w1843:bool)
            n1041 = case shown="假" w1843 {
              tunnel: ["N" ("数据标识") "hd" ("数据标识")] -> w1844
              frame False {
              }
              frame True {
              }
            }
          }
          frame True {
          }
        }
        n1042 = global read "COD浓度全局变量.vi" "基本量程"() -> (w1695:enum16{"10mg/L", "20mg/L"})
        n1043 = local read "温度"() -> (w1721:dbl)
        n1044 = Format Into String(format string="w%05d" ("格式字符串"), u32 1019 ("因子编码")) -> (resulting string=w1725:string)  [unwired: 2 in, 1 out]
        n1045 = Bundle(cluster=T12 {"时间"=timestamp(0 s since 1904-01-01), "测量模式"="", "数据类型"="", "检测值"=0.0, "单位"="", "数据标识"="", "因子编码"="", "标样参考值"=0.0, "ORP-A"=0.0, "ORP-B"=0.0, "ORP-K"=0.0, "COD滴定值"=0.0, "高锰酸钾滴定数"=0.0, "温度"=0.0, "量程"=0.0} ("data"), "时间"=w1704, "测量模式"=w1694, "数据类型"=w1722, "检测值"=w1702, "单位"="mg/L", "数据标识"=w1724, "因子编码"=w1725, "标样参考值"=w1706, "ORP-A"=w1726, "ORP-B"=w1727, "ORP-K"=w1728, "COD滴定值"=w1729, "高锰酸钾滴定数"=w1719, "温度"=w1721, "量程"=w1695) -> (w1701:T12)
        n1046 = case shown="假" w1699 {
          tunnel: w1720 -> [w1762 _]
          tunnel: w1702 -> [w1760 _]
          tunnel: w1701 -> [w1759 w1839]
          frame False {
            # "量程切换前"
            n1047 = case shown="\"自动切换测两次\"" "自动切换量程:" {
              tunnel: w1762 -> [_ w1776 w1805]
              tunnel: w1760 -> [_ w1772 w1804]
              tunnel: w1759 -> [w1763 w1768 w1803]
              frame "关闭", Default {
                # "关闭自动切换量程"
                n1048 = local write "枚举"(enum16{"读取数据", "写入数据", "读取写入DATABASE", "读取参数"}."读取数据" ("枚举")) -> ()
                n1049 = call "存数据cloumns(子VI).vi"() -> ("数组"=w1765:string[])  [unwired: 11 in]
                n1050 = global write "COD读取DATA全局.vi" "data"(w1763) -> ()
                n1051 = call "数据写入database.vi"("data"=w1763, "columns"=w1765, "table"="CODMn") -> ()  [unwired: 8 in, 1 out]
              }
              frame "自动切换测一次" {
                # "自动切换量程选择是否重测"
                n1052 = global read "COD测量模式全局.vi" "测量模式"() -> (w1775:string)
                n1053 = Not Equal?(x=w1775, y="水样测试") -> (x != y?=w1773:bool)
                n1054 = case shown="假" w1773 {
                  tunnel: [w1777 w1778] -> w1771
                  tunnel: w1772 -> [w1777 _]
                  frame False {
                  }
                  frame True {
                    n1055 = global read "COD读取DATA全局.vi" "测量数据区"() -> (w1779:T2)
                    n1056 = Unbundle By Name(w1779) -> ("水样实测值"=w1778:sgl)
                  }
                }
                n1057 = global read "COD浓度全局变量.vi" "基本量程"() -> (w1767:enum16{"10mg/L", "20mg/L"})
                n1058 = case shown="\"20mg/L\"" w1767 {
                  tunnel: w1776 -> [w1781 w1792]
                  tunnel: w1771 -> [w1780 w1791]
                  frame "10mg/L", Default {
                    n1059 = Greater?(x=w1780, y="低切高阈值:") -> (0:w1782:bool)
                    n1060 = case shown="真" w1782 {
                      tunnel: w1781 -> [_ w1785]
                      frame False {
                        n1061 = local write "枚举"(enum16{"读取数据", "写入数据", "读取写入DATABASE", "读取参数"}."读取数据" ("枚举")) -> ()
                      }
                      frame True {
                        n1062 = local write "枚举"(enum16{"读取数据", "写入数据", "读取写入DATABASE", "读取参数"}."写入数据" ("枚举")) -> ()
                        n1063 = Bundle By Name(cluster=cluster{"starting address":u16, "values":u16[]} {"starting address"=0, "values"=[]}, "starting address"=u16 4276, "values"=u16[] [1]) -> (w1787:cluster{"starting address":u16, "values":u16[]})
                        n1064 = Enqueue Element(queue=w1785, element=w1787) -> ()  [unwired: 2 in, 3 out]
                      }
                    }
                  }
                  frame "20mg/L" {
                    n1065 = Less?(x=w1791, y="高切低阈值:") -> (x < y?=w1793:bool)
                    n1066 = case shown="真" w1793 {
                      tunnel: w1792 -> [_ w1796]
                      frame False {
                        n1067 = local write "枚举"(enum16{"读取数据", "写入数据", "读取写入DATABASE", "读取参数"}."读取数据" ("枚举")) -> ()
                      }
                      frame True {
                        n1068 = local write "枚举"(enum16{"读取数据", "写入数据", "读取写入DATABASE", "读取参数"}."写入数据" ("枚举")) -> ()
                        n1069 = Bundle By Name(cluster=cluster{"starting address":u16, "values":u16[]} {"starting address"=0, "values"=[]}, "starting address"=u16 4276, "values"=u16[] [0]) -> (w1798:cluster{"starting address":u16, "values":u16[]})
                        n1070 = Enqueue Element(queue=w1796, element=w1798) -> ()  [unwired: 2 in, 3 out]
                      }
                    }
                  }
                }
                n1071 = call "存数据cloumns(子VI).vi"() -> ("数组"=w1770:string[])  [unwired: 11 in]
                n1072 = global write "COD读取DATA全局.vi" "data"(w1768) -> ()
                n1073 = call "数据写入database.vi"("data"=w1768, "columns"=w1770, "table"="CODMn") -> ()  [unwired: 8 in, 1 out]
              }
              frame "自动切换测两次" {
                # "自动切换量程选择是否重测"
                n1074 = global read "COD浓度全局变量.vi" "基本量程"() -> (w1802:enum16{"10mg/L", "20mg/L"})
                n1075 = case shown="\"20mg/L\"" w1802 {
                  tunnel: w1805 -> [w1809 w1825]
                  tunnel: w1804 -> [w1807 w1823]
                  tunnel: w1803 -> [w1806 w1822]
                  frame "10mg/L", Default {
                    n1076 = local read "低切高阈值:"() -> (w1808:dbl)
                    n1077 = Greater?(x=w1807, y=w1808) -> (0:w1810:bool)
                    n1078 = case shown="真" w1810 {
                      tunnel: w1809 -> [_ w1816]
                      tunnel: w1806 -> [w1811 _]
                      frame False {
                        n1079 = local write "枚举"(enum16{"读取数据", "写入数据", "读取写入DATABASE", "读取参数"}."读取数据" ("枚举")) -> ()
                        n1080 = call "存数据cloumns(子VI).vi"() -> ("数组"=w1813:string[])  [unwired: 11 in]
                        n1081 = global write "COD读取DATA全局.vi" "data"(w1811) -> ()
                        n1082 = call "数据写入database.vi"("data"=w1811, "columns"=w1813, "table"="CODMn") -> ()  [unwired: 8 in, 1 out]
                      }
                      frame True {
                        n1083 = local write "枚举"(enum16{"读取数据", "写入数据", "读取写入DATABASE", "读取参数"}."写入数据" ("枚举")) -> ()
                        n1084 = Bundle By Name(cluster=cluster{"starting address":u16, "values":u16[]} {"starting address"=0, "values"=[]}, "starting address"=u16 4276, "values"=u16[] [1]) -> (w1818:cluster{"starting address":u16, "values":u16[]})
                        n1085 = Enqueue Element(queue=w1816, element=w1818) -> ()  [unwired: 2 in, 3 out]
                        "切换量程连续测两次" <- TRUE ("切换量程连续测两次")
                      }
                    }
                  }
                  frame "20mg/L" {
                    n1086 = local read "高切低阈值:"() -> (w1824:dbl)
                    n1087 = Less?(x=w1823, y=w1824) -> (x < y?=w1826:bool)
                    n1088 = case shown="假" w1826 {
                      tunnel: w1825 -> [_ w1832]
                      tunnel: w1822 -> [w1827 _]
                      frame False {
                        n1089 = local write "枚举"(enum16{"读取数据", "写入数据", "读取写入DATABASE", "读取参数"}."读取数据" ("枚举")) -> ()
                        n1090 = call "存数据cloumns(子VI).vi"() -> ("数组"=w1829:string[])  [unwired: 11 in]
                        n1091 = global write "COD读取DATA全局.vi" "data"(w1827) -> ()
                        n1092 = call "数据写入database.vi"("data"=w1827, "columns"=w1829, "table"="CODMn") -> ()  [unwired: 8 in, 1 out]
                      }
                      frame True {
                        n1093 = local write "枚举"(enum16{"读取数据", "写入数据", "读取写入DATABASE", "读取参数"}."写入数据" ("枚举")) -> ()
                        n1094 = Bundle By Name(cluster=cluster{"starting address":u16, "values":u16[]} {"starting address"=0, "values"=[]}, "starting address"=u16 4276, "values"=u16[] [0]) -> (w1834:cluster{"starting address":u16, "values":u16[]})
                        n1095 = Enqueue Element(queue=w1832, element=w1834) -> ()  [unwired: 2 in, 3 out]
                        n1096 = local write "切换量程连续测两次"(TRUE ("切换量程连续测两次")) -> ()
                      }
                    }
                  }
                }
              }
            }
          }
          frame True {
            # "防止无限切量程"
            n1097 = local write "枚举"(enum16{"读取数据", "写入数据", "读取写入DATABASE", "读取参数"}."读取数据" ("枚举")) -> ()
            n1098 = local write "量程切换次数"(u8 0 ("量程切换次数")) -> ()
            n1099 = call "存数据cloumns(子VI).vi"() -> ("数组"=w1841:string[])  [unwired: 11 in]
            n1100 = global write "COD读取DATA全局.vi" "data"(w1839) -> ()
            n1101 = call "数据写入database.vi"("data"=w1839, "columns"=w1841, "table"="CODMn") -> ()  [unwired: 8 in, 1 out]
          }
        }
        n1102 = global read "COD测量模式全局.vi" "测量模式"() -> (w1712:string)
        n1103 = global write "COD浓度全局变量.vi" "COD浓度（mg/L)"(w1702) -> ()
        n1104 = Equal?(x=w1712, y="校标") -> (x = y?=w1710:bool)
        n1105 = case shown="真" w1710 {
          tunnel: w1719 -> [_ w1877]
          frame False {
          }
          frame True {
            n1106 = local read "当前校准"() -> (w1878:i32)
            n1107 = case shown="3" w1878 {
              tunnel: w1877 -> [w1879 w1880 w1881 w1882 w1883]
              frame 1, Default {
                n1108 = local write "泵滴定数1"(w1879) -> ()
              }
              frame 2 {
                n1109 = local write "泵滴定数2"(w1880) -> ()
              }
              frame 3 {
                n1110 = local write "泵滴定数3"(w1881) -> ()
              }
              frame 4 {
                n1111 = local write "泵滴定数4"(w1882) -> ()
              }
              frame 5 {
                n1112 = local write "泵滴定数5"(w1883) -> ()
              }
            }
          }
        }
      }
      frame "读取参数" {
        n1113 = Dequeue Element(queue=w1899, timeout in ms (-1)=1000 ("超时毫秒(-1)"), error in (no error)=w1898) -> (element=w1905:T5)  [unwired: 3 out]
        n1114 = local write "枚举"(enum16{"读取数据", "写入数据", "读取写入DATABASE", "读取参数"}."读取数据" ("枚举")) -> ()
        n1115 = Unbundle By Name(w1905) -> ("starting address"=w1904:u16, "number of holding registers"=w1903:u16)
        n1116 = local read "读取KB值"() -> (w1894:bool)
        n1117 = call <vilib>:"Read Holding Registers.vi"("error in (no error)"=w1900, "quantity"=w1903, "starting address"=w1904, "MB session in"=w1901) -> ("error out"=w1893:errorcluster, "Registers"=w1897:u16[], "MB session out"=w1895:refnum<class "MB_Master_Serial.lvclass">)  [unwired: 5 in]
        n1118 = case shown="假" w1894 {
          tunnel: w1897 -> [w1920 w1938]
          tunnel: w1893 -> [_ w1940]
          frame False {
            n1119 = Index Array(array=w1920) -> (element #1=w1917:u16, element #2=w1930:u16, element #3=w1910:u16, element #4=w1915:u16, element #5=w1913:u16, element #6=w1912:u16, element #7=w1929:u16, element #8=w1928:u16, element #9=w1927:u16, element #10=w1926:u16, element #11=w1925:u16, element #12=w1924:u16, element #13=w1923:u16, element #14=w1922:u16, element #15=w1921:u16, element #16=w1908:u16, element #17=w1907:u16, element #18=w1906:u16)  [unwired: 18 in]
            n1120 = local write "恒温时间"(w1930) -> ()
            n1121 = local write "基本量程"(w1913) -> ()
            n1122 = local write "水样"(w1912) -> ()
            n1123 = local write "蒸馏水"(w1929) -> ()
            n1124 = local write "标液"(w1928) -> ()
            n1125 = local write "质控样"(w1927) -> ()
            n1126 = local write "加标回收"(w1926) -> ()
            n1127 = local write "高锰酸钾"(w1925) -> ()
            n1128 = local write "草酸钠"(w1924) -> ()
            n1129 = local write "硫酸"(w1923) -> ()
            n1130 = local write "零点泵计量数 2"(w1922) -> ()
            n1131 = local write "标度泵计量数 2"(w1921) -> ()
            n1132 = Divide(x=w1917, y=u16 10) -> (x/y=w1918:dbl)
            n1133 = Divide(x=w1910, y=u16 100) -> (x/y=w1909:dbl)
            n1134 = Divide(x=w1915, y=u16 100) -> (x/y=w1914:dbl)
            n1135 = local write "高量程稀释倍数:"(w1908) -> ()
            n1136 = local write "低量程稀释倍数:"(w1907) -> ()
            n1137 = local write "CODMn零点核查选择"(w1906) -> ()
            n1138 = local write "温度"(w1918) -> ()
            n1139 = local write "标准液浓度"(w1909) -> ()
            n1140 = local write "修正系数"(w1914) -> ()
          }
          frame True {
            (unwired) 9 ("索引")
            n1141 = case shown="错误" w1940 {
              tunnel: ["读取成功" ("消息") "读取失败" ("消息")] -> w1939
              frame No Error {
              }
              frame Error {
              }
            }
            n1142 = Array Subset(array=w1938, index=10 ("索引"), length=84 ("长度")) -> (w1935:u16[])
            n1143 = call "浮点CDAB转换COD.vi"("数组"=w1935) -> ("数组 2"=w1934:sgl[])  [unwired: 10 in]
            n1144 = local read "测量模式(公式)"() -> (w1932:u16)
            n1145 = One Button Dialog(message=w1939) -> ()  [unwired: 1 in, 1 out]
            n1146 = Array To Cluster(array=w1934) -> (cluster=w1931:T18)
            n1147 = case shown="7" w1932 {
              tunnel: [cluster{"X":dbl, "b":dbl, "X^2":dbl} {"X"=999.0, "b"=999.0, "X^2"=999.0} ("方程系数") w1943 w1962 w1981 w2000 w2019 w2038 w2057] -> w1933
              tunnel: w1931 -> [_ w1942 w1961 w1980 w1999 w2018 w2037 w2056]
              frame 0, Default {
              }
              frame 1 {
                n1148 = local read "量程选择"() -> (w1945:enum16{"低量程", "高量程", "0-2量程"})
                n1149 = case shown="\"低量程\", 默认" w1945 {
                  tunnel: w1942 -> [w1952 w1956 w1960]
                  tunnel: [w1951 w1955 w1959] -> w1948
                  tunnel: [w1950 w1954 w1958] -> w1947
                  tunnel: [w1949 w1953 w1957] -> w1946
                  frame "低量程", Default {
                    n1150 = Unbundle By Name(w1952) -> ("数组 2[0]"=w1951:sgl, "数组 2[1]"=w1950:sgl, "数组 2[2]"=w1949:sgl)
                  }
                  frame "高量程" {
                    n1151 = Unbundle By Name(w1956) -> ("数组 2[3]"=w1955:sgl, "数组 2[4]"=w1954:sgl, "数组 2[5]"=w1953:sgl)
                  }
                  frame "0-2量程" {
                    n1152 = Unbundle By Name(w1960) -> ("数组 2[6]"=w1959:sgl, "数组 2[7]"=w1958:sgl, "数组 2[8]"=w1957:sgl)
                  }
                }
                n1153 = Bundle By Name(cluster=cluster{"X":dbl, "b":dbl, "X^2":dbl} {"X"=0.0, "b"=0.0, "X^2"=0.0} ("方程系数"), "X"=w1948, "b"=w1947, "X^2"=w1946) -> (w1943:cluster{"X":dbl, "b":dbl, "X^2":dbl})
              }
              frame 2 {
                n1154 = local read "量程选择"() -> (w1964:enum16{"低量程", "高量程", "0-2量程"})
                n1155 = case shown="\"高量程\"" w1964 {
                  tunnel: w1961 -> [w1971 w1975 w1979]
                  tunnel: [w1970 w1974 w1978] -> w1967
                  tunnel: [w1969 w1973 w1977] -> w1966
                  tunnel: [w1968 w1972 w1976] -> w1965
                  frame "低量程", Default {
                    n1156 = Unbundle By Name(w1971) -> ("数组 2[6]"=w1970:sgl, "数组 2[7]"=w1969:sgl, "数组 2[8]"=w1968:sgl)
                  }
                  frame "高量程" {
                    n1157 = Unbundle By Name(w1975) -> ("数组 2[9]"=w1974:sgl, "数组 2[10]"=w1973:sgl, "数组 2[11]"=w1972:sgl)
                  }
                  frame "0-2量程" {
                    n1158 = Unbundle By Name(w1979) -> ("数组 2[6]"=w1978:sgl, "数组 2[7]"=w1977:sgl, "数组 2[8]"=w1976:sgl)
                  }
                }
                n1159 = Bundle By Name(cluster=cluster{"X":dbl, "b":dbl, "X^2":dbl} {"X"=0.0, "b"=0.0, "X^2"=0.0} ("方程系数"), "X"=w1967, "b"=w1966, "X^2"=w1965) -> (w1962:cluster{"X":dbl, "b":dbl, "X^2":dbl})
              }
              frame 3 {
                n1160 = local read "量程选择"() -> (w1983:enum16{"低量程", "高量程", "0-2量程"})
                n1161 = case shown="\"高量程\"" w1983 {
                  tunnel: w1980 -> [w1990 w1994 w1998]
                  tunnel: [w1989 w1993 w1997] -> w1986
                  tunnel: [w1988 w1992 w1996] -> w1985
                  tunnel: [w1987 w1991 w1995] -> w1984
                  frame "低量程", Default {
                    n1162 = Unbundle By Name(w1990) -> ("数组 2[12]"=w1989:sgl, "数组 2[13]"=w1988:sgl, "数组 2[14]"=w1987:sgl)
                  }
                  frame "高量程" {
                    n1163 = Unbundle By Name(w1994) -> ("数组 2[15]"=w1993:sgl, "数组 2[16]"=w1992:sgl, "数组 2[17]"=w1991:sgl)
                  }
                  frame "0-2量程" {
                    n1164 = Unbundle By Name(w1998) -> ("数组 2[6]"=w1997:sgl, "数组 2[7]"=w1996:sgl, "数组 2[8]"=w1995:sgl)
                  }
                }
                n1165 = Bundle By Name(cluster=cluster{"X":dbl, "b":dbl, "X^2":dbl} {"X"=0.0, "b"=0.0, "X^2"=0.0} ("方程系数"), "X"=w1986, "b"=w1985, "X^2"=w1984) -> (w1981:cluster{"X":dbl, "b":dbl, "X^2":dbl})
              }
              frame 4 {
                n1166 = local read "量程选择"() -> (w2002:enum16{"低量程", "高量程", "0-2量程"})
                n1167 = case shown="\"高量程\"" w2002 {
                  tunnel: w1999 -> [w2009 w2013 w2017]
                  tunnel: [w2008 w2012 w2016] -> w2005
                  tunnel: [w2007 w2011 w2015] -> w2004
                  tunnel: [w2006 w2010 w2014] -> w2003
                  frame "低量程", Default {
                    n1168 = Unbundle By Name(w2009) -> ("数组 2[18]"=w2008:sgl, "数组 2[19]"=w2007:sgl, "数组 2[20]"=w2006:sgl)
                  }
                  frame "高量程" {
                    n1169 = Unbundle By Name(w2013) -> ("数组 2[21]"=w2012:sgl, "数组 2[22]"=w2011:sgl, "数组 2[23]"=w2010:sgl)
                  }
                  frame "0-2量程" {
                    n1170 = Unbundle By Name(w2017) -> ("数组 2[6]"=w2016:sgl, "数组 2[7]"=w2015:sgl, "数组 2[8]"=w2014:sgl)
                  }
                }
                n1171 = Bundle By Name(cluster=cluster{"X":dbl, "b":dbl, "X^2":dbl} {"X"=0.0, "b"=0.0, "X^2"=0.0} ("方程系数"), "X"=w2005, "b"=w2004, "X^2"=w2003) -> (w2000:cluster{"X":dbl, "b":dbl, "X^2":dbl})
              }
              frame 5 {
                n1172 = local read "量程选择"() -> (w2021:enum16{"低量程", "高量程", "0-2量程"})
                n1173 = case shown="\"高量程\"" w2021 {
                  tunnel: w2018 -> [w2028 w2032 w2036]
                  tunnel: [w2027 w2031 w2035] -> w2024
                  tunnel: [w2026 w2030 w2034] -> w2023
                  tunnel: [w2025 w2029 w2033] -> w2022
                  frame "低量程", Default {
                    n1174 = Unbundle By Name(w2028) -> ("数组 2[24]"=w2027:sgl, "数组 2[25]"=w2026:sgl, "数组 2[26]"=w2025:sgl)
                  }
                  frame "高量程" {
                    n1175 = Unbundle By Name(w2032) -> ("数组 2[27]"=w2031:sgl, "数组 2[28]"=w2030:sgl, "数组 2[29]"=w2029:sgl)
                  }
                  frame "0-2量程" {
                    n1176 = Unbundle By Name(w2036) -> ("数组 2[6]"=w2035:sgl, "数组 2[7]"=w2034:sgl, "数组 2[8]"=w2033:sgl)
                  }
                }
                n1177 = Bundle By Name(cluster=cluster{"X":dbl, "b":dbl, "X^2":dbl} {"X"=0.0, "b"=0.0, "X^2"=0.0} ("方程系数"), "X"=w2024, "b"=w2023, "X^2"=w2022) -> (w2019:cluster{"X":dbl, "b":dbl, "X^2":dbl})
              }
              frame 6 {
                n1178 = local read "量程选择"() -> (w2040:enum16{"低量程", "高量程", "0-2量程"})
                n1179 = case shown="\"高量程\"" w2040 {
                  tunnel: w2037 -> [w2047 w2051 w2055]
                  tunnel: [w2046 w2050 w2054] -> w2043
                  tunnel: [w2045 w2049 w2053] -> w2042
                  tunnel: [w2044 w2048 w2052] -> w2041
                  frame "低量程", Default {
                    n1180 = Unbundle By Name(w2047) -> ("数组 2[30]"=w2046:sgl, "数组 2[31]"=w2045:sgl, "数组 2[32]"=w2044:sgl)
                  }
                  frame "高量程" {
                    n1181 = Unbundle By Name(w2051) -> ("数组 2[33]"=w2050:sgl, "数组 2[34]"=w2049:sgl, "数组 2[35]"=w2048:sgl)
                  }
                  frame "0-2量程" {
                    n1182 = Unbundle By Name(w2055) -> ("数组 2[6]"=w2054:sgl, "数组 2[7]"=w2053:sgl, "数组 2[8]"=w2052:sgl)
                  }
                }
                n1183 = Bundle By Name(cluster=cluster{"X":dbl, "b":dbl, "X^2":dbl} {"X"=0.0, "b"=0.0, "X^2"=0.0} ("方程系数"), "X"=w2043, "b"=w2042, "X^2"=w2041) -> (w2038:cluster{"X":dbl, "b":dbl, "X^2":dbl})
              }
              frame 7 {
                n1184 = local read "量程选择"() -> (w2059:enum16{"低量程", "高量程", "0-2量程"})
                n1185 = case shown="\"高量程\"" w2059 {
                  tunnel: w2056 -> [w2066 w2070 w2074]
                  tunnel: [w2065 w2069 w2073] -> w2062
                  tunnel: [w2064 w2068 w2072] -> w2061
                  tunnel: [w2063 w2067 w2071] -> w2060
                  frame "低量程", Default {
                    n1186 = Unbundle By Name(w2066) -> ("数组 2[36]"=w2065:sgl, "数组 2[37]"=w2064:sgl, "数组 2[38]"=w2063:sgl)
                  }
                  frame "高量程" {
                    n1187 = Unbundle By Name(w2070) -> ("数组 2[39]"=w2069:sgl, "数组 2[40]"=w2068:sgl, "数组 2[41]"=w2067:sgl)
                  }
                  frame "0-2量程" {
                    n1188 = Unbundle By Name(w2074) -> ("数组 2[6]"=w2073:sgl, "数组 2[7]"=w2072:sgl, "数组 2[8]"=w2071:sgl)
                  }
                }
                n1189 = Bundle By Name(cluster=cluster{"X":dbl, "b":dbl, "X^2":dbl} {"X"=0.0, "b"=0.0, "X^2"=0.0} ("方程系数"), "X"=w2062, "b"=w2061, "X^2"=w2060) -> (w2057:cluster{"X":dbl, "b":dbl, "X^2":dbl})
              }
            }
            n1190 = local write "方程系数"(w1933) -> ()
          }
        }
      }
    }
    n1191 = Unbundle By Name(w1580) -> ("status"=w1581:bool)
    n1192 = Not(x=w1581) -> (.not. x?=→"通讯状态":bool)
  }
  n1193 = call-dynamic "Close Session.vi"("error in (no error)"=w30, "MB_Serial session"=w29) -> ()  [unwired: 9 in, 1 out]
  "COM" <- "VISA resource name"
